vi "Data Analysis.vi"(1 "Data IN":T1={"Impulse Positions"=[], "No. Imp"=0, "Parameter Time Series"=[], "Parameter Impuls Series"=[], "Experiment Parameters"={"Freq"=0.0, "Vel"=0, "Acc"=0, "Stimulus"=""}, "Autosort File"=refnum, "Data File"={"Data Channels"=[], "Sample Rate"=0, "Channel List"=[]}, "Experiment data path"=path "/Macintosh HD/Users/patrick/Studium/Diploma Thesis/Data Analysis", "Image data path"=path "/Macintosh HD/Users/patrick/Studium/Diploma Thesis/Data Analysis", "LVS data path"=path "/Macintosh HD/Users/patrick/Studium/Diploma Thesis/Data Analysis", "Raw copy path"=path "/Macintosh HD/Users/patrick/Studium/Diploma Thesis/Data Analysis", "filename"="No file selected", "desaccading parameters"={"Tolerance"=0, "Acc Range"=0.0, "Sample Rate"=0, "Impulse Plane 2"=enum."Other", "Impulse dir"=FALSE}, "Experiment Parameters 2"={"Subject"="", "Strain"="", "Rotation plane"="", "Experimenter"="", "Trial"=0.0, "Time"=0.0}, "Excel"={"Excel._Application"=refnum, "Use Excel"=FALSE, "Worksheet SINE"=refnum, "Row SINE"=0, "Worksheet TRANS"=refnum, "Row TRANS"=0}, "Session Config File"=refnum, "Autosort Parameter Set"=1, "EMA Version"="", "desacc "={"Threshold 1 [Acc]"=1617.080808080808, "Threshold 2 [% of TH1]"=67, "tolerance"=5, "Search WD "=0.19090909090909092, " always use TH2"=TRUE, "Range"=3.2323232323232323, "Max time"=200.0, "Min time"=20.0, "Velocity Threshold"=67}, "Cycle Nr for Saccades"={"POS"=0, "NEG"=0}, "calibration name"="No file selected", "Excel"=refnum} {"Parameter Time Series"."time offset" format="%.3f"; "Parameter Time Series"."Gain" format="%.1f"; "Parameter Time Series"."Offset" format="%.1f"; "Parameter Time Series"."List 1" items=["Motor-Pos", "Motor-Vel", "Lx Position-in-Head", "Ly Position-in-Head", "Lz Position-in-Head", "Lx Velocity-in-Head", "Ly Velocity-in-Head", "Lz Velocity-in-Head", "Ll Velocity-in-Head", "Lr Velocity-in-Head", "Lx Accel-in-Head", "Ly Accel-in-Head", "Lz Accel-in-Head", "Rx Position-in-Head", "Ry Position-in-Head", "Rz Position-in-Head", "Rx Velocity-in-Head", "Ry Velocity-in-Head", "Rz Velocity-in-Head", "Rl Velocity-in-Head", "Rr Velocity-in-Head", "Rx Accel-in-Head", "Ry Accel-in-Head", "Rz Accel-in-Head", "Global Trigger", "", "", ""]; "Parameter Impuls Series"."Gain" format="%.1f"; "Parameter Impuls Series"."Offset" format="%.1f"}, 9 "Trace Select":i32 min=0 max=1000, 11 "Interpolate":bool) -> (3 "Data OUT":T1={"Impulse Positions"=[], "No. Imp"=0, "Parameter Time Series"=[], "Parameter Impuls Series"=[], "Experiment Parameters"={"Freq"=0.0, "Vel"=0, "Acc"=0, "Stimulus"=""}, "Autosort File"=refnum, "Data File"={"Data Channels"=[], "Sample Rate"=0, "Channel List"=[]}, "Experiment data path"=path "/Macintosh HD/Users/patrick/Studium/Diploma Thesis/Data Analysis", "Image data path"=path "/Macintosh HD/Users/patrick/Studium/Diploma Thesis/Data Analysis", "LVS data path"=path "/Macintosh HD/Users/patrick/Studium/Diploma Thesis/Data Analysis", "Raw copy path"=path "/Macintosh HD/Users/patrick/Studium/Diploma Thesis/Data Analysis", "filename"="No file selected", "desaccading parameters"={"Tolerance"=0, "Acc Range"=0.0, "Sample Rate"=0, "Impulse Plane 2"=enum."Other", "Impulse dir"=FALSE}, "Experiment Parameters 2"={"Subject"="", "Strain"="", "Rotation plane"="", "Experimenter"="", "Trial"=0.0, "Time"=0.0}, "Excel"={"Excel._Application"=refnum, "Use Excel"=FALSE, "Worksheet SINE"=refnum, "Row SINE"=0, "Worksheet TRANS"=refnum, "Row TRANS"=0}, "Session Config File"=refnum, "Autosort Parameter Set"=1, "EMA Version"="", "desacc "={"Threshold 1 [Acc]"=1617.080808080808, "Threshold 2 [% of TH1]"=67, "tolerance"=5, "Search WD "=0.19090909090909092, " always use TH2"=TRUE, "Range"=3.2323232323232323, "Max time"=200.0, "Min time"=20.0, "Velocity Threshold"=67}, "Cycle Nr for Saccades"={"POS"=0, "NEG"=0}, "calibration name"="No file selected", "Excel"=refnum} {"Parameter Time Series"."time offset" format="%.3f"; "Parameter Time Series"."Gain" format="%.1f"; "Parameter Time Series"."Offset" format="%.1f"; "Parameter Time Series"."List 1" items=["Motor-Pos", "Motor-Vel", "Lx Position-in-Head", "Ly Position-in-Head", "Lz Position-in-Head", "Lx Velocity-in-Head", "Ly Velocity-in-Head", "Lz Velocity-in-Head", "Ll Velocity-in-Head", "Lr Velocity-in-Head", "Lx Accel-in-Head", "Ly Accel-in-Head", "Lz Accel-in-Head", "Rx Position-in-Head", "Ry Position-in-Head", "Rz Position-in-Head", "Rx Velocity-in-Head", "Ry Velocity-in-Head", "Rz Velocity-in-Head", "Rl Velocity-in-Head", "Rr Velocity-in-Head", "Rx Accel-in-Head", "Ry Accel-in-Head", "Rz Accel-in-Head", "Global Trigger", "", "", ""]; "Parameter Impuls Series"."Gain" format="%.1f"; "Parameter Impuls Series"."Offset" format="%.1f"})   [LabVIEW 2016]
uses:
  Typedef - Sinusoidal Fit Controls.ctl
  Typedef - Sinusoidal Fit Coefficients.ctl
  Typedef_StatisticType.ctl
  Typedef - Gain and Phase.ctl
  core/type-defs/TD_Statemachine-Data.ctl
  <userlib>/Import Export/Excel/Excel.lvclass
  core/type-defs/TD_Time Series.ctl
  core/type-defs/TD_Impulse Parameter.ctl
  Typedef - Type of Analysis.ctl
  core/Classes/Exponential Fit/Exponential Fit Parameters.ctl
  core/Classes/Head Impulse Fit/Fit Data.ctl
  core/Classes/Head Impulse Fit/Fit Controls.ctl
  Data Analysis state.ctl
  Typedef - Data Analyser Main Cluster.ctl
  core/Classes/Impulse Data/Instance handle.ctl
  core/Classes/Impulse Data/Impulse Data.lvclass
  core/Classes/Impulse Manager/Impulse Manager.lvclass
  core/Classes/Graph Manager/Graph Manager.lvclass
  core/Classes/Sinusoidal Fit/Sinusoidal Fit.lvclass
  C:/Users/w.figtree/Desktop/Work/4. Projects/3. In Progress Engineering Projects/EMA/src/core/Classes/Abstract Fit/Abstract Fit.lvclass
  core/Classes/Excel Logger/Excel Logger.lvclass
  core/Classes/Fit Displays/Halfwave Fit Display/Halfwave Fit Display.lvclass
  core/Classes/Mean Fit/Mean Fit.lvclass
  core/Classes/Exponential Fit/Exponential Fit.lvclass
  core/Classes/Head Impulse Fit/Head Impulse Fit.lvclass
  core/Classes/Desaccade Manipulator/Desaccade Manipulator.lvclass
  core/Classes/Excel Logger/Excel Logger.lvclass/Excel Logger.ctl
  core/type-defs/TD_Impulse Planes.ctl
  core/Classes/Abstract Fit/Abstract Fit.lvclass/Abstract Fit.ctl
  core/Classes/Sinusoidal Fit/Sinusoidal Fit.lvclass/Sinusoidal Fit.ctl
  <vilib>/Analysis/baseanly.llb/Mean (DBL).vi
  core/Classes/Data Analyser Report/Data Analyser Report.lvclass
  C:/Users/w.figtree/Desktop/Work/4. Projects/3. In Progress Engineering Projects/EMA/src/core/Classes/Excel Interface/Excel Sheet/Excel Sheet.lvclass
  core/Classes/Sinusoidal Fit/Halfwave Sinusoidal Fit/Halfwave Sinusoidal Fit.lvclass
  C:/Users/w.figtree/Desktop/Work/4. Projects/3. In Progress Engineering Projects/EMA/src/core/Classes/Sinusoidal Fit/Sinusoidal Fit.lvclass
  core/Classes/Excel Interface/Excel Sheet/Write to Cell - String.vi
  core/Classes/Excel Interface/Excel Sheet/Write to Cell - Int.vi
  core/Classes/Excel Interface/Excel Sheet/Write to Cell - Dbl.vi
  <userlib>/_OpenG.lib/array/array.llb/Remove Duplicates from 1D Array (I32)__ogtk.vi
  comm/impulse/impulse functions.lvlib
  comm/nan operations/nan operations.lvlib
  comm/stats/stats.lvlib
  <vilib>/Analysis/NI_AALPro.lvlib
  comm/excel/excel.lvlib
  <vilib>/Analysis/NI_AALBase.lvlib
  core/core.lvlib
  core/Classes/Excel Interface/Excel Sheet/Excel Sheet.lvclass
  core/Classes/Abstract Fit/Abstract Fit.lvclass
panel:
  out "Impulse Trace":cluster{dbl, dbl, "Impulses":dbl[][]}(graph)
  in  "Response":dbl[](array[numeric]) format="%.2f"
  in  "Stimulus":dbl[](array[numeric]) format="%.2f"
  in  "Reset view":bool
  in  "Show Fit":bool=TRUE
  in  "Mean Traces":bool=TRUE
  in  "Fixed Time":bool
  in  "Fixed Amplitude":bool
  in  "Interpolate 3":bool
  in  "Interpolate 2":bool
  in  "Gv Line Fit Response":cluster{"Offset":dbl, "Slope":dbl}={"Offset"=186.60289859552654, "Slope"=-3505.824046527282} {"Slope" format="%.2f"; "Offset" format="%.2f"}
  in  "Gv Line Fit Stimulus":cluster{"Offset":dbl, "Slope":dbl}={"Offset"=195.7972297018837, "Slope"=-3976.499768980883} {"Slope" format="%.2f"; "Offset" format="%.2f"}
  in  "Fitted Curves":dbl[][](array[numeric]) format="%.2f"
  in  "Tab Control":T4(tab)
  in  "Sinusoidal Fit Controls":T5={"Sinusoidal Response"={"Offset"=-0.14811303182601265, "Gain"=36.1562775012231, "Phase"=51.14206032808873, "Freq"=8.0}, "Sinusoidal Stimulus"={"Offset"=-0.1762531244084861, "Gain"=54.01231242273056, "Phase"=48.997269246957444, "Freq"=8.0}, "Stimulus\nFrequency"=8.0, "Stat."=enum."Ind. Traces", "Use Values Above to Calculate Gains"=FALSE, "Automatically Calculate \nStimulus Frequency"=FALSE, "Gain and Phase"={"Gain"=0.0, "Gain SD"=0.0, "Phase"=0.0, "Phase SD"=0.0}} {"Gain and Phase"."Phase SD" format="%.1f"; "Gain and Phase"."Phase" format="%.1f"; "Gain and Phase"."Gain SD" format="%.2f"; "Gain and Phase"."Gain" format="%.2f"; "Stimulus\nFrequency" format="%.2f"; "Sinusoidal Stimulus"."Freq" format="%#.2f"; "Sinusoidal Stimulus"."Offset" format="%.3f"; "Sinusoidal Stimulus"."Gain" format="%.2f"; "Sinusoidal Stimulus"."Phase" format="%.1f"; "Sinusoidal Response"."Freq" format="%#.2f"; "Sinusoidal Response"."Offset" format="%.3f"; "Sinusoidal Response"."Gain" format="%.2f"; "Sinusoidal Response"."Phase" format="%.1f"}
  in  "Transient Gains":T9={"Line Fit Response"={"Offset"=186.60289859552654, "Slope"=-3505.824046527282}, "Stimulus Equation"="195.80  + -3976.50 t ", "Reponse Equation"="186.60  + -3505.82 t ", "Gv"=-0.4707337082056428, "Ga"=0.8816409948711299, "Line Fit Stimulus"={"Offset"=195.7972297018837, "Slope"=-3976.499768980883}, "Ga Window (early)"=0, "Gv Window"=1, "Latency (ms)"=3.987957239637936, "Stim.Onset"=49.23858696766971, "TH/#SDs 2"=10.0, "Response Onset"=53.22654420730765, "Snap Cursor"=1, "Latency"=2, "Poly. Window"=1, "Ord."=3, "BIC"=3.7869704994038274, "Poly Equation"="124.42 t^0 + -1322.54 t^1 + -147215.26 t^2 + 1663449.30 t^3", "Gv SD"=1.2509198071254501, "Ga SD"=0.09245681991197086, "Ga Stat."=0, "Mirror"=FALSE, "MSE"=3.7869704994038274, "Gv Stat."=2, "Ga 2"=0.8816409948711299, "Ga SD 2"=0.09245681991197086, "Ga Window  (late)"=5, "Ga Stat. 2"=0, "GV desaccading"=TRUE, "GA2 desaccading"=FALSE, "GA1 desaccading"=FALSE, "Line Fit Response 2"={"Offset"=186.60289859552654, "Slope"=-3505.824046527282}, "Stimulus Equation 2"="195.80  + -3976.50 t ", "Reponse Equation 2"="186.60  + -3505.82 t ", "Line Fit Stimulus 2"={"Offset"=195.7972297018837, "Slope"=-3976.499768980883}, "Show Line Fit Parameters "=FALSE, "Gv Line Fit Stimulus"={"Offset"=195.7972297018837, "Slope"=-3976.499768980883}, "Gv Line Fit Response"={"Offset"=186.60289859552654, "Slope"=-3505.824046527282}, "Latency window"=0, "Latency Stat."=0, "Line Fit Res Latency"={"Offset"=186.60289859552654, "Slope"=-3505.824046527282}, "Stim Eq Latency"="195.80  + -3976.50 t ", "Resp Eq Latency"="186.60  + -3505.82 t ", "Line Fit Stim Latency"={"Offset"=195.7972297018837, "Slope"=-3976.499768980883}, "GA Line active"=0} {"Line Fit Stim Latency"."Slope" format="%.2f"; "Line Fit Stim Latency"."Offset" format="%.2f"; "Line Fit Res Latency"."Slope" format="%.2f"; "Line Fit Res Latency"."Offset" format="%.2f"; "Latency Stat." items=["Mean Trace", "Ind. Traces", "Pnt. by Pnt.", "Inst. Slope"]; "Latency window" items=["Cursor", "10 - 20 ms", "20 - 30 ms", "30 - 40 ms", "40 - 50 ms", "20 - 40 ms", "10 - 30 ms"]; "Latency" items=["Standard Dev.", "Threshold", "Line Intercept"]; "TH/#SDs 2" format="%.2f"; "Stim.Onset" format="%.2f"; "Latency (ms)" format="%.2f"; "MSE" format="%.4f"; "BIC" format="%.2f"; "Poly. Window" items=["Cursor", "10 - 40 ms", "5 - 35 ms", "0 - 30 ms"]; "Ga Stat." items=["Mean Trace", "Ind. Traces", "Pnt. by Pnt.", "Inst. Slope"]; "Ga SD" format="%.2f"; "Ga Window (early)" items=["Cursor", "10 - 20 ms", "20 - 30 ms", "30 - 40 ms", "40 - 50 ms", "20 - 40 ms", "10 - 30 ms"]; "Ga" format="%.2f"; "Ga Stat. 2" items=["Mean Trace", "Ind. Traces", "Pnt. by Pnt.", "Inst. Slope"]; "Ga Window  (late)" items=["Cursor", "10 - 20 ms", "20 - 30 ms", "30 - 40 ms", "40 - 50 ms", "20 - 40 ms", "10 - 30 ms"]; "Ga SD 2" format="%.2f"; "Ga 2" format="%.2f"; "Gv Stat." items=["Mean Trace", "Ind. Traces", "Pnt. by Pnt.", "Inst. Slope"]; "Gv SD" format="%.2f"; "Gv Window" items=["Cursor", "200 - 400ms", "200 - 700ms"]; "Gv" format="%.2f"; "Snap Cursor" items=["No Snap", "to Ga (early)", "to Ga (late)", "to Gv", "Latency"]; "Gv Line Fit Response"."Slope" format="%.2f"; "Gv Line Fit Response"."Offset" format="%.2f"; "Gv Line Fit Stimulus"."Slope" format="%.2f"; "Gv Line Fit Stimulus"."Offset" format="%.2f"; "Line Fit Stimulus 2"."Slope" format="%.2f"; "Line Fit Stimulus 2"."Offset" format="%.2f"; "Line Fit Response 2"."Slope" format="%.2f"; "Line Fit Response 2"."Offset" format="%.2f"; "Response Onset" format="%.2f"; "Line Fit Stimulus"."Slope" format="%.2f"; "Line Fit Stimulus"."Offset" format="%.2f"; "Line Fit Response"."Slope" format="%.2f"; "Line Fit Response"."Offset" format="%.2f"}
  in  "Tab Control 2":enum32{"Page 1", "Page 2"}(tab)
  in  "Save All G&P To Excel":bool
  out "Normal Sine - Gain and Phase":T8 caption="Gain and Phase" {"Phase SD" format="%.1f"; "Phase" format="%.1f"; "Gain SD" format="%.2f"; "Gain" format="%.2f"}
  out "Normal Sine - Stimulus":T6 caption="Stimulus" {"Freq" format="%#.2f"; "Offset" format="%.3f"; "Gain" format="%.2f"; "Phase" format="%.1f"}
  in  "Normal Sine - Response":T6 caption="Response" {"Freq" format="%#.2f"; "Offset" format="%.3f"; "Gain" format="%.2f"; "Phase" format="%.1f"}
  out "Positive Halfwave":T8 {"Phase SD" format="%.1f"; "Phase" format="%.1f"; "Gain SD" format="%.2f"; "Gain" format="%.2f"}
  out "Negative Halfwave":T8 {"Phase SD" format="%.1f"; "Phase" format="%.1f"; "Gain SD" format="%.2f"; "Gain" format="%.2f"}
  out "Coefficients":T6 {"Freq" format="%#.2f"; "Offset" format="%.3f"; "Gain" format="%.2f"; "Phase" format="%.1f"}
  in  "Pos HW Response":T6 caption="Response" {"Freq" format="%#.2f"; "Offset" format="%.3f"; "Gain" format="%.2f"; "Phase" format="%.1f"}
  out "Coefficients 2":T6 {"Freq" format="%#.2f"; "Offset" format="%.3f"; "Gain" format="%.2f"; "Phase" format="%.1f"}
  in  "Neg HW Response":T6 {"Freq" format="%#.2f"; "Offset" format="%.3f"; "Gain" format="%.2f"; "Phase" format="%.1f"}
  in  "Auto Calc.":bool
  in  "Stimulus\nFrequency":dbl=8.0 format="%.2f"
  in  "Sine Fit Type":enum16{"Normal Fit", "Halfwave Fit"}(ring)
  in  "Stat. Method":T7=enum."Ind. Traces"
  in  "Offset":dbl format="%#_13g"
  in  "Mean Stats Method":T7=enum."Ind. Traces" caption="Statistics Method"
  out "Mean Fit":T10
  in  "Exp Response":T11 caption="Response Fit Parameters"
  in  "Exp Stimulus":T11 caption="Stimulus Fit Parameters"
  in  "Head Impulse Fit Controls":T12={"Pre-peak-ms"=30.0, "Onset threshold (%)"=4.0, "Window size (+- ms)"=10.0, "Window Centres\n(ms after onset)"=[40.0, 60.0, 80.0]}
  out "Head Impulse Fit Data":T13 {"Window Eye Lag (ms)" format="%#_4g"; "Window Gain" format="%#_4g"}
  in  "btn_SaveImpulseLatency":bool
  out "Impulse Latency Summary":T14
  in  "Impulse Latency Controls":T15={"Peak%"=4.0, "Min Valid Latency"=-50.0, "Max Valid Latency"=50.0, "Only After\nCursor?"=TRUE}
  out "Impulse Latency Results":dbl[][](array[numeric])
  in  "Excel Cell Handling":enum16{"Active Cell", "First empty cell (Ax)"}(ring)=enum."First empty cell (Ax)"
  in  "Freeze Visibility On Channel Cycle":bool
  in  "Auto Channel Cycle":bool
  in  "Prefer Mean Fit":bool
  in  "Limit Phase to 180 degrees (negative gains!)":bool
  in  "Hide Grid":bool
  in  "Hide Cursors":bool
  in  "Parameters":T16={"Vel Range"=10.0, "Acc Range"=500.0, "Stimulus Freq"=4.0, "Impulse Plane"=enum."Other", "Impulse Direction"=TRUE} {"Stimulus Freq" step=0.5 format="%.2f"; "Acc Range" format="%.2f"; "Vel Range" format="%.2f"}
  in  "Line Range +/- GV":dbl=0.2
  in  "Line Range +/- GA":dbl=0.06
  in  "Spline Parameter":dbl=0.999
  in  "Spline":bool
  in  "Type of Analysis":T17
  in  "Save 2 Excel":bool
  in  "Save":bool
  in  "Analyse Data":bool
  in  "Impulse Direction":bool=TRUE
  in  "Cycle  Channel":bool
  in  "Parameter Impuls Series":T3=[{"Color"=4652800, "Visible"=TRUE, "Channel"=5, "Invert"=FALSE, "Desaccade"=FALSE, "Offset"=0.0, "Gain"=1.0}, {"Color"=16860, "Visible"=TRUE, "Channel"=13, "Invert"=FALSE, "Desaccade"=FALSE, "Offset"=0.0, "Gain"=1.0}, {"Color"=16711680, "Visible"=TRUE, "Channel"=21, "Invert"=FALSE, "Desaccade"=FALSE, "Offset"=0.0, "Gain"=1.0}] {"Gain" format="%.1f"; "Offset" format="%.1f"; "Channel" items=["-", "Hz Velocity-in-Head", "-", "Hy Velocity-in-Head", "-", "Hx Velocity-in-Head", "Hl Velocity-in-Head", "Hr Velocity-in-Head", "-", "Ly Position-in-Head", "Lz Position-in-Head", "-", "Ly Velocity-in-Head", "Lz Velocity-in-Head", "-", "Hx Acceleration-in-Head", "Hy Acceleration-in-Head", "Hz Acceleration-in-Head", "Hl Acceleration-in-Head", "Hr Acceleration-in-Head", "-", "Ly Acceleration-in-Head", "Lz Acceleration-in-Head", "-"]}
  in  "Generate New Plot":bool
  # "Gain:"
  # "+/-"
  # "Phase:"
  # "+/-"
  # "Latency"
  # "Polynomial Fit"
  # "Regression Fit"
  # "Desacc."
  # "Gain:"
  # "+/-"
  # "Phase:"
  # "+/-"
  # "Gain:"
  # "+/-"
  # "Phase:"
  # "+/-"
  # "Gain:"
  # "+/-"
  # "Phase:"
  # "+/-"
  # "Fit Controls"
  # "Stimulus"
  # "Response"
  # "EXPERIMENTAL - DO NOT USE"
  # "NOTE: Response must be inverted!"
  # "Desaccading Parameters"
  # "Pos"
  # "Neg"
  # "Latency, Gain and Phase Detector \nver 3.0\nAmerico A. Migliaccio and Patrick P. Huebner\n13th May 2010"
  # "Analysis"
  # "Offset      Gain    Inv                    Channel                      Col   Vis   Sac"
  # "Stimulus"
  # "Response"
  # "Additional\n|\n\\/"
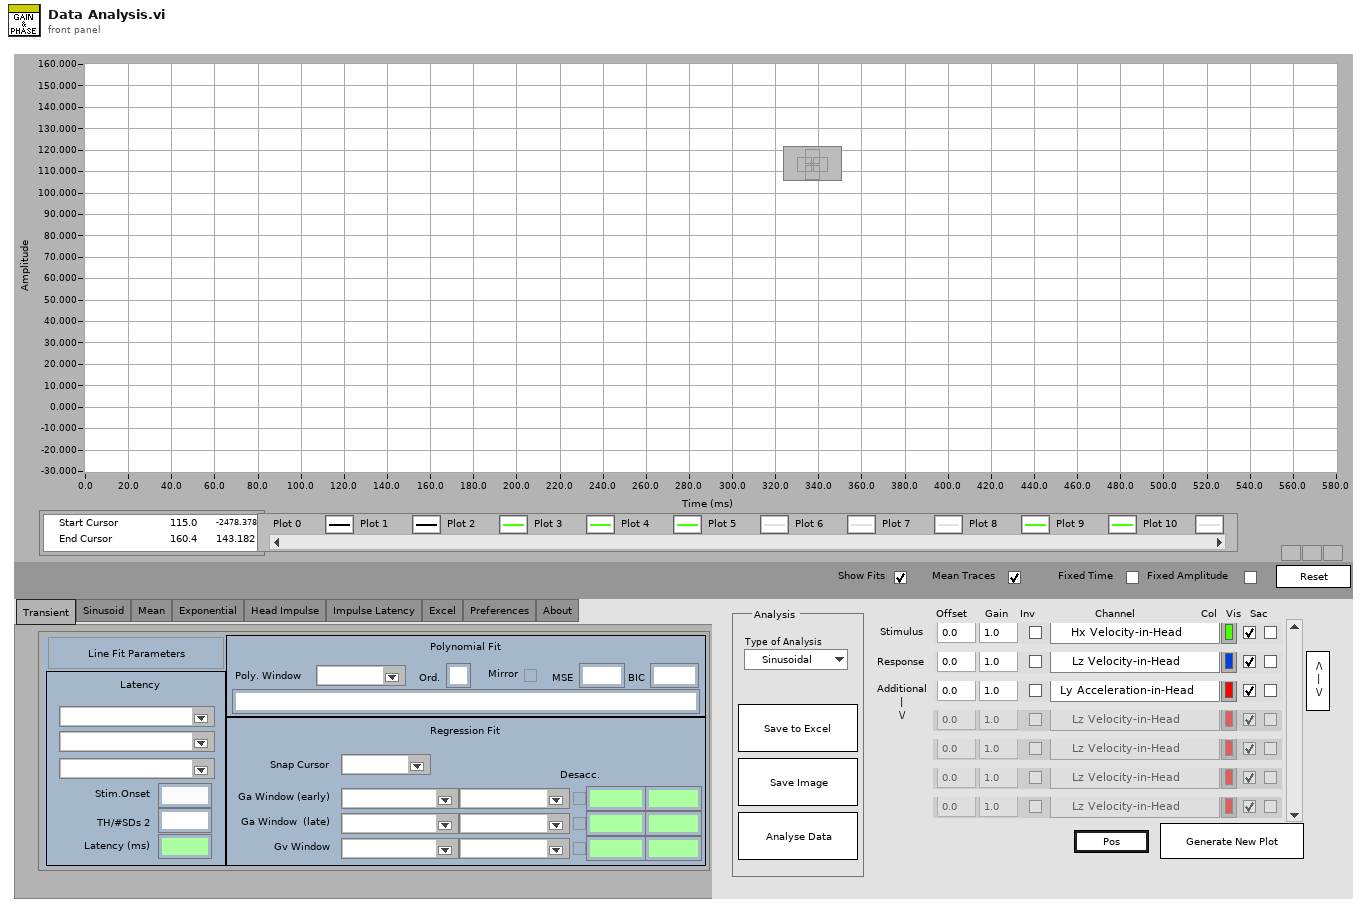
[diagram p1: front panel]
types:
  T1 = typedef "core.lvlib/TD_Statemachine-Data.ctl" = cluster{"Impulse Positions":cluster{"Start":i32, "End":i32, "Impulse Plane":enum16{"Other", "Yaw", "Pitch", "Roll", "LARP", "RALP"}, "Impulse Direction +ve?":bool, "Time offset":i32, "Amplitude offset":dbl}[], "No. Imp":i32, "Parameter Time Series":T2, "Parameter Impuls Series":T3, "Experiment Parameters":cluster{"Freq":dbl, "Vel":i32, "Acc":i32, "Stimulus":string}, "Autosort File":refnum<file>, "Data File":cluster{"Data Channels":dbl[][], "Sample Rate":i32, "Channel List":string[]}, "Experiment data path":path, "Image data path":path, "LVS data path":path, "Raw copy path":path, "filename":string, "desaccading parameters":cluster{"Tolerance":i32, "Acc Range":dbl, "Sample Rate":i32, "Impulse Plane 2":enum16{"Other", "Yaw", "Pitch", "Roll", "LARP", "RALP"}, "Impulse dir":bool}, "Experiment Parameters 2":cluster{"Subject":string, "Strain":string, "Rotation plane":string, "Experimenter":string, "Trial":dbl, "Time":dbl}, "Excel":cluster{"Excel._Application":refnum<k7>, "Use Excel":bool, "Worksheet SINE":refnum<k7>, "Row SINE":i32, "Worksheet TRANS":refnum<k7>, "Row TRANS":i32}, "Session Config File":refnum<file>, "Autosort Parameter Set":i32, "EMA Version":string, "desacc ":cluster{"Threshold 1 [Acc]":dbl, "Threshold 2 [% of TH1]":i32, "tolerance":i32, "Search WD ":dbl, " always use TH2":bool, "Range":dbl, "Max time":dbl, "Min time":dbl, "Velocity Threshold":i32}, "Cycle Nr for Saccades":cluster{"POS":i32, "NEG":i32}, "calibration name":string, "Excel":refnum<class "Excel.lvclass">}
  T2 = typedef "core.lvlib/TD_Time Series.ctl" = cluster{"time offset":dbl, "Offset":dbl, "Gain":dbl, "inverse":bool, "filter data":bool, "dots":bool, "interpolate":bool, "List 1":u16, "Color Box":u32, "Boolean":bool}[]
  T3 = typedef "core.lvlib/TD_Impulse Parameter.ctl" = cluster{"Color":u32, "Visible":bool, "Channel":u16, "Invert":bool, "Desaccade":bool, "Offset":dbl, "Gain":dbl}[]
  T4 = enum32{"Transient", "Sinusoid", "Mean", "Exponential", "Head Impulse", "Impulse Latency", "Excel", "Preferences", "About"}
  T5 = typedef "Typedef - Sinusoidal Fit Controls.ctl" = cluster{"Sinusoidal Response":T6, "Sinusoidal Stimulus":T6, "Stimulus\nFrequency":dbl, "Stat.":T7, "Use Values Above to Calculate Gains":bool, "Automatically Calculate \nStimulus Frequency":bool, "Gain and Phase":T8}
  T6 = typedef "Typedef - Sinusoidal Fit Coefficients.ctl" = cluster{"Offset":dbl, "Gain":dbl, "Phase":dbl, "Freq":dbl}
  T7 = typedef "Typedef_StatisticType.ctl" = enum16{"Mean Trace", "Ind. Traces"}
  T8 = typedef "Typedef - Gain and Phase.ctl" = cluster{"Gain":dbl, "Gain SD":dbl, "Phase":dbl, "Phase SD":dbl}
  T9 = cluster{"Line Fit Response":cluster{"Offset":dbl, "Slope":dbl}, "Stimulus Equation":string, "Reponse Equation":string, "Gv":dbl, "Ga":dbl, "Line Fit Stimulus":cluster{"Offset":dbl, "Slope":dbl}, "Ga Window (early)":u16, "Gv Window":u16, "Latency (ms)":dbl, "Stim.Onset":dbl, "TH/#SDs 2":dbl, "Response Onset":dbl, "Snap Cursor":u16, "Latency":u16, "Poly. Window":u16, "Ord.":i32, "BIC":dbl, "Poly Equation":string, "Gv SD":dbl, "Ga SD":dbl, "Ga Stat.":u16, "Mirror":bool, "MSE":dbl, "Gv Stat.":u16, "Ga 2":dbl, "Ga SD 2":dbl, "Ga Window  (late)":u16, "Ga Stat. 2":u16, "GV desaccading":bool, "GA2 desaccading":bool, "GA1 desaccading":bool, "Line Fit Response 2":cluster{"Offset":dbl, "Slope":dbl}, "Stimulus Equation 2":string, "Reponse Equation 2":string, "Line Fit Stimulus 2":cluster{"Offset":dbl, "Slope":dbl}, "Show Line Fit Parameters ":bool, "Gv Line Fit Stimulus":cluster{"Offset":dbl, "Slope":dbl}, "Gv Line Fit Response":cluster{"Offset":dbl, "Slope":dbl}, "Latency window":u16, "Latency Stat.":u16, "Line Fit Res Latency":cluster{"Offset":dbl, "Slope":dbl}, "Stim Eq Latency":string, "Resp Eq Latency":string, "Line Fit Stim Latency":cluster{"Offset":dbl, "Slope":dbl}, "GA Line active":i32}
  T10 = cluster{"Respopnse Mean":dbl, "Response SD":dbl, "Stimulus Mean":dbl, "Stimulus SD":dbl}
  T11 = typedef "Exponential Fit.lvclass/Exponential Fit Parameters.ctl" = cluster{"Amplitude":dbl, "Duration":dbl, "Time Constant":dbl, "Offset":dbl}
  T12 = typedef "Head Impulse Fit.lvclass/Fit Controls.ctl" = cluster{"Pre-peak-ms":dbl, "Onset threshold (%)":dbl, "Window size (+- ms)":dbl, "Window Centres\n(ms after onset)":dbl[]}
  T13 = typedef "Head Impulse Fit.lvclass/Fit Data.ctl" = cluster{"Peak time (ms)":dbl, "Peak val":dbl, "Gain":dbl, "Gain SD":dbl, "Peak-Peak lag (ms)":dbl, "Peak-Peak lag SD":dbl, "Window Gain":dbl[][], "Window Eye Lag (ms)":dbl[][]}
  T14 = cluster{"Stimulus Onset (ms)":dbl, "Response Onset (ms)":dbl, "Latency (ms)":dbl, "Num Impulses":dbl}
  T15 = cluster{"Peak%":dbl, "Min Valid Latency":dbl, "Max Valid Latency":dbl, "Only After\nCursor?":bool}
  T16 = cluster{"Vel Range":dbl, "Acc Range":dbl, "Stimulus Freq":dbl, "Impulse Plane":enum16{"Other", "Yaw", "Pitch", "Roll", "LARP", "RALP"}, "Impulse Direction":bool}
  T17 = typedef "Typedef - Type of Analysis.ctl" = enum16{"Sinusoidal", "Transient", "Mean", "Exponential", "Head Impulse", "Impulse Latency"}
  T18 = typedef "Typedef - Data Analyser Main Cluster.ctl" = cluster{"Impulse Positions":cluster{"Start":i32, "End":i32, "Impulse Plane":enum16{"Other", "Yaw", "Pitch", "Roll", "LARP", "RALP"}, "Impulse Direction +ve?":bool, "Time offset":i32, "Amplitude offset":dbl}[], "Data File":cluster{"Data Channels":dbl[][], "Sample Rate":i32, "Channel List":string[]}, "desaccading parameters":cluster{"Tolerance":i32, "Acc Range":dbl, "Sample Rate":i32, "Impulse Plane 2":enum16{"Other", "Yaw", "Pitch", "Roll", "LARP", "RALP"}, "Impulse dir":bool}, "Stimulus":dbl[], "Response":dbl[], "Fitted Curves":dbl[][], "Sinusoidal Fit Controls":T5, "Transient Gains":cluster{"Line Fit Response":cluster{"Offset":dbl, "Slope":dbl}, "Stimulus Equation":string, "Reponse Equation":string, "Gv":dbl, "Ga":dbl, "Line Fit Stimulus":cluster{"Offset":dbl, "Slope":dbl}, "Ga Window (early)":u16, "Gv Window":u16, "Latency (ms)":dbl, "Stim.Onset":dbl, "TH/#SDs 2":dbl, "Response Onset":dbl, "Snap Cursor":u16, "Latency":u16, "Poly. Window":u16, "Ord.":i32, "BIC":dbl, "Poly Equation":string, "Gv SD":dbl, "Ga SD":dbl, "Ga Stat.":u16, "Mirror":bool, "MSE":dbl, "Gv Stat.":u16, "Ga 2":dbl, "Ga SD 2":dbl, "Ga Window  (late)":u16, "Ga Stat. 2":u16, "GV desaccading":bool, "GA2 desaccading":bool, "GA1 desaccading":bool, "Line Fit Response 2":cluster{"Offset":dbl, "Slope":dbl}, "Stimulus Equation 2":string, "Reponse Equation 2":string, "Line Fit Stimulus 2":cluster{"Offset":dbl, "Slope":dbl}, "Show Line Fit Parameters ":bool, "Gv Line Fit Stimulus":cluster{"Offset":dbl, "Slope":dbl}, "Gv Line Fit Response":cluster{"Offset":dbl, "Slope":dbl}, "Latency window":u16, "Latency Stat.":u16, "Line Fit Res Latency":cluster{"Offset":dbl, "Slope":dbl}, "Stim Eq Latency":string, "Resp Eq Latency":string, "Line Fit Stim Latency":cluster{"Offset":dbl, "Slope":dbl}, "GA Line active":i32}, "Gv Line Fit Stimulus":cluster{"Offset":dbl, "Slope":dbl}, "Gv Line Fit Response":cluster{"Offset":dbl, "Slope":dbl}, "Fit Calculated":bool, "Excel":cluster{"Excel._Application":refnum<k7>, "Use Excel":bool, "Worksheet SINE":refnum<k7>, "Row SINE":i32, "Worksheet TRANS":refnum<k7>, "Row TRANS":i32}, "desacc ":cluster{"Threshold 1 [Acc]":dbl, "Threshold 2 [% of TH1]":i32, "tolerance":i32, "Search WD ":dbl, " always use TH2":bool, "Range":dbl, "Max time":dbl, "Min time":dbl, "Velocity Threshold":i32}, "Impulse Data":T19, "Impulse Manager":refnum<class "Impulse Manager.lvclass">, "Graph Manager":refnum<class "Graph Manager.lvclass">, "Sine Fit":refnum<class "Sinusoidal Fit.lvclass">[], "Excel Logger":refnum<class "Excel Logger.lvclass">, "Halfwave Fit Display":refnum<class "Halfwave Fit Display.lvclass">, "Mean Fit":refnum<class "Mean Fit.lvclass">, "Exponential Fit":refnum<class "Exponential Fit.lvclass">, "HI Fit":refnum<class "Head Impulse Fit.lvclass">}
  T19 = typedef "Impulse Data.lvclass/Instance handle.ctl" = refnum<data-value>
  T20 = typedef "Data Analysis state.ctl" = enum16{"Quit", "Cycle Channels", "Generate Plot", "Analyse Data", "Save Image", "Polynomial Fit", "Open_Create Excel", "Excel find free A cell", "Panel Monitoring", "Save to Excel", "Initialize", "Extract Data", "Display Data", "Calculate Sinusoidal Gains", "Make Transient Fits & Equations", "Calculate Latency Fits", "Calculate Transient Ga 1 Gain", "Calculate Transient Ga 2 Gain", "Calculate Transient Gv Gain", "Stop", "Calculate Latency", "Calculate Exponential", "Calculate Mean", "Calculate Head Impulse", "Update controls and variables", "Save All Gain And Phase To Excel", "Calculate Impulse Latency", "Save Impulse Latency To Excel"}
  T21 = enum8{"solid", "dashed long", "dashed short", "dot dashed"}
  T22 = cluster{"Tolerance":i32, "Acc Range":dbl, "Sample Rate":i32, "Impulse Plane 2":enum16{"Other", "Yaw", "Pitch", "Roll", "LARP", "RALP"}, "Impulse dir":bool}
  T23 = typedef "eventvkey.ctl" = enum16{"ASCII", "Enter", "Return", "Shift", "Ctrl", "Alt", "Cmd", "Opt", "Caps", "NumLock", "Clear", "Break", "Up", "Down", "Left", "Right", "Insert", "Delete", "Home", "End", "PageUp", "PageDown", "Escape", "Help", "Pause", "ScrollLock", "F1", "F2", "F3", "F4", "F5", "F6", "F7", "F8", "F9", "F10", "F11", "F12", "F13", "F14", "F15", "F16", "F17", "F18", "F19", "F20", "F21", "F22", "F23", "F24", "Play", "VolumeUp", "VolumeDown", "Mute", "Two Byte Char"}
  T24 = cluster{"Start":i32, "End":i32, "Impulse Plane":enum16{"Other", "Yaw", "Pitch", "Roll", "LARP", "RALP"}, "Impulse Direction +ve?":bool, "Time offset":i32, "Amplitude offset":dbl}[]
  T25 = cluster{"Data Channels":dbl[][], "Sample Rate":i32, "Channel List":string[]}
  T26 = cluster{"Excel._Application":refnum<k7>, "Use Excel":bool, "Worksheet SINE":refnum<k7>, "Row SINE":i32, "Worksheet TRANS":refnum<k7>, "Row TRANS":i32}
  T27 = cluster{"Threshold 1 [Acc]":dbl, "Threshold 2 [% of TH1]":i32, "tolerance":i32, "Search WD ":dbl, " always use TH2":bool, "Range":dbl, "Max time":dbl, "Min time":dbl, "Velocity Threshold":i32}
  T28 = enum16{"Other", "Yaw", "Pitch", "Roll", "LARP", "RALP"}
  T29 = cluster{"Subject":string, "Strain":string, "Rotation plane":string, "Experimenter":string, "Trial":dbl, "Time":dbl}
  T30 = cluster{"Freq":dbl, "Vel":i32, "Acc":i32, "Stimulus":string}
  T31 = cluster{"Color":u32, "Visible":bool, "Channel":u16, "Invert":bool, "Desaccade":bool, "Offset":dbl, "Gain":dbl}
  T32 = typedef "imagedata.ctl" = cluster{"image type":i32, "image depth":i32, "image":u8[], "mask":u8[], "colors":u32[], "Rectangle":cluster{"left":i16, "top":i16, "right":i16, "bottom":i16}}
  T33 = typedef "TD_Impulse Planes.ctl" = enum16{"Other", "Yaw", "Pitch", "Roll", "LARP", "RALP"}
  T34 = cluster{"Impulse Plane":T33, "Impulse Direction +ve?":bool, "Start":i32, "Duration":i32}[]
  T35 = typedef "LVCursorListTypeDef.ctl" = cluster{"Name":string, "Color":u32, "Style":u8, "Point Style":u8, "Name Visible":bool, "Allow Drag":bool, "Cursor Mode":u32, "Plot":i32, "Index":i32, "Position":cluster{"X":dbl, "Y":dbl}, "X Scale":u32, "Y Scale":u32, "Watch Plots":i32[], "Watch All Plots":bool, "Plot Area":i32, "Label Offset":cluster{"X":dbl, "Y":dbl}}[]
  T36 = cluster{"Name":string, "Color":u32, "Style":u8, "Point Style":u8, "Name Visible":bool, "Allow Drag":bool, "Cursor Mode":u32, "Plot":i32, "Index":i32, "Position":cluster{"X":dbl, "Y":dbl}, "X Scale":u32, "Y Scale":u32, "Watch Plots":i32[], "Watch All Plots":bool, "Plot Area":i32, "Label Offset":cluster{"X":dbl, "Y":dbl}}
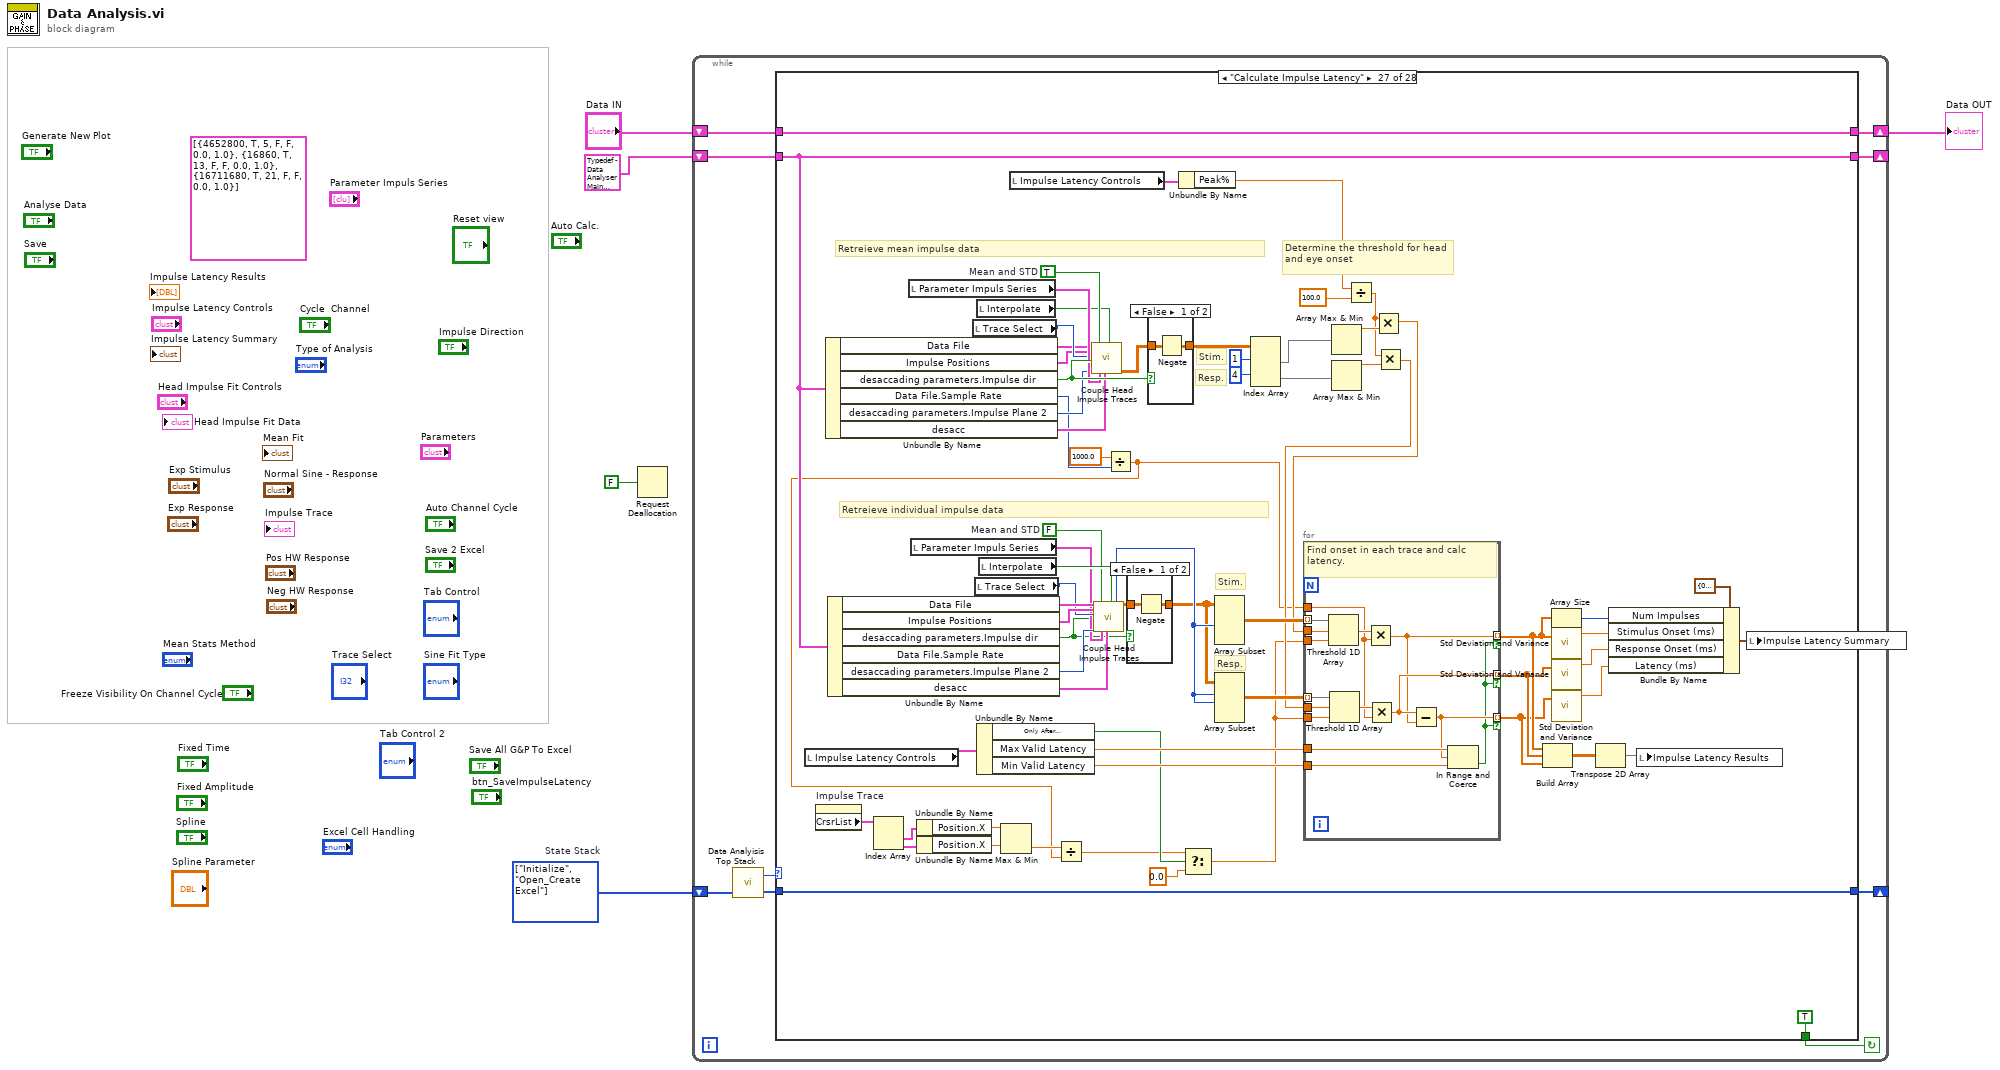
[diagram p0: block diagram]
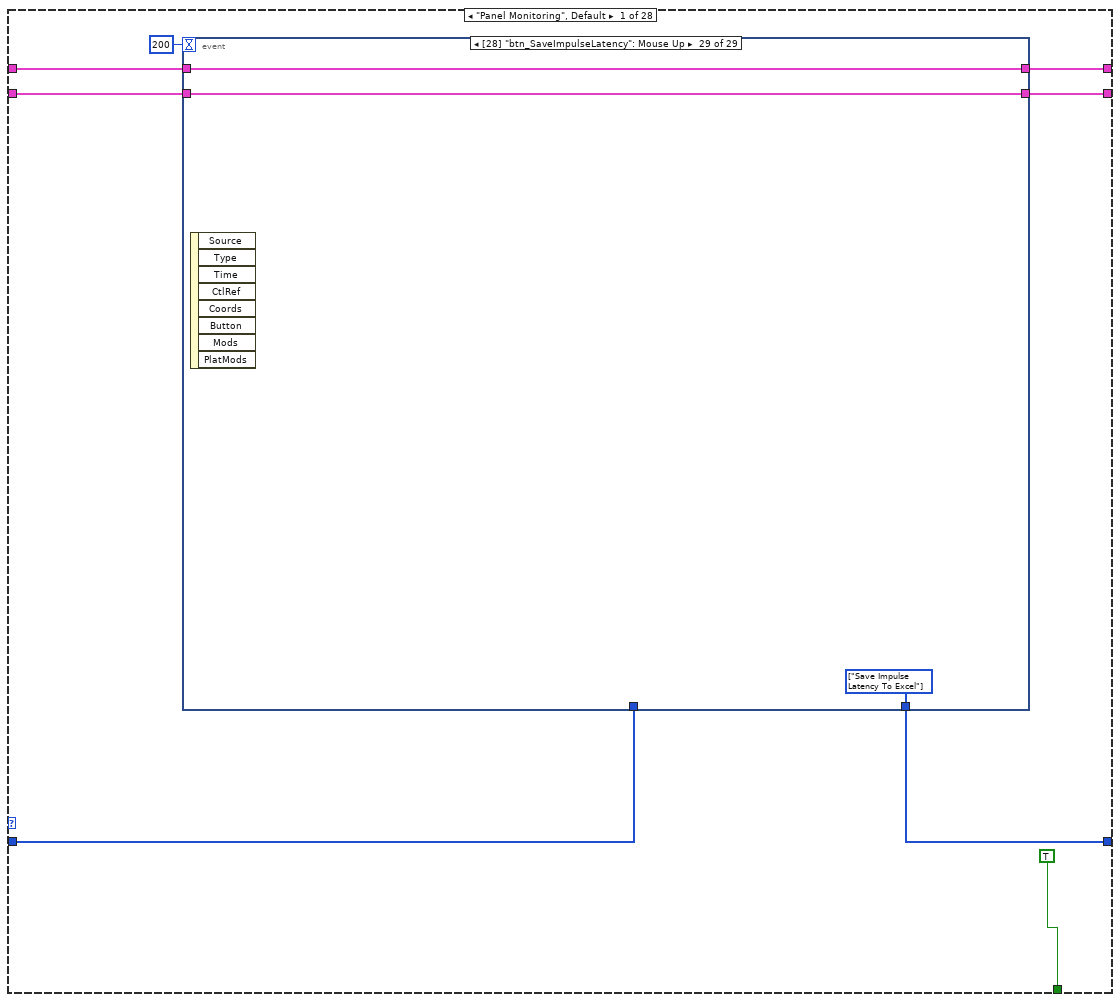
[diagram p2: hidden frame]
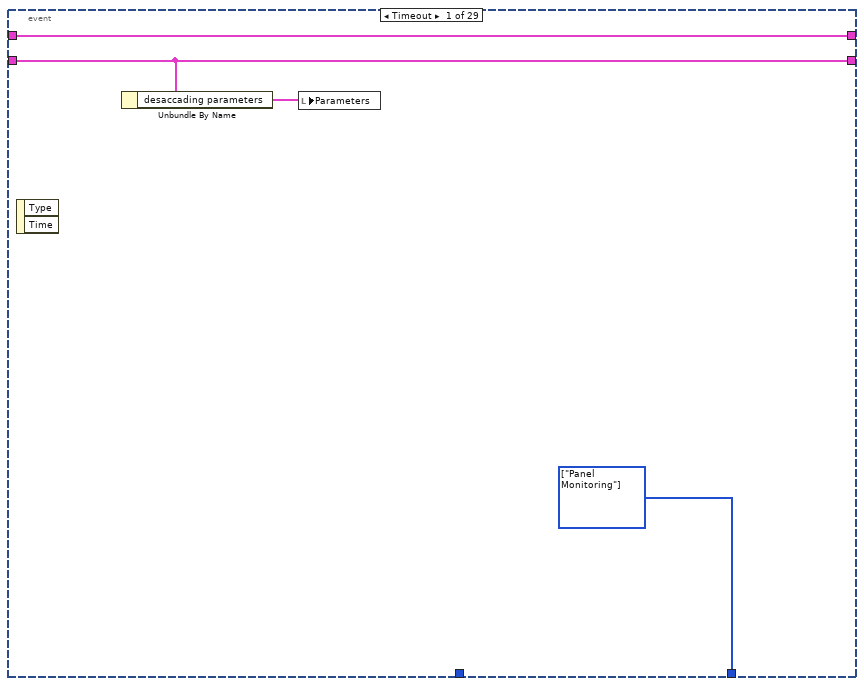
[diagram p3: hidden frame]
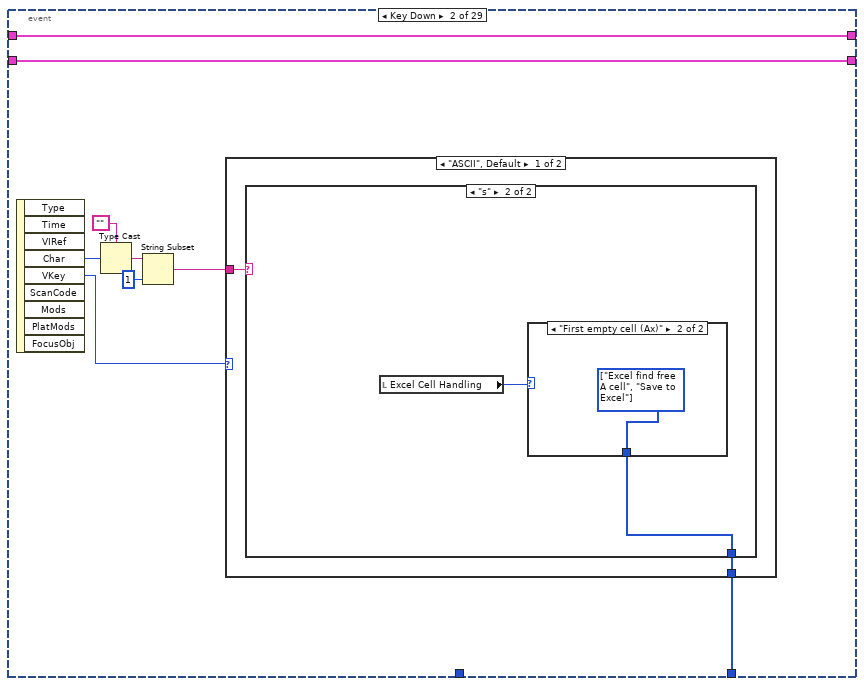
[diagram p4: hidden frame]
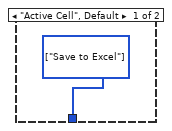
[diagram p6: hidden frame]
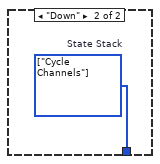
[diagram p7: hidden frame]
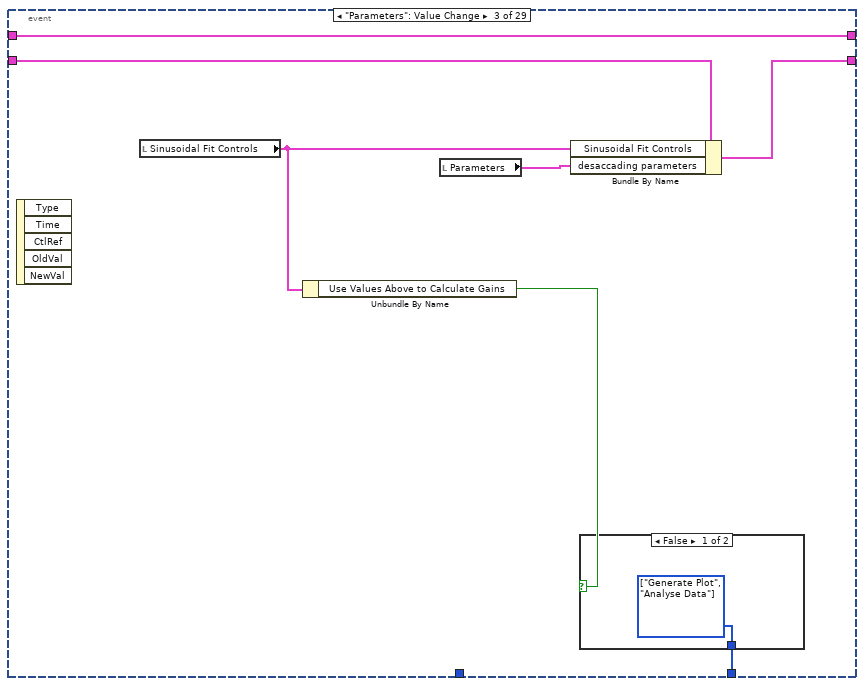
[diagram p8: hidden frame]
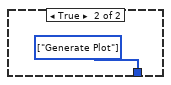
[diagram p9: hidden frame]
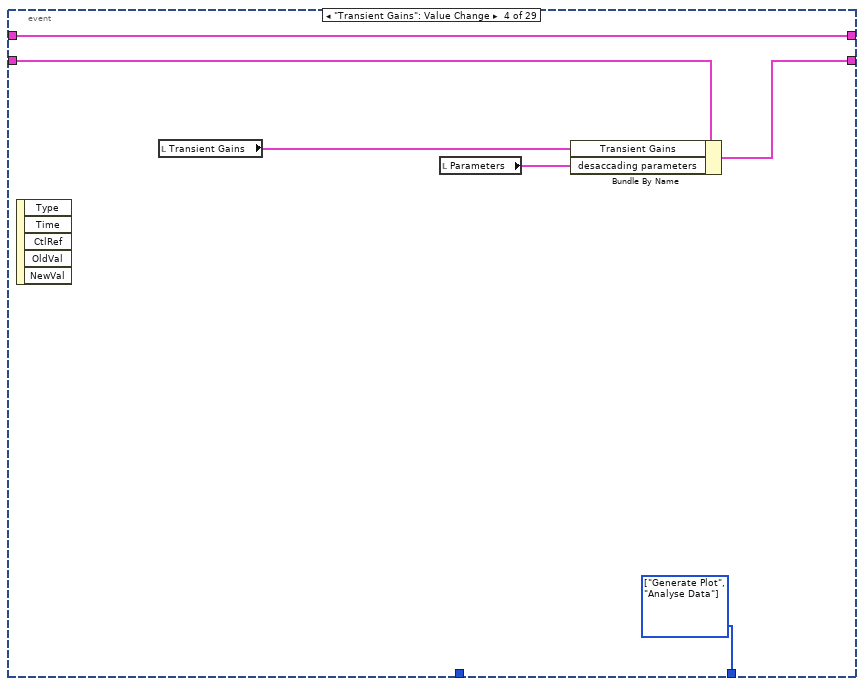
[diagram p10: hidden frame]
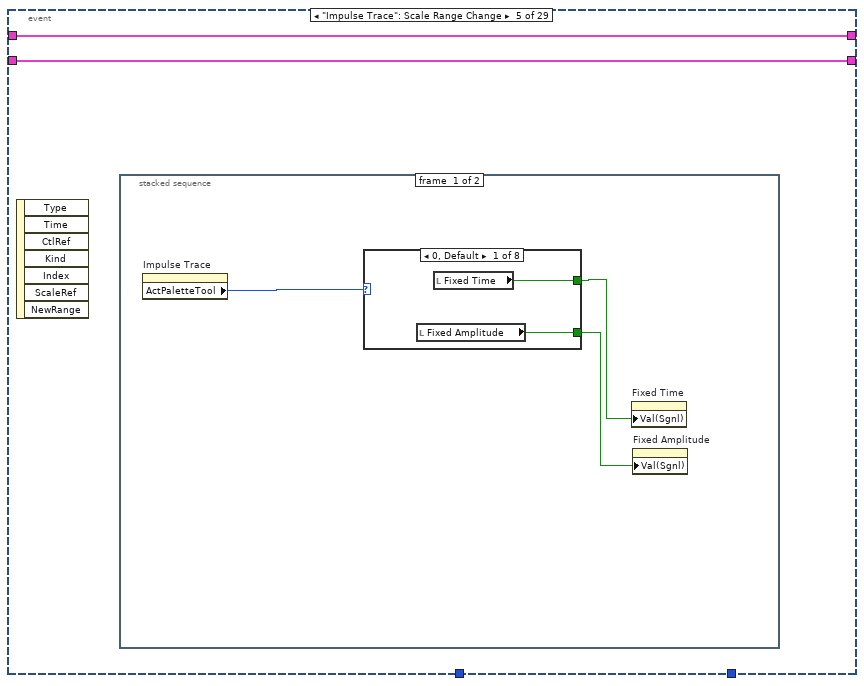
[diagram p11: hidden frame]
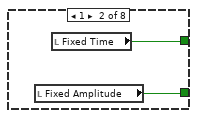
[diagram p12: hidden frame]
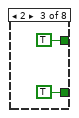
[diagram p13: hidden frame]
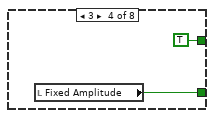
[diagram p14: hidden frame]
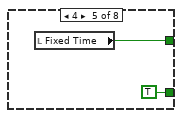
[diagram p15: hidden frame]
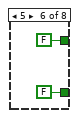
[diagram p16: hidden frame]
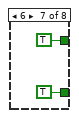
[diagram p17: hidden frame]
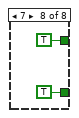
[diagram p18: hidden frame]
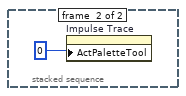
[diagram p19: hidden frame]
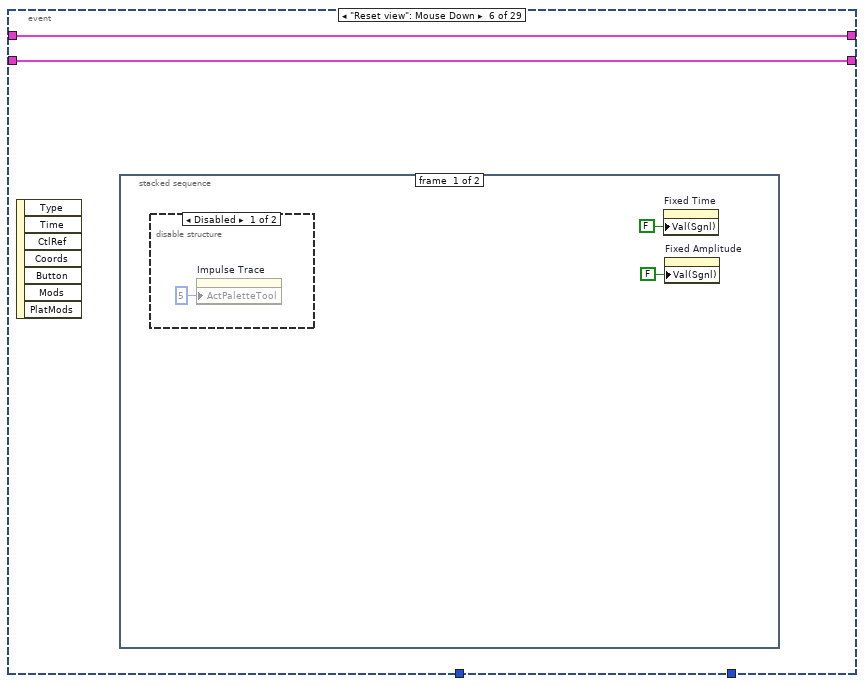
[diagram p20: hidden frame]
diagram:
  (unwired) T3 [{"Color"=4652800, "Visible"=TRUE, "Channel"=5, "Invert"=FALSE, "Desaccade"=FALSE, "Offset"=0.0, "Gain"=1.0}, {"Color"=16860, "Visible"=TRUE, "Channel"=13, "Invert"=FALSE, "Desaccade"=FALSE, "Offset"=0.0, "Gain"=1.0}, {"Color"=16711680, "Visible"=TRUE, "Channel"=21, "Invert"=FALSE, "Desaccade"=FALSE, "Offset"=0.0, "Gain"=1.0}] ("Parameter Impuls Series")
  w2 = T20[] [enum."Initialize", enum."Open_Create Excel"] items=["Quit", "Cycle Channels", "Generate Plot", "Analyse Data", "Save Image", "Polynomial Fit", "Open_Create Excel", "Excel find free A cell", "Panel Monitoring", "Save to Excel", "Initialize", "Extract Data", "Display Data", "Calculate Sinusoidal Gains", "Make Transient Fits & Equations", "Calculate Latency Fits", "Calculate Transient Ga 1 Gain", "Calculate Transient Ga 2 Gain", "Calculate Transient Gv Gain", "Stop", "Calculate Latency", "Calculate Exponential", "Calculate Mean", "Calculate Head Impulse", "Update controls and variables", "Save All Gain And Phase To Excel", "Calculate Impulse Latency", "Save Impulse Latency To Excel"]  # State Stack
  n1 = Request Deallocation(FALSE ("flag")) -> ()
  n2 = while {
    shift-left: w2 -> [w14]
    shift-right: [w12] -> _
    shift-right: [w6] -> _
    shift-left: T18 {"Impulse Positions"=[], "Data File"={"Data Channels"=[], "Sample Rate"=0, "Channel List"=[]}, "desaccading parameters"={"Tolerance"=0, "Acc Range"=0.0, "Sample Rate"=0, "Impulse Plane 2"=enum."Other", "Impulse dir"=FALSE}, "Stimulus"=[], "Response"=[], "Fitted Curves"=[], "Sinusoidal Fit Controls"={"Sinusoidal Response"={"Offset"=0.0, "Gain"=0.0, "Phase"=0.0, "Freq"=0.0}, "Sinusoidal Stimulus"={"Offset"=0.0, "Gain"=0.0, "Phase"=0.0, "Freq"=0.0}, "Stimulus\nFrequency"=0.0, "Stat."=enum."Mean Trace", "Use Values Above to Calculate Gains"=FALSE, "Automatically Calculate \nStimulus Frequency"=FALSE, "Gain and Phase"={"Gain"=0.0, "Gain SD"=0.0, "Phase"=0.0, "Phase SD"=0.0}}, "Transient Gains"={"Line Fit Response"={"Offset"=0.0, "Slope"=0.0}, "Stimulus Equation"="", "Reponse Equation"="", "Gv"=0.0, "Ga"=0.0, "Line Fit Stimulus"={"Offset"=0.0, "Slope"=0.0}, "Ga Window (early)"=0, "Gv Window"=0, "Latency (ms)"=0.0, "Stim.Onset"=0.0, "TH/#SDs 2"=0.0, "Response Onset"=0.0, "Snap Cursor"=0, "Latency"=0, "Poly. Window"=0, "Ord."=0, "BIC"=0.0, "Poly Equation"="", "Gv SD"=0.0, "Ga SD"=0.0, "Ga Stat."=0, "Mirror"=FALSE, "MSE"=0.0, "Gv Stat."=0, "Ga 2"=0.0, "Ga SD 2"=0.0, "Ga Window  (late)"=0, "Ga Stat. 2"=0, "GV desaccading"=FALSE, "GA2 desaccading"=FALSE, "GA1 desaccading"=FALSE, "Line Fit Response 2"={"Offset"=0.0, "Slope"=0.0}, "Stimulus Equation 2"="", "Reponse Equation 2"="", "Line Fit Stimulus 2"={"Offset"=0.0, "Slope"=0.0}, "Show Line Fit Parameters "=FALSE, "Gv Line Fit Stimulus"={"Offset"=0.0, "Slope"=0.0}, "Gv Line Fit Response"={"Offset"=0.0, "Slope"=0.0}, "Latency window"=0, "Latency Stat."=0, "Line Fit Res Latency"={"Offset"=0.0, "Slope"=0.0}, "Stim Eq Latency"="", "Resp Eq Latency"="", "Line Fit Stim Latency"={"Offset"=0.0, "Slope"=0.0}, "GA Line active"=0}, "Gv Line Fit Stimulus"={"Offset"=0.0, "Slope"=0.0}, "Gv Line Fit Response"={"Offset"=0.0, "Slope"=0.0}, "Fit Calculated"=FALSE, "Excel"={"Excel._Application"=refnum, "Use Excel"=FALSE, "Worksheet SINE"=refnum, "Row SINE"=0, "Worksheet TRANS"=refnum, "Row TRANS"=0}, "desacc "={"Threshold 1 [Acc]"=0.0, "Threshold 2 [% of TH1]"=0, "tolerance"=0, "Search WD "=0.0, " always use TH2"=FALSE, "Range"=0.0, "Max time"=0.0, "Min time"=0.0, "Velocity Threshold"=0}, "Impulse Data"=refnum, "Impulse Manager"=refnum, "Graph Manager"=refnum, "Sine Fit"=[], "Excel Logger"=refnum, "Halfwave Fit Display"=refnum, "Mean Fit"=refnum, "Exponential Fit"=refnum, "HI Fit"=refnum} ("output cluster") -> [w9]
    shift-right: [w7] -> w3
    shift-left: "Data IN" -> [w8]
    stop <- w10 continue-if-true
    n3 = call "Data Analyisis Top Stack.vi"("State Stack (in)"=w14) -> ("State Stack (out)"=w13:T20[], "State (out)"=w11:T20)  [unwired: 1 in]
    n4 = case shown="\"Calculate Impulse Latency\"" w11 {
      tunnel: w13 -> [w21 _ w284 w290 w369 w376 w535 w567 w572 _ _ _ w727 w848 w862 w1101 w1134 w1469 w1804 w2135 w2403 w2520 w2604 w2628 w2631 w2679 w2747 w2807]
      tunnel: [w20 w260 w284 w290 w369 w376 w535 w567 w571 w584 w610 w628 w725 w848 w862 w1101 w1134 w1469 w1804 w2135 w2403 w2520 w2604 w2628 w2631 w2679 w2747 w2807] -> w12
      tunnel: [TRUE TRUE FALSE TRUE TRUE TRUE FALSE TRUE TRUE TRUE TRUE TRUE TRUE TRUE TRUE TRUE TRUE TRUE TRUE TRUE TRUE TRUE TRUE TRUE TRUE TRUE TRUE TRUE] -> w10
      tunnel: w9 -> [w19 w227 w281 w285 w366 w374 w533 w564 w573 w580 w612 w622 w724 w847 w860 w1100 w1116 w1451 w1786 w2122 w2386 w2503 w2601 w2625 w2634 w2659 w2736 w2808]
      tunnel: [w18 w244 w281 w286 w366 w373 w533 w564 w573 w579 w612 w622 w723 w829 w861 w1094 w1133 w1468 w1803 w2134 w2385 w2504 w2603 w2627 w2633 w2659 w2736 w2808] -> w6
      tunnel: w8 -> [w17 w251 w282 w288 w367 w372 w532 w565 w574 w587 w613 w625 w728 w828 w851 w1099 w1103 w1439 w1774 w2109 w2361 w2474 w2605 w2629 w2649 w2652 w2763 w2794]
      tunnel: [w16 w251 w282 w288 w367 w372 w531 w565 w574 w587 w613 w624 w728 w827 w851 w1099 w1103 w1439 w1774 w2109 w2361 w2474 w2605 w2629 w2649 w2651 w2763 w2793] -> w7
      frame "Panel Monitoring", Default {
        n5 = event shown="[28] \"btn_SaveImpulseLatency\": Mouse Up" {
          selector: _ -> [_ _ _ _ _ _ _ _ _ _ _ _ _ _ _ _ _ _ _ _ _ _ _ _ _ _ _ _ _]
          dyn-events: _ -> [_ _ _ _ _ _ _ _ _ _ _ _ _ _ _ _ _ _ _ _ _ _ _ _ _ _ _ _ _]
          timeout: 200 -> [_ _ _ _ _ _ _ _ _ _ _ _ _ _ _ _ _ _ _ _ _ _ _ _ _ _ _ _ _]
          tunnel: w21 -> [_ _ _ _ _ _ _ _ _ _ _ _ _ _ _ _ _ _ _ _ _ _ _ _ _ _ w213 _ _]
          tunnel: [w26 w30 w48 w56 _ _ w86 w93 w96 w101 w108 w110 _ _ w131 w134 w138 w139 w144 w154 w166 w178 w190 w193 w198 w200 w211 w218 w221] -> w20
          tunnel: w19 -> [w24 w27 w47 w55 w58 w80 w88 w95 w97 w99 w104 w113 w118 w127 w129 w132 w136 w140 w146 w157 w169 w181 w191 w194 w196 w203 w214 w216 w219]
          tunnel: w17 -> [w25 w28 w49 w57 w59 w81 w87 w94 w98 w100 w109 w116 w122 w128 w130 w133 w137 w141 w147 w161 w173 w185 w192 w195 w197 w204 w215 w217 w220]
          tunnel: [w24 w27 w46 w54 w58 w80 w88 w95 w97 w99 w107 w112 w117 w126 w129 w132 w136 w140 w146 w156 w168 w180 w191 w194 w196 w203 w214 w216 w219] -> w18
          tunnel: [w25 w28 w49 w57 w59 w81 w87 w94 w98 w100 w109 w116 w122 w128 w130 w133 w137 w141 w147 w161 w173 w185 w192 w195 w197 w204 w215 w217 w220] -> w16
          event Timeout {
            w26 = T20[] [enum."Panel Monitoring"] items=["Quit", "Cycle Channels", "Generate Plot", "Analyse Data", "Save Image", "Polynomial Fit", "Open_Create Excel", "Excel find free A cell", "Panel Monitoring", "Save to Excel", "Initialize", "Extract Data", "Display Data", "Calculate Sinusoidal Gains", "Make Transient Fits & Equations", "Calculate Latency Fits", "Calculate Transient Ga 1 Gain", "Calculate Transient Ga 2 Gain", "Calculate Transient Gv Gain", "Stop", "Calculate Latency", "Calculate Exponential", "Calculate Mean", "Calculate Head Impulse", "Update controls and variables", "Save All Gain And Phase To Excel", "Calculate Impulse Latency", "Save Impulse Latency To Excel"] ("State Stack")
            n6 = event-data() -> ()  [unwired: 1 in, 2 out]
            n7 = Unbundle By Name(w24) -> ("desaccading parameters"=w23:T22)
            n8 = local write "Parameters"(w23) -> ()
          }
          event Key Down {
            n9 = event-data() -> ("Char"=w35:i16, "VKey"=w29:T23)  [unwired: 1 in, 7 out]
            n10 = Type Cast(type="", x=w35) -> (*(type *) &x=w33:string)
            n11 = String Subset(string=w33, offset (0)=1) -> (substring=w31:string)  [unwired: 1 in]
            n12 = case shown="\"ASCII\", Default" w29 {
              tunnel: w31 -> [w37 _]
              tunnel: [w36 w42] -> w30
              frame "ASCII", Default {
                n13 = case shown="\"s\"" w37 {
                  tunnel: [_ w39] -> w36
                  frame "False", Default {
                  }
                  frame "s" {
                    n14 = local read "Excel Cell Handling"() -> (w38:enum16{"Active Cell", "First empty cell (Ax)"})
                    n15 = case shown="\"First empty cell (Ax)\"" w38 {
                      tunnel: [w40 w41] -> w39
                      frame "Active Cell", Default {
                        w40 = T20[] [enum."Save to Excel"] items=["Quit", "Cycle Channels", "Generate Plot", "Analyse Data", "Save Image", "Polynomial Fit", "Open_Create Excel", "Excel find free A cell", "Panel Monitoring", "Save to Excel", "Initialize", "Extract Data", "Display Data", "Calculate Sinusoidal Gains", "Make Transient Fits & Equations", "Calculate Latency Fits", "Calculate Transient Ga 1 Gain", "Calculate Transient Ga 2 Gain", "Calculate Transient Gv Gain", "Stop", "Calculate Latency", "Calculate Exponential", "Calculate Mean", "Calculate Head Impulse", "Update controls and variables", "Save All Gain And Phase To Excel", "Calculate Impulse Latency", "Save Impulse Latency To Excel"] ("State Stack")
                      }
                      frame "First empty cell (Ax)" {
                        w41 = T20[] [enum."Excel find free A cell", enum."Save to Excel"] items=["Quit", "Cycle Channels", "Generate Plot", "Analyse Data", "Save Image", "Polynomial Fit", "Open_Create Excel", "Excel find free A cell", "Panel Monitoring", "Save to Excel", "Initialize", "Extract Data", "Display Data", "Calculate Sinusoidal Gains", "Make Transient Fits & Equations", "Calculate Latency Fits", "Calculate Transient Ga 1 Gain", "Calculate Transient Ga 2 Gain", "Calculate Transient Gv Gain", "Stop", "Calculate Latency", "Calculate Exponential", "Calculate Mean", "Calculate Head Impulse", "Update controls and variables", "Save All Gain And Phase To Excel", "Calculate Impulse Latency", "Save Impulse Latency To Excel"] ("State Stack")
                      }
                    }
                  }
                }
              }
              frame "Down" {
                w42 = T20[] [enum."Cycle Channels"] items=["Quit", "Cycle Channels", "Generate Plot", "Analyse Data", "Save Image", "Polynomial Fit", "Open_Create Excel", "Excel find free A cell", "Panel Monitoring", "Save to Excel", "Initialize", "Extract Data", "Display Data", "Calculate Sinusoidal Gains", "Make Transient Fits & Equations", "Calculate Latency Fits", "Calculate Transient Ga 1 Gain", "Calculate Transient Ga 2 Gain", "Calculate Transient Gv Gain", "Stop", "Calculate Latency", "Calculate Exponential", "Calculate Mean", "Calculate Head Impulse", "Update controls and variables", "Save All Gain And Phase To Excel", "Calculate Impulse Latency", "Save Impulse Latency To Excel"]  # State Stack
              }
            }
          }
          event "Parameters": Value Change {
            n16 = event-data() -> ()  [unwired: 1 in, 5 out]
            n17 = local read "Sinusoidal Fit Controls"() -> (w44:T5)
            n18 = Unbundle By Name(w44) -> ("Use Values Above to Calculate Gains"=w43:bool)
            n19 = local read "Parameters"() -> (w45:T16)
            n20 = Bundle By Name(cluster=w47, "Sinusoidal Fit Controls"=w44, "desaccading parameters"=w45) -> (w46:T18)
            n21 = case shown="False" w43 {
              tunnel: [w50 w51] -> w48
              frame False {
                w50 = T20[] [enum."Generate Plot", enum."Analyse Data"] items=["Quit", "Cycle Channels", "Generate Plot", "Analyse Data", "Save Image", "Polynomial Fit", "Open_Create Excel", "Excel find free A cell", "Panel Monitoring", "Save to Excel", "Initialize", "Extract Data", "Display Data", "Calculate Sinusoidal Gains", "Make Transient Fits & Equations", "Calculate Latency Fits", "Calculate Transient Ga 1 Gain", "Calculate Transient Ga 2 Gain", "Calculate Transient Gv Gain", "Stop", "Calculate Latency", "Calculate Exponential", "Calculate Mean", "Calculate Head Impulse", "Update controls and variables", "Save All Gain And Phase To Excel", "Calculate Impulse Latency", "Save Impulse Latency To Excel"] ("State Stack")
              }
              frame True {
                w51 = T20[] [enum."Generate Plot"] items=["Quit", "Cycle Channels", "Generate Plot", "Analyse Data", "Save Image", "Polynomial Fit", "Open_Create Excel", "Excel find free A cell", "Panel Monitoring", "Save to Excel", "Initialize", "Extract Data", "Display Data", "Calculate Sinusoidal Gains", "Make Transient Fits & Equations", "Calculate Latency Fits", "Calculate Transient Ga 1 Gain", "Calculate Transient Ga 2 Gain", "Calculate Transient Gv Gain", "Stop", "Calculate Latency", "Calculate Exponential", "Calculate Mean", "Calculate Head Impulse", "Update controls and variables", "Save All Gain And Phase To Excel", "Calculate Impulse Latency", "Save Impulse Latency To Excel"] ("State Stack")
              }
            }
          }
          event "Transient Gains": Value Change {
            w56 = T20[] [enum."Generate Plot", enum."Analyse Data"] items=["Quit", "Cycle Channels", "Generate Plot", "Analyse Data", "Save Image", "Polynomial Fit", "Open_Create Excel", "Excel find free A cell", "Panel Monitoring", "Save to Excel", "Initialize", "Extract Data", "Display Data", "Calculate Sinusoidal Gains", "Make Transient Fits & Equations", "Calculate Latency Fits", "Calculate Transient Ga 1 Gain", "Calculate Transient Ga 2 Gain", "Calculate Transient Gv Gain", "Stop", "Calculate Latency", "Calculate Exponential", "Calculate Mean", "Calculate Head Impulse", "Update controls and variables", "Save All Gain And Phase To Excel", "Calculate Impulse Latency", "Save Impulse Latency To Excel"] ("State Stack")
            n22 = event-data() -> ()  [unwired: 1 in, 5 out]
            n23 = local read "Transient Gains"() -> (w52:T9)
            n24 = local read "Parameters"() -> (w53:T16)
            n25 = Bundle By Name(cluster=w55, "Transient Gains"=w52, "desaccading parameters"=w53) -> (w54:T18)
          }
          event "Impulse Trace": Scale Range Change {
            n26 = event-data() -> ()  [unwired: 1 in, 7 out]
            n27 = stacked-sequence {
              frame #0 {
                n28 = property on="Impulse Trace" class="WFGraph (strict)"() -> ("ActPaletteTool"=w62:i32)  [unwired: 2 in, 2 out]
                n29 = case shown="0, Default" w62 {
                  tunnel: [w64 w65 TRUE ("Fixed Time") TRUE ("Fixed Time") w71 FALSE ("Fixed Time") TRUE ("Fixed Time") TRUE ("Fixed Time")] -> w61
                  tunnel: [w63 w66 TRUE ("Fixed Amplitude") w69 TRUE ("Fixed Amplitude") FALSE ("Fixed Amplitude") TRUE ("Fixed Amplitude") TRUE ("Fixed Amplitude")] -> w60
                  frame 0, Default {
                    n30 = local read "Fixed Amplitude"() -> (w63:bool)
                    n31 = local read "Fixed Time"() -> (w64:bool)
                  }
                  frame 1 {
                    n32 = local read "Fixed Amplitude"() -> (w66:bool)
                    n33 = local read "Fixed Time"() -> (w65:bool)
                  }
                  frame 2 {
                  }
                  frame 3 {
                    n34 = local read "Fixed Amplitude"() -> (w69:bool)
                  }
                  frame 4 {
                    n35 = local read "Fixed Time"() -> (w71:bool)
                  }
                  frame 5 {
                  }
                  frame 6 {
                  }
                  frame 7 {
                  }
                }
                n36 = property on="Fixed Time" class="Bool (strict)"("Val(Sgnl)"=w61) -> ()  [unwired: 2 in, 2 out]
                n37 = property on="Fixed Amplitude" class="Bool (strict)"("Val(Sgnl)"=w60) -> ()  [unwired: 2 in, 2 out]
              }
              frame #1 {
                n38 = property on="Impulse Trace" class="WFGraph (strict)"("ActPaletteTool"=0 ("Palette:Active Tool")) -> ()  [unwired: 2 in, 2 out]
              }
            }
          }
          event "Reset view": Mouse Down {
            n39 = event-data() -> ()  [unwired: 1 in, 7 out]
            n40 = stacked-sequence {
              frame #0 {
                n41 = disable-structure shown="Disabled" {
                  frame Disabled {
                    n42 = property on="Impulse Trace" class="WFGraph (strict)"("ActPaletteTool"=5 ("Palette:Active Tool")) -> ()  [unwired: 2 in, 2 out]
                  }
                  frame Enabled {
                  }
                }
                n43 = property on="Fixed Time" class="Bool (strict)"("Val(Sgnl)"=FALSE ("Value (Signaling)")) -> ()  [unwired: 2 in, 2 out]
                n44 = property on="Fixed Amplitude" class="Bool (strict)"("Val(Sgnl)"=FALSE ("Value (Signaling)")) -> ()  [unwired: 2 in, 2 out]
              }
              frame #1 {
                n45 = disable-structure shown="Disabled" {
                  frame Disabled {
                    n46 = property on="Impulse Trace" class="WFGraph (strict)"("ActPaletteTool"=0 ("Palette:Active Tool")) -> ()  [unwired: 2 in, 2 out]
                  }
                  frame Enabled {
                  }
                }
              }
            }
          }
          event "Hide Cursors": Value Change {
            w86 = T20[] [enum."Panel Monitoring"] items=["Quit", "Cycle Channels", "Generate Plot", "Analyse Data", "Save Image", "Polynomial Fit", "Open_Create Excel", "Excel find free A cell", "Panel Monitoring", "Save to Excel", "Initialize", "Extract Data", "Display Data", "Calculate Sinusoidal Gains", "Make Transient Fits & Equations", "Calculate Latency Fits", "Calculate Transient Ga 1 Gain", "Calculate Transient Ga 2 Gain", "Calculate Transient Gv Gain", "Stop", "Calculate Latency", "Calculate Exponential", "Calculate Mean", "Calculate Head Impulse", "Update controls and variables", "Save All Gain And Phase To Excel", "Calculate Impulse Latency", "Save Impulse Latency To Excel"] ("State Stack")
            n47 = event-data() -> ()  [unwired: 1 in, 5 out]
            n48 = Not(x="Hide Cursors") -> (.not. x?=w89:bool)
            n49 = property on="Impulse Trace" class="WFGraph (strict)"("Active Cursor"=u32 0, "Cursor.Visible"=w89) -> ()  [unwired: 2 in, 2 out]
            n50 = property on="Impulse Trace" class="WFGraph (strict)"("Active Cursor"=u32 1, "Cursor.Visible"=w89) -> ()  [unwired: 2 in, 2 out]
          }
          event "Impulse Trace": Cursor Release {
            w93 = T20[] [enum."Analyse Data"] items=["Quit", "Cycle Channels", "Generate Plot", "Analyse Data", "Save Image", "Polynomial Fit", "Open_Create Excel", "Excel find free A cell", "Panel Monitoring", "Save to Excel", "Initialize", "Extract Data", "Display Data", "Calculate Sinusoidal Gains", "Make Transient Fits & Equations", "Calculate Latency Fits", "Calculate Transient Ga 1 Gain", "Calculate Transient Ga 2 Gain", "Calculate Transient Gv Gain", "Stop", "Calculate Latency", "Calculate Exponential", "Calculate Mean", "Calculate Head Impulse", "Update controls and variables", "Save All Gain And Phase To Excel", "Calculate Impulse Latency", "Save Impulse Latency To Excel"] ("State Stack")
            n51 = event-data() -> ()  [unwired: 1 in, 9 out]
          }
          event "Hide Grid": Value Change {
            w96 = T20[] [enum."Panel Monitoring"] items=["Quit", "Cycle Channels", "Generate Plot", "Analyse Data", "Save Image", "Polynomial Fit", "Open_Create Excel", "Excel find free A cell", "Panel Monitoring", "Save to Excel", "Initialize", "Extract Data", "Display Data", "Calculate Sinusoidal Gains", "Make Transient Fits & Equations", "Calculate Latency Fits", "Calculate Transient Ga 1 Gain", "Calculate Transient Ga 2 Gain", "Calculate Transient Gv Gain", "Stop", "Calculate Latency", "Calculate Exponential", "Calculate Mean", "Calculate Head Impulse", "Update controls and variables", "Save All Gain And Phase To Excel", "Calculate Impulse Latency", "Save Impulse Latency To Excel"] ("State Stack")
            n52 = event-data() -> ()  [unwired: 1 in, 5 out]
          }
          event "Prefer Mean Fit": Value Change {
            w101 = T20[] [enum."Panel Monitoring"] items=["Quit", "Cycle Channels", "Generate Plot", "Analyse Data", "Save Image", "Polynomial Fit", "Open_Create Excel", "Excel find free A cell", "Panel Monitoring", "Save to Excel", "Initialize", "Extract Data", "Display Data", "Calculate Sinusoidal Gains", "Make Transient Fits & Equations", "Calculate Latency Fits", "Calculate Transient Ga 1 Gain", "Calculate Transient Ga 2 Gain", "Calculate Transient Gv Gain", "Stop", "Calculate Latency", "Calculate Exponential", "Calculate Mean", "Calculate Head Impulse", "Update controls and variables", "Save All Gain And Phase To Excel", "Calculate Impulse Latency", "Save Impulse Latency To Excel"] ("State Stack")
            n53 = event-data() -> ()  [unwired: 1 in, 6 out]
          }
          event "Impulse Direction": Value Change {
            w108 = T20[] [enum."Analyse Data"] items=["Quit", "Cycle Channels", "Generate Plot", "Analyse Data", "Save Image", "Polynomial Fit", "Open_Create Excel", "Excel find free A cell", "Panel Monitoring", "Save to Excel", "Initialize", "Extract Data", "Display Data", "Calculate Sinusoidal Gains", "Make Transient Fits & Equations", "Calculate Latency Fits", "Calculate Transient Ga 1 Gain", "Calculate Transient Ga 2 Gain", "Calculate Transient Gv Gain", "Stop", "Calculate Latency", "Calculate Exponential", "Calculate Mean", "Calculate Head Impulse", "Update controls and variables", "Save All Gain And Phase To Excel", "Calculate Impulse Latency", "Save Impulse Latency To Excel"] ("State Stack")
            n54 = event-data() -> ("NewVal"=w105:bool)  [unwired: 1 in, 4 out]
            n55 = Unbundle By Name(w104) -> ("Impulse Manager"=w106:refnum<class "Impulse Manager.lvclass">)
            n56 = call-dynamic "Set Direction.vi"("Direction"=w105, "Impulse Manager in"=w106) -> ("Impulse Manager out"=w102:refnum<class "Impulse Manager.lvclass">)  [unwired: 8 in, 1 out]
            n57 = Bundle By Name(cluster=w104, "Impulse Manager"=w102) -> (w103:T18)
            n58 = Bundle By Name(cluster=w103, "desaccading parameters.Impulse dir"=w105) -> (w107:T18)
          }
          event Value Change {
            w110 = T20[] [enum."Generate Plot"] items=["Quit", "Cycle Channels", "Generate Plot", "Analyse Data", "Save Image", "Polynomial Fit", "Open_Create Excel", "Excel find free A cell", "Panel Monitoring", "Save to Excel", "Initialize", "Extract Data", "Display Data", "Calculate Sinusoidal Gains", "Make Transient Fits & Equations", "Calculate Latency Fits", "Calculate Transient Ga 1 Gain", "Calculate Transient Ga 2 Gain", "Calculate Transient Gv Gain", "Stop", "Calculate Latency", "Calculate Exponential", "Calculate Mean", "Calculate Head Impulse", "Update controls and variables", "Save All Gain And Phase To Excel", "Calculate Impulse Latency", "Save Impulse Latency To Excel"] ("State Stack")
            n59 = event-data() -> ("NewVal"=w114:T3)  [unwired: 1 in, 5 out]
            n60 = Unbundle By Name(w113) -> ("Impulse Manager"=w115:refnum<class "Impulse Manager.lvclass">)
            n61 = call-dynamic "Set Channels.vi"("Channel Selector in"=w114, "Impulse Manager in"=w115) -> ("Impulse Manager out"=w111:refnum<class "Impulse Manager.lvclass">)  [unwired: 8 in, 1 out]
            n62 = Bundle By Name(cluster=w113, "Impulse Manager"=w111) -> (w112:T18)
          }
          event "Fixed Amplitude": Value Change {
            n63 = event-data() -> ("NewVal"=w120:bool)  [unwired: 1 in, 5 out]
            n64 = Unbundle By Name(w118) -> ("Graph Manager"=w121:refnum<class "Graph Manager.lvclass">)
            n65 = call-dynamic "Set Y Scale Lock.vi"("Lock"=w120, "Graph Manager in"=w121) -> ("Graph Manager out"=w119:refnum<class "Graph Manager.lvclass">)  [unwired: 8 in, 1 out]
            n66 = Bundle By Name(cluster=w118, "Graph Manager"=w119) -> (w117:T18)
          }
          event "Fixed Time": Value Change {
            n67 = event-data() -> ("NewVal"=w123:bool)  [unwired: 1 in, 5 out]
            n68 = Unbundle By Name(w127) -> ("Graph Manager"=w125:refnum<class "Graph Manager.lvclass">)
            n69 = call-dynamic "Set X Scale Lock.vi"("Lock"=w123, "Graph Manager in"=w125) -> ("Graph Manager out"=w124:refnum<class "Graph Manager.lvclass">)  [unwired: 8 in, 1 out]
            n70 = Bundle By Name(cluster=w127, "Graph Manager"=w124) -> (w126:T18)
          }
          event "Show Fit", "Mean Traces": Value Change {
            w131 = T20[] [enum."Display Data"] items=["Quit", "Cycle Channels", "Generate Plot", "Analyse Data", "Save Image", "Polynomial Fit", "Open_Create Excel", "Excel find free A cell", "Panel Monitoring", "Save to Excel", "Initialize", "Extract Data", "Display Data", "Calculate Sinusoidal Gains", "Make Transient Fits & Equations", "Calculate Latency Fits", "Calculate Transient Ga 1 Gain", "Calculate Transient Ga 2 Gain", "Calculate Transient Gv Gain", "Stop", "Calculate Latency", "Calculate Exponential", "Calculate Mean", "Calculate Head Impulse", "Update controls and variables", "Save All Gain And Phase To Excel", "Calculate Impulse Latency", "Save Impulse Latency To Excel"]  # State Stack
            n71 = event-data() -> ()  [unwired: 1 in, 6 out]
          }
          event "Sine Fit Type": Value Change {
            w134 = T20[] [enum."Update controls and variables", enum."Display Data"] items=["Quit", "Cycle Channels", "Generate Plot", "Analyse Data", "Save Image", "Polynomial Fit", "Open_Create Excel", "Excel find free A cell", "Panel Monitoring", "Save to Excel", "Initialize", "Extract Data", "Display Data", "Calculate Sinusoidal Gains", "Make Transient Fits & Equations", "Calculate Latency Fits", "Calculate Transient Ga 1 Gain", "Calculate Transient Ga 2 Gain", "Calculate Transient Gv Gain", "Stop", "Calculate Latency", "Calculate Exponential", "Calculate Mean", "Calculate Head Impulse", "Update controls and variables", "Save All Gain And Phase To Excel", "Calculate Impulse Latency", "Save Impulse Latency To Excel"] ("State Stack")
            n72 = event-data() -> ()  [unwired: 1 in, 6 out]
          }
          event Panel Close? {
            w138 = T20[] [enum."Quit"] items=["Quit", "Cycle Channels", "Generate Plot", "Analyse Data", "Save Image", "Polynomial Fit", "Open_Create Excel", "Excel find free A cell", "Panel Monitoring", "Save to Excel", "Initialize", "Extract Data", "Display Data", "Calculate Sinusoidal Gains", "Make Transient Fits & Equations", "Calculate Latency Fits", "Calculate Transient Ga 1 Gain", "Calculate Transient Ga 2 Gain", "Calculate Transient Gv Gain", "Stop", "Calculate Latency", "Calculate Exponential", "Calculate Mean", "Calculate Head Impulse", "Update controls and variables", "Save All Gain And Phase To Excel", "Calculate Impulse Latency", "Save Impulse Latency To Excel"]  # State Stack
            n73 = event-data() -> ()  [unwired: 1 in, 4 out]
            n74 = event-data("Discard?"=TRUE) -> ()  [unwired: 1 in, 1 out]
          }
          event "Generate New Plot": Mouse Up {
            w139 = T20[] [enum."Generate Plot"] items=["Quit", "Cycle Channels", "Generate Plot", "Analyse Data", "Save Image", "Polynomial Fit", "Open_Create Excel", "Excel find free A cell", "Panel Monitoring", "Save to Excel", "Initialize", "Extract Data", "Display Data", "Calculate Sinusoidal Gains", "Make Transient Fits & Equations", "Calculate Latency Fits", "Calculate Transient Ga 1 Gain", "Calculate Transient Ga 2 Gain", "Calculate Transient Gv Gain", "Stop", "Calculate Latency", "Calculate Exponential", "Calculate Mean", "Calculate Head Impulse", "Update controls and variables", "Save All Gain And Phase To Excel", "Calculate Impulse Latency", "Save Impulse Latency To Excel"] ("State Stack")
            n75 = event-data() -> ()  [unwired: 1 in, 7 out]
          }
          event Value Change {
            w144 = T20[] [enum."Panel Monitoring"] items=["Quit", "Cycle Channels", "Generate Plot", "Analyse Data", "Save Image", "Polynomial Fit", "Open_Create Excel", "Excel find free A cell", "Panel Monitoring", "Save to Excel", "Initialize", "Extract Data", "Display Data", "Calculate Sinusoidal Gains", "Make Transient Fits & Equations", "Calculate Latency Fits", "Calculate Transient Ga 1 Gain", "Calculate Transient Ga 2 Gain", "Calculate Transient Gv Gain", "Stop", "Calculate Latency", "Calculate Exponential", "Calculate Mean", "Calculate Head Impulse", "Update controls and variables", "Save All Gain And Phase To Excel", "Calculate Impulse Latency", "Save Impulse Latency To Excel"]  # State Stack
            n76 = event-data() -> ("NewVal"=w145:T17)  [unwired: 1 in, 5 out]
            n77 = case shown="\"Impulse Latency\"" w145 {
              frame "Sinusoidal", Default {
                n78 = local write "Tab Control"(T4."Sinusoid" ("Tab Control")) -> ()
              }
              frame "Transient" {
                n79 = local write "Tab Control"(T4."Transient" ("Tab Control")) -> ()
              }
              frame "Mean" {
                n80 = local write "Tab Control"(T4."Mean" ("Tab Control")) -> ()
              }
              frame "Exponential" {
                n81 = local write "Tab Control"(T4."Exponential" ("Tab Control")) -> ()
              }
              frame "Head Impulse" {
                n82 = local write "Tab Control"(T4."Head Impulse" ("Tab Control")) -> ()
              }
              frame "Impulse Latency" {
                n83 = local write "Tab Control"(T4."Impulse Latency" ("Tab Control")) -> ()
              }
            }
            n84 = property on="Transient Gains" class="Clust (strict)"("Visible"=TRUE) -> ()  [unwired: 2 in, 2 out]
            n85 = property on="Sinusoidal Fit Controls" class="Clust (strict)"("Visible"=FALSE) -> ()  [unwired: 2 in, 2 out]
          }
          event Value Change {
            w154 = T20[] [enum."Update controls and variables", enum."Display Data"] items=["Quit", "Cycle Channels", "Generate Plot", "Analyse Data", "Save Image", "Polynomial Fit", "Open_Create Excel", "Excel find free A cell", "Panel Monitoring", "Save to Excel", "Initialize", "Extract Data", "Display Data", "Calculate Sinusoidal Gains", "Make Transient Fits & Equations", "Calculate Latency Fits", "Calculate Transient Ga 1 Gain", "Calculate Transient Ga 2 Gain", "Calculate Transient Gv Gain", "Stop", "Calculate Latency", "Calculate Exponential", "Calculate Mean", "Calculate Head Impulse", "Update controls and variables", "Save All Gain And Phase To Excel", "Calculate Impulse Latency", "Save Impulse Latency To Excel"] ("State Stack")
            n86 = event-data() -> ("NewVal"=w158:T6)  [unwired: 1 in, 5 out]
            n87 = Unbundle By Name(w157) -> ("Sine Fit"=w160:refnum<class "Sinusoidal Fit.lvclass">[])
            n88 = in-place {
              in-place-border: w158 -> [w164]
              n89 = in-place-array #1(w160, 0) -> (w165:refnum<class "Sinusoidal Fit.lvclass">)
              n90 = call-dynamic "Set Response Coefficients.vi"("Coefficients"=w164, "Sinusoidal Fit in"=w165) -> ("Sinusoidal Fit out"=w163:refnum<class "Sinusoidal Fit.lvclass">)  [unwired: 8 in, 1 out]
              n91 = call-dynamic "Adjust Gain and Phase.vi"("Sinusoidal Fit in"=w163) -> ("Sinusoidal Fit out"=w162:refnum<class "Sinusoidal Fit.lvclass">)  [unwired: 9 in, 1 out]
              n92 = in-place-array #1(w162) -> (w155:refnum<class "Sinusoidal Fit.lvclass">[])  [unwired: 1 out]
            }
            n93 = Bundle By Name(cluster=w157, "Sine Fit"=w155) -> (w156:T18)
          }
          event Value Change {
            w166 = T20[] [enum."Update controls and variables", enum."Display Data"] items=["Quit", "Cycle Channels", "Generate Plot", "Analyse Data", "Save Image", "Polynomial Fit", "Open_Create Excel", "Excel find free A cell", "Panel Monitoring", "Save to Excel", "Initialize", "Extract Data", "Display Data", "Calculate Sinusoidal Gains", "Make Transient Fits & Equations", "Calculate Latency Fits", "Calculate Transient Ga 1 Gain", "Calculate Transient Ga 2 Gain", "Calculate Transient Gv Gain", "Stop", "Calculate Latency", "Calculate Exponential", "Calculate Mean", "Calculate Head Impulse", "Update controls and variables", "Save All Gain And Phase To Excel", "Calculate Impulse Latency", "Save Impulse Latency To Excel"] ("State Stack")
            n94 = event-data() -> ("NewVal"=w170:T6)  [unwired: 1 in, 5 out]
            n95 = Unbundle By Name(w169) -> ("Sine Fit"=w172:refnum<class "Sinusoidal Fit.lvclass">[])
            n96 = in-place {
              in-place-border: w170 -> [w174]
              n97 = in-place-array #2(w172, 2) -> (w177:refnum<class "Sinusoidal Fit.lvclass">)
              n98 = call-dynamic "Set Response Coefficients.vi"("Coefficients"=w174, "Sinusoidal Fit in"=w177) -> ("Sinusoidal Fit out"=w176:refnum<class "Sinusoidal Fit.lvclass">)  [unwired: 8 in, 1 out]
              n99 = call-dynamic "Adjust Gain and Phase.vi"("Sinusoidal Fit in"=w176) -> ("Sinusoidal Fit out"=w175:refnum<class "Sinusoidal Fit.lvclass">)  [unwired: 9 in, 1 out]
              n100 = in-place-array #2(w175) -> (w167:refnum<class "Sinusoidal Fit.lvclass">[])  [unwired: 1 out]
            }
            n101 = Bundle By Name(cluster=w169, "Sine Fit"=w167) -> (w168:T18)
          }
          event Value Change {
            w178 = T20[] [enum."Update controls and variables", enum."Display Data"] items=["Quit", "Cycle Channels", "Generate Plot", "Analyse Data", "Save Image", "Polynomial Fit", "Open_Create Excel", "Excel find free A cell", "Panel Monitoring", "Save to Excel", "Initialize", "Extract Data", "Display Data", "Calculate Sinusoidal Gains", "Make Transient Fits & Equations", "Calculate Latency Fits", "Calculate Transient Ga 1 Gain", "Calculate Transient Ga 2 Gain", "Calculate Transient Gv Gain", "Stop", "Calculate Latency", "Calculate Exponential", "Calculate Mean", "Calculate Head Impulse", "Update controls and variables", "Save All Gain And Phase To Excel", "Calculate Impulse Latency", "Save Impulse Latency To Excel"] ("State Stack")
            n102 = event-data() -> ("NewVal"=w182:T6)  [unwired: 1 in, 5 out]
            n103 = Unbundle By Name(w181) -> ("Sine Fit"=w184:refnum<class "Sinusoidal Fit.lvclass">[])
            n104 = in-place {
              in-place-border: w182 -> [w186]
              n105 = in-place-array #3(w184, 1) -> (w189:refnum<class "Sinusoidal Fit.lvclass">)
              n106 = call-dynamic "Set Response Coefficients.vi"("Coefficients"=w186, "Sinusoidal Fit in"=w189) -> ("Sinusoidal Fit out"=w188:refnum<class "Sinusoidal Fit.lvclass">)  [unwired: 8 in, 1 out]
              n107 = call-dynamic "Adjust Gain and Phase.vi"("Sinusoidal Fit in"=w188) -> ("Sinusoidal Fit out"=w187:refnum<class "Sinusoidal Fit.lvclass">)  [unwired: 9 in, 1 out]
              n108 = in-place-array #3(w187) -> (w179:refnum<class "Sinusoidal Fit.lvclass">[])  [unwired: 1 out]
            }
            n109 = Bundle By Name(cluster=w181, "Sine Fit"=w179) -> (w180:T18)
          }
          event "Analyse Data": Mouse Up {
            w190 = T20[] [enum."Analyse Data"] items=["Quit", "Cycle Channels", "Generate Plot", "Analyse Data", "Save Image", "Polynomial Fit", "Open_Create Excel", "Excel find free A cell", "Panel Monitoring", "Save to Excel", "Initialize", "Extract Data", "Display Data", "Calculate Sinusoidal Gains", "Make Transient Fits & Equations", "Calculate Latency Fits", "Calculate Transient Ga 1 Gain", "Calculate Transient Ga 2 Gain", "Calculate Transient Gv Gain", "Stop", "Calculate Latency", "Calculate Exponential", "Calculate Mean", "Calculate Head Impulse", "Update controls and variables", "Save All Gain And Phase To Excel", "Calculate Impulse Latency", "Save Impulse Latency To Excel"] ("State Stack")
            n110 = event-data() -> ()  [unwired: 1 in, 7 out]
          }
          event Value Change {
            w193 = T20[] [enum."Analyse Data"] items=["Quit", "Cycle Channels", "Generate Plot", "Analyse Data", "Save Image", "Polynomial Fit", "Open_Create Excel", "Excel find free A cell", "Panel Monitoring", "Save to Excel", "Initialize", "Extract Data", "Display Data", "Calculate Sinusoidal Gains", "Make Transient Fits & Equations", "Calculate Latency Fits", "Calculate Transient Ga 1 Gain", "Calculate Transient Ga 2 Gain", "Calculate Transient Gv Gain", "Stop", "Calculate Latency", "Calculate Exponential", "Calculate Mean", "Calculate Head Impulse", "Update controls and variables", "Save All Gain And Phase To Excel", "Calculate Impulse Latency", "Save Impulse Latency To Excel"] ("State Stack")
            n111 = event-data() -> ()  [unwired: 1 in, 6 out]
          }
          event "Cycle  Channel": Mouse Up {
            w198 = T20[] [enum."Cycle Channels"] items=["Quit", "Cycle Channels", "Generate Plot", "Analyse Data", "Save Image", "Polynomial Fit", "Open_Create Excel", "Excel find free A cell", "Panel Monitoring", "Save to Excel", "Initialize", "Extract Data", "Display Data", "Calculate Sinusoidal Gains", "Make Transient Fits & Equations", "Calculate Latency Fits", "Calculate Transient Ga 1 Gain", "Calculate Transient Ga 2 Gain", "Calculate Transient Gv Gain", "Stop", "Calculate Latency", "Calculate Exponential", "Calculate Mean", "Calculate Head Impulse", "Update controls and variables", "Save All Gain And Phase To Excel", "Calculate Impulse Latency", "Save Impulse Latency To Excel"] ("State Stack")
            n112 = event-data() -> ()  [unwired: 1 in, 7 out]
          }
          event "Save 2 Excel": Mouse Up {
            n113 = event-data() -> ()  [unwired: 1 in, 7 out]
            n114 = local read "Excel Cell Handling"() -> (w199:enum16{"Active Cell", "First empty cell (Ax)"})
            n115 = case shown="\"First empty cell (Ax)\"" w199 {
              tunnel: [w209 w210] -> w201
              frame "Active Cell", Default {
                w209 = T20[] [enum."Save to Excel"] items=["Quit", "Cycle Channels", "Generate Plot", "Analyse Data", "Save Image", "Polynomial Fit", "Open_Create Excel", "Excel find free A cell", "Panel Monitoring", "Save to Excel", "Initialize", "Extract Data", "Display Data", "Calculate Sinusoidal Gains", "Make Transient Fits & Equations", "Calculate Latency Fits", "Calculate Transient Ga 1 Gain", "Calculate Transient Ga 2 Gain", "Calculate Transient Gv Gain", "Stop", "Calculate Latency", "Calculate Exponential", "Calculate Mean", "Calculate Head Impulse", "Update controls and variables", "Save All Gain And Phase To Excel", "Calculate Impulse Latency", "Save Impulse Latency To Excel"] ("State Stack")
              }
              frame "First empty cell (Ax)" {
                w210 = T20[] [enum."Excel find free A cell", enum."Save to Excel"] items=["Quit", "Cycle Channels", "Generate Plot", "Analyse Data", "Save Image", "Polynomial Fit", "Open_Create Excel", "Excel find free A cell", "Panel Monitoring", "Save to Excel", "Initialize", "Extract Data", "Display Data", "Calculate Sinusoidal Gains", "Make Transient Fits & Equations", "Calculate Latency Fits", "Calculate Transient Ga 1 Gain", "Calculate Transient Ga 2 Gain", "Calculate Transient Gv Gain", "Stop", "Calculate Latency", "Calculate Exponential", "Calculate Mean", "Calculate Head Impulse", "Update controls and variables", "Save All Gain And Phase To Excel", "Calculate Impulse Latency", "Save Impulse Latency To Excel"] ("State Stack")
              }
            }
            n116 = local read "Auto Channel Cycle"() -> (w202:bool)
            n117 = case shown="True" w202 {
              tunnel: w201 -> [w205 w207]
              tunnel: [w205 w208] -> w200
              frame False {
              }
              frame True {
                n118 = Build Array (concatenate)(w207, Data_Analysis_state."Cycle Channels" ("State (out)")) -> (w208:T20[])
              }
            }
          }
          event "Save All G&P To Excel": Mouse Up {
            w212 = T20[] [enum."Save All Gain And Phase To Excel"] items=["Quit", "Cycle Channels", "Generate Plot", "Analyse Data", "Save Image", "Polynomial Fit", "Open_Create Excel", "Excel find free A cell", "Panel Monitoring", "Save to Excel", "Initialize", "Extract Data", "Display Data", "Calculate Sinusoidal Gains", "Make Transient Fits & Equations", "Calculate Latency Fits", "Calculate Transient Ga 1 Gain", "Calculate Transient Ga 2 Gain", "Calculate Transient Gv Gain", "Stop", "Calculate Latency", "Calculate Exponential", "Calculate Mean", "Calculate Head Impulse", "Update controls and variables", "Save All Gain And Phase To Excel", "Calculate Impulse Latency", "Save Impulse Latency To Excel"] ("element")
            n119 = event-data() -> ()  [unwired: 1 in, 8 out]
            n120 = Build Array (concatenate)(w213, w212) -> (w211:T20[])
          }
          event "Save": Mouse Up {
            w218 = T20[] [enum."Save Image"] items=["Quit", "Cycle Channels", "Generate Plot", "Analyse Data", "Save Image", "Polynomial Fit", "Open_Create Excel", "Excel find free A cell", "Panel Monitoring", "Save to Excel", "Initialize", "Extract Data", "Display Data", "Calculate Sinusoidal Gains", "Make Transient Fits & Equations", "Calculate Latency Fits", "Calculate Transient Ga 1 Gain", "Calculate Transient Ga 2 Gain", "Calculate Transient Gv Gain", "Stop", "Calculate Latency", "Calculate Exponential", "Calculate Mean", "Calculate Head Impulse", "Update controls and variables", "Save All Gain And Phase To Excel", "Calculate Impulse Latency", "Save Impulse Latency To Excel"]  # State Stack
            n121 = event-data() -> ()  [unwired: 1 in, 7 out]
          }
          event "btn_SaveImpulseLatency": Mouse Up {
            w221 = T20[] [enum."Save Impulse Latency To Excel"] items=["Quit", "Cycle Channels", "Generate Plot", "Analyse Data", "Save Image", "Polynomial Fit", "Open_Create Excel", "Excel find free A cell", "Panel Monitoring", "Save to Excel", "Initialize", "Extract Data", "Display Data", "Calculate Sinusoidal Gains", "Make Transient Fits & Equations", "Calculate Latency Fits", "Calculate Transient Ga 1 Gain", "Calculate Transient Ga 2 Gain", "Calculate Transient Gv Gain", "Stop", "Calculate Latency", "Calculate Exponential", "Calculate Mean", "Calculate Head Impulse", "Update controls and variables", "Save All Gain And Phase To Excel", "Calculate Impulse Latency", "Save Impulse Latency To Excel"] ("State Stack")
            n122 = event-data() -> ()  [unwired: 1 in, 8 out]
          }
        }
      }
      frame "Initialize" {
        w252 = FALSE  # Fit Calculated
        w260 = T20[] [enum."Open_Create Excel", enum."Excel find free A cell", enum."Update controls and variables", enum."Generate Plot", enum."Analyse Data", enum."Panel Monitoring"] items=["Quit", "Cycle Channels", "Generate Plot", "Analyse Data", "Save Image", "Polynomial Fit", "Open_Create Excel", "Excel find free A cell", "Panel Monitoring", "Save to Excel", "Initialize", "Extract Data", "Display Data", "Calculate Sinusoidal Gains", "Make Transient Fits & Equations", "Calculate Latency Fits", "Calculate Transient Ga 1 Gain", "Calculate Transient Ga 2 Gain", "Calculate Transient Gv Gain", "Stop", "Calculate Latency", "Calculate Exponential", "Calculate Mean", "Calculate Head Impulse", "Update controls and variables", "Save All Gain And Phase To Excel", "Calculate Impulse Latency", "Save Impulse Latency To Excel"]  # State Stack
        n123 = Unbundle By Name(w251) -> ("Impulse Positions"=w240:T24, "Data File"=w242:T25, "desaccading parameters"=w239:T22, "Experiment Parameters.Stimulus"=w250:string, "Experiment Parameters.Freq"=w228:dbl, "Parameter Impuls Series"=w237:T3, "Excel"=w246:T26, "desacc"=w225:T27)
        n124 = call-dynamic "Set Desaccading Parameters.vi"("Parameter"=w225, "Desaccade Manipulator in"=refnum<class "Desaccade Manipulator.lvclass"> refnum ("Desaccade Manipulator.lvclass")) -> ("Desaccade Manipulator out"=w222:refnum<class "Desaccade Manipulator.lvclass">)  [unwired: 8 in, 1 out]
        n125 = call "Constructor.vi"() -> ("data value reference"=w243:T19)  [unwired: 11 in]
        n126 = case shown="Default" w250 {
          frame Default {
            n127 = local write "Type of Analysis"(Typedef_-_Type_of_Analysis."Mean" ("Type of Analysis")) -> ()
            n128 = local write "Tab Control"(T4."Mean" ("Tab Control")) -> ()
          }
          frame "TRANSIENT" {
            n129 = local read "Prefer Mean Fit"() -> (w265:bool)
            n130 = case shown="False" w265 {
              tunnel: [Typedef_-_Type_of_Analysis."Transient" ("Type of Analysis") Typedef_-_Type_of_Analysis."Mean" ("Type of Analysis")] -> w266
              tunnel: [T4."Transient" ("Tab Control") T4."Mean" ("Tab Control")] -> w264
              frame False {
              }
              frame True {
              }
            }
            n131 = local write "Type of Analysis"(w266) -> ()
            n132 = local write "Tab Control"(w264) -> ()
          }
          frame "SINE" {
            n133 = local write "Type of Analysis"(Typedef_-_Type_of_Analysis."Sinusoidal" ("Type of Analysis")) -> ()
            n134 = local write "Tab Control"(T4."Sinusoid" ("Tab Control")) -> ()
          }
          frame "EXP" {
            n135 = local write "Type of Analysis"(Typedef_-_Type_of_Analysis."Exponential" ("Type of Analysis")) -> ()
            n136 = local write "Tab Control"(T4."Exponential" ("Tab Control")) -> ()
          }
          frame "HIT-Horizontal" {
            n137 = local write "Type of Analysis"(Typedef_-_Type_of_Analysis."Head Impulse" ("Type of Analysis")) -> ()
            n138 = local write "Tab Control"(T4."Head Impulse" ("Tab Control")) -> ()
          }
        }
        n139 = Bundle By Name(cluster="Sinusoidal Fit Controls", "Stimulus\nFrequency"=w228) -> (w248:T5)
        n140 = local write "Stimulus\nFrequency"(w228) -> ()
        n141 = local write "Parameter Impuls Series"(w237) -> ()
        n142 = control-ref of="Impulse Trace"() -> (w236:refnum<vi>)
        n143 = Unbundle By Name(w239) -> ("Impulse Plane 2"=w238:T28, "Impulse dir"=w229:bool)
        n144 = call "Set Time Data.vi"("Time Series Data"=w242, "Reference in"=w243) -> ("Reference out"=w241:T19)  [unwired: 8 in, 1 out]
        n145 = call "Set Impulse Positions.vi"("Impulse Positions"=w240, "Reference in"=w241) -> ("Reference out"=w234:T19)  [unwired: 9 in]
        n146 = call "Constructor with Impulse Reference.vi"("Impulse Object Reference"=w234) -> ("Impulse Manager.lvclass"=w235:refnum<class "Impulse Manager.lvclass">)  [unwired: 10 in]
        n147 = call "Constructor Singleton.vi"() -> ("Excel Logger.lvclass"=w233:refnum<class "Excel Logger.lvclass">)  [unwired: 11 in]
        n148 = call "Constructor.vi"("Graph Reference"=w236) -> ("Graph Manager out"=w232:refnum<class "Graph Manager.lvclass">)  [unwired: 10 in]
        n149 = call-dynamic "Set Impulse Plane.vi"("Impulse Plane"=w238, "Impulse Manager in"=w235) -> ("Impulse Manager out"=w231:refnum<class "Impulse Manager.lvclass">)  [unwired: 8 in, 1 out]
        n150 = call-dynamic "Set Direction.vi"("Direction"=w229, "Impulse Manager in"=w231) -> ("Impulse Manager out"=w230:refnum<class "Impulse Manager.lvclass">)  [unwired: 8 in, 1 out]
        n151 = call-dynamic "Set Channels.vi"("Channel Selector in"=w237, "Impulse Manager in"=w230) -> ("Impulse Manager out"=w224:refnum<class "Impulse Manager.lvclass">)  [unwired: 8 in, 1 out]
        n152 = call-dynamic "Set Desaccade Manipulator.vi"("Desaccade Manipulator.lvclass"=w222, "Impulse Manager in"=w224) -> ("Impulse Manager out"=w223:refnum<class "Impulse Manager.lvclass">)  [unwired: 8 in, 1 out]
        n153 = Unbundle By Name(w242) -> ("Channel List"=w245:string[])
        n154 = local write "Parameters"(w239) -> ()
        n155 = Unbundle By Name(w239) -> ("Impulse dir"=w247:bool)
        n156 = Bundle By Name(cluster=w227, "Impulse Positions"=w240, "Data File"=w242, "desaccading parameters"=w239, "Stimulus"="Stimulus", "Response"="Response", "Fitted Curves"="Fitted Curves", "Sinusoidal Fit Controls"=w248, "Transient Gains"="Transient Gains", "Transient Gains.Gv Line Fit Stimulus"="Gv Line Fit Stimulus", "Transient Gains.Gv Line Fit Response"="Gv Line Fit Response", "Fit Calculated"=w252, "Excel"=w246, "desacc"=w225, "Impulse Data"=w234, "Impulse Manager"=w223, "Graph Manager"=w232, "Excel Logger"=w233) -> (w244:T18)
        n157 = local write "Impulse Direction"(w247) -> ()
        n158 = property on="Response Onset" class="DigNum (strict)"("Visible"=FALSE) -> ()  [unwired: 2 in, 2 out]
        n159 = property on="Channel" class="Ring (strict)"("Strings []"=w245) -> ()  [unwired: 2 in, 2 out]
      }
      frame "Quit" {
        n160 = Unbundle By Name(w281) -> ("Halfwave Fit Display"=w280:refnum<class "Halfwave Fit Display.lvclass">, "Excel Logger"=w278:refnum<class "Excel Logger.lvclass">, "Impulse Data"=w277:T19)
        n161 = call-dynamic "Stop Core.vi"("Halfwave Fit Display in"=w280) -> ()  [unwired: 9 in, 2 out]
        n162 = call "Constructor Singleton.vi"("Enum"=enum16{"Init", "Update"}."Update", "Excel Logger.lvclass 2"=w278) -> ()  [unwired: 9 in, 1 out]
        n163 = call "Destructor.vi"("data value reference"=w277) -> ()  [unwired: 11 in]
      }
      frame "Excel find free A cell" {
        n164 = Unbundle By Name(w285) -> ("Excel.Use Excel"=w287:bool)
        n165 = disable-structure shown="Enabled" {
          disable-tunnel: w287 -> [w293 _]
          disable-tunnel: [w292 w350] -> w286
          disable-tunnel: w285 -> [w291 w350]
          frame Disabled {
            n166 = case shown="True" w293 {
              tunnel: [w294 w298] -> w292
              tunnel: w291 -> [w294 w299]
              tunnel: w291 -> [_ w303]
              frame False {
              }
              frame True {
                n167 = local read item#-1() -> (w296)
                n168 = case shown="\"Sinusoidal\", Default" w296 {
                  tunnel: w303 -> [w346 w349]
                  tunnel: [w344 w348] -> w302
                  tunnel: [w345 w347] -> w300
                  frame "Transient" {
                    n169 = Unbundle By Name(w346) -> ("Excel.Worksheet TRANS"=w345:refnum<k7>, "Excel.Row TRANS"=w344:i32)
                  }
                  frame "Sinusoidal", Default {
                    n170 = Unbundle By Name(w349) -> ("Excel.Worksheet SINE"=w347:refnum<k7>, "Excel.Row SINE"=w348:i32)
                  }
                }
                n171 = while {
                  shift-right: [w315] -> w297
                  shift-left: w302 -> [w320]
                  shift-right: [w324] -> _
                  shift-left: FALSE -> [w323]
                  shift-right: [w312] -> w295
                  shift-left: w300 -> [w317]
                  stop <- w318 stop-if-true
                  n172 = call "Excel Num to Cell.vi"("Column"=1, "Row"=w320) -> ("Cell"=w330:string)  [unwired: 3 in]
                  n173 = To Variant(anything=w330) -> (Variant=w329:variant)
                  n174 = invoke class="_Worksheet" method="Range"(reference=w317, "Cell1"=w329) -> (reference out=w312:refnum<k7>, "Range"=w328:refnum<k7>)  [unwired: 3 in, 3 out]
                  n175 = property class="Range"(reference=w328) -> ("Value2"=w325:variant)  [unwired: 1 in, 2 out]
                  n176 = Variant To Data(type="", Variant=w325) -> (data=w327:string)  [unwired: 1 in, 1 out]
                  n177 = Empty String/Path?(string/path=w327) -> (empty?=w324:bool)
                  n178 = Build Array(w324, w323) -> (w322:bool[])
                  n179 = Boolean Array To Number(Boolean array=w322) -> (number=w321:u32)
                  n180 = case shown="2" w321 {
                    tunnel: w320 -> [w334 w337 w340 w343]
                    tunnel: [w333 w336 w339 w342] -> w314
                    tunnel: [FALSE FALSE TRUE FALSE] -> w319
                    frame 0, Default {
                      # "No empty cell found, \ngo to next"
                      n181 = Increment(x=w334) -> (x+1=w333:i32)
                    }
                    frame 1 {
                      # "Empty Cell found,\nreverse direction"
                      n182 = Decrement(x=w337) -> (x-1=w336:i32)
                    }
                    frame 2 {
                      # "First empty cell found"
                      n183 = Increment(x=w340) -> (x+1=w339:i32)
                    }
                    frame 3 {
                      # "Two empty cells found,\nreduce cell by one"
                      n184 = Decrement(x=w343) -> (x-1=w342:i32)
                    }
                  }
                  n185 = Less Or Equal To 0?(x=w314) -> (x <= 0?=w316:bool)
                  n186 = Compound Arithmetic op=OR(w316, w319) -> (w318:bool)
                  n187 = Select(t=1, s=w316, f=w314) -> (s? t:f=w315:i32)
                }
                n188 = case shown="\"Sinusoidal\", Default" w296 {
                  tunnel: w299 -> [w306 w311]
                  tunnel: [w307 w310] -> w298
                  tunnel: w297 -> [w305 w309]
                  tunnel: w295 -> [w304 w308]
                  frame "Sinusoidal", Default {
                    n189 = Bundle By Name(cluster=w306, "Excel.Row SINE"=w305, "Excel.Worksheet SINE"=w304) -> (w307:T18)
                  }
                  frame "Transient" {
                    n190 = Bundle By Name(cluster=w311, "Excel.Row TRANS"=w309, "Excel.Worksheet TRANS"=w308) -> (w310:T18)
                  }
                }
              }
            }
          }
          frame Enabled {
          }
        }
      }
      frame "Open_Create Excel" {
        n191 = Unbundle By Name(w366) -> ("Excel Logger"=w365:refnum<class "Excel Logger.lvclass">)
        n192 = call "Get Sinusoidal Sheet.vi"("Excel Logger in"=w365) -> ("Data Analyser Report.lvclass"=w364:refnum<class "Data Analyser Report.lvclass">, "Excel Logger out"=w362:refnum<class "Excel Logger.lvclass">)  [unwired: 8 in, 1 out]
        n193 = call-dynamic "Write Header.vi"("Header"=string[] ["ID", "Type", "Rot.Plane", "Experimenter", "Trial", "Eye", "Eye.Plane", "Direction", "Freq", "Vel", "Acc", "Cycles", "Gain", "Gain.SD", "Phase", "Phase.SD", "Offset", "Filename"], "Data Analyser Report in"=w364) -> ()  [unwired: 8 in, 2 out]
        n194 = call "Get Transient Sheet.vi"("Excel Logger in"=w362) -> ("Data Analyser Report.lvclass"=w361:refnum<class "Data Analyser Report.lvclass">, "Excel Logger out"=w359:refnum<class "Excel Logger.lvclass">)  [unwired: 8 in, 1 out]
        n195 = call-dynamic "Write Header.vi"("Header"=string[] ["ID", "Type", "Rot.Plane", "Experimenter", "Trial", "Eye", "Eye.Plane", "Direction", "Acc", "Vel", "Cycles", "GA1", "GA1.SD", "GA2", "GA2.SD", "GV", "GV.SD", "Latency"], "Data Analyser Report in"=w361) -> ()  [unwired: 8 in, 2 out]
        n196 = call "Get Mean Sheet.vi"("Excel Logger in"=w359) -> ("Data Analyser Report.lvclass"=w358:refnum<class "Data Analyser Report.lvclass">, "Excel Logger out"=w356:refnum<class "Excel Logger.lvclass">)  [unwired: 8 in, 1 out]
        n197 = call-dynamic "Write Header.vi"("Header"=string[] ["ID", "Type", "Rot.Plane", "Experimenter", "Trial", "Eye", "Eye.Plane", "Direction", "Stimulus", "Number Impulses", "Stimulus.Mean", "Stimulus.SD", "Response.Mean", "Response.SD"], "Data Analyser Report in"=w358) -> ()  [unwired: 8 in, 2 out]
        n198 = call "Get Exponential Sheet.vi"("Excel Logger in"=w356) -> ("Exponential"=w355:refnum<class "Data Analyser Report.lvclass">, "Excel Logger out"=w353:refnum<class "Excel Logger.lvclass">)  [unwired: 8 in, 1 out]
        n199 = call-dynamic "Write Header.vi"("Header"=string[] ["ID", "Type", "Rot.Plane", "Experimenter", "Trial", "Eye", "Eye.Plane", "Direction", "Stimulus", "Number Impulses", "Stimulus.Amplitude", "Stimulus.Duration", "Stimulus.TC", "Stimulus.Offset", "Response.Amplitude", "Response.Duration", "Response.TC", "Response.Offset"], "Data Analyser Report in"=w355) -> ()  [unwired: 8 in, 2 out]
        n200 = call "Get Head Impulse Sheet.vi"("Excel Logger in"=w353) -> ("Head Impulse"=w351:refnum<class "Data Analyser Report.lvclass">)  [unwired: 8 in, 2 out]
        n201 = call-dynamic "Write Header.vi"("Header"=string[] ["ID", "Type", "Rot.Plane", "Experimenter", "Trial", "Eye", "Eye.Plane", "Direction", "Stimulus", "Number Impulses", "Peak Head Velocity (deg/s)", "Gain", "Gain.SD", "Peak-Peak Lag (ms)", "Peak-Peak Lag (ms).SD", "GainW1", "GainW1.SD", "LagW1", "LagW1.SD", "GainW2", "GainW2.SD", "LagW2", "LagW2.SD", "GainW3", "GainW3.SD", "LagW3", "LagW3.SD"], "Data Analyser Report in"=w351) -> ()  [unwired: 8 in, 2 out]
      }
      frame "Save to Excel" {
        n202 = property on="Type of Analysis" class="Enum (strict)"() -> ("Value"=w370:T17)  [unwired: 2 in, 2 out]
        n203 = Unbundle By Name(w374) -> ("Excel Logger"=w371:refnum<class "Excel Logger.lvclass">)
        n204 = case shown="\"Transient\"" w370 {
          tunnel: w371 -> [w390 w440 w452 w477 w505]
          tunnel: w372 -> [w378 w439 w456 w484 w512]
          tunnel: w374 -> [w388 w424 w457 w485 w513]
          tunnel: w374 -> [w381 w434 w459 w487 w515]
          tunnel: [w380 w433 w458 w486 w514] -> w373
          frame "Sinusoidal", Default {
            n205 = call "Get Sinusoidal Sheet.vi"("Excel Logger in"=w390) -> ("Data Analyser Report.lvclass"=w386:refnum<class "Data Analyser Report.lvclass">, "Excel Logger out"=w382:refnum<class "Excel Logger.lvclass">)  [unwired: 8 in, 1 out]
            n206 = Unbundle By Name(w388) -> ("Sine Fit"=w387:refnum<class "Sinusoidal Fit.lvclass">[], "Impulse Manager"=w385:refnum<class "Impulse Manager.lvclass">)
            n207 = Unbundle By Name(w378) -> ("Experiment Parameters 2"=w389:T29, "Experiment Parameters"=w384:T30)
            n208 = Unbundle By Name(w378) -> ("filename"=w377:string)
            n209 = for {
              tunnel: w389 -> [w415]
              tunnel: w387 -> [w403] mode=indexing
              shift-right: [w392] -> w383
              shift-left: w386 -> [w405]
              tunnel: w385 -> [w411]
              tunnel: w384 -> [w394]
              tunnel: w377 -> [w391]
              n210 = call-dynamic "Find first empty row.vi"("Excel Sheet in"=w405) -> ("Excel Sheet out"=w404:refnum<class "Data Analyser Report.lvclass">)  [unwired: 8 in, 2 out]
              n211 = call "Write Experiment Parameter.vi"("Experiment Parameters"=w415, "Data Analyser Reportin"=w404) -> ("Data Analyser Report out"=w412:refnum<class "Data Analyser Report.lvclass">)  [unwired: 9 in]
              n212 = call "Write Eye and Eye Axis.vi"("Impulse Manager"=w411, "Data Analyser Report in"=w412) -> ("Data Analyser Report out"=w410:refnum<class "Data Analyser Report.lvclass">)  [unwired: 8 in, 1 out]
              n213 = call-dynamic "Direction to String.vi"("Sinusoidal Fit in"=w403) -> ("String"=w413:string, "Sinusoidal Fit out"=w409:refnum<class "Sinusoidal Fit.lvclass">)  [unwired: 8 in, 1 out]
              n214 = call-dynamic "Get Stimulus Coefficients.vi"("Sinusoidal Fit in"=w403) -> ("Coefficients"=w402:T6)  [unwired: 8 in, 2 out]
              n215 = call-dynamic "Get Response Coefficients.vi"("Sinusoidal Fit in"=w403) -> ("Coefficients"=w401:T6)  [unwired: 8 in, 2 out]
              n216 = Unbundle By Name(w402) -> ("Offset"=w399:dbl)
              n217 = Unbundle By Name(w401) -> ("Offset"=w400:dbl)
              n218 = call-poly "Write to Cell.vi"("Value"=w413, "Excel Sheet in"=w410) -> ("Excel Sheet out"=w395:refnum<class "Data Analyser Report.lvclass">)  [unwired: 9 in]
              n219 = call-dynamic "Write Sinusoid Stimulus Parameter.vi"("Stimulus Parameters"=w394, "Data Analyser Report in"=w395) -> ("Data Analyser Report out"=w396:refnum<class "Data Analyser Report.lvclass">)  [unwired: 8 in, 1 out]
              n220 = call-dynamic "Get Impulse Count.vi"("Abstract Fit in"=w409) -> ("Nr of Fit Impulses"=w407:i32, "Abstract Fit out"=w408:refnum<class "Sinusoidal Fit.lvclass">)  [unwired: 8 in, 1 out]
              n221 = Subtract(x=w400, y=w399) -> (x-y=w397:dbl)
              n222 = call-poly "Write to Cell.vi"("Value"=w407, "Excel Sheet in"=w396) -> ("Excel Sheet out"=w406:refnum<class "Data Analyser Report.lvclass">)  [unwired: 9 in]
              n223 = call-dynamic "Fit Result to String.vi"("Sinusoidal Fit in"=w408) -> ("Array"=w414:string[])  [unwired: 8 in, 2 out]
              n224 = for {
                tunnel: w414 -> [w417] mode=indexing
                shift-right: [w416] -> w398
                shift-left: w406 -> [w418]
                n225 = call-poly "Write to Cell.vi"("Value"=w417, "Excel Sheet in"=w418) -> ("Excel Sheet out"=w416:refnum<class "Data Analyser Report.lvclass">)  [unwired: 9 in]
              }
              n226 = call-poly "Write to Cell.vi"("Value"=w397, "Excel Sheet in"=w398) -> ("Excel Sheet out"=w393:refnum<class "Data Analyser Report.lvclass">)  [unwired: 9 in]
              n227 = call-poly "Write to Cell.vi"("Value"=w391, "Excel Sheet in"=w393) -> ("Excel Sheet out"=w392:refnum<class "Data Analyser Report.lvclass">)  [unwired: 9 in]
            }
            n228 = call "Write Sinusoid Sheet.vi"("Data Analyser Report.lvclass"=w383, "Excel Logger in"=w382) -> ("Excel Logger out"=w379:refnum<class "Excel Logger.lvclass">)  [unwired: 8 in, 1 out]
            n229 = Bundle By Name(cluster=w381, "Excel Logger"=w379) -> (w380:T18)
          }
          frame "Transient" {
            n230 = call "Get Transient Sheet.vi"("Excel Logger in"=w440) -> ("Data Analyser Report.lvclass"=w437:refnum<class "Data Analyser Report.lvclass">, "Excel Logger out"=w435:refnum<class "Excel Logger.lvclass">)  [unwired: 8 in, 1 out]
            n231 = Unbundle By Name(w424) -> ("Transient Gains"=w426:T9, "Impulse Manager"=w436:refnum<class "Impulse Manager.lvclass">)
            n232 = Unbundle By Name(w424) -> ("desaccading parameters.Impulse dir"=w423:bool)
            n233 = Unbundle By Name(w439) -> ("Experiment Parameters 2"=w438:T29, "Experiment Parameters"=w419:T30, "No. Imp"=w422:i32)
            n234 = call-dynamic "Find first empty row.vi"("Excel Sheet in"=w437) -> ("Excel Sheet out"=w429:refnum<class "Data Analyser Report.lvclass">)  [unwired: 8 in, 2 out]
            n235 = call "Write Experiment Parameter.vi"("Experiment Parameters"=w438, "Data Analyser Reportin"=w429) -> ("Data Analyser Report out"=w431:refnum<class "Data Analyser Report.lvclass">)  [unwired: 9 in]
            n236 = case shown="False" w423 {
              tunnel: ["NEG" "POS"] -> w425
              frame False {
              }
              frame True {
              }
            }
            n237 = call "Write Eye and Eye Axis.vi"("Impulse Manager"=w436, "Data Analyser Report in"=w431) -> ("Data Analyser Report out"=w430:refnum<class "Data Analyser Report.lvclass">)  [unwired: 8 in, 1 out]
            n238 = call-poly "Write to Cell.vi"("Value"=w425, "Excel Sheet in"=w430) -> ("Excel Sheet out"=w421:refnum<class "Data Analyser Report.lvclass">)  [unwired: 9 in]
            n239 = call-dynamic "Write Transient Stimulus Parameter.vi"("Stimulus Parameters"=w419, "Data Analyser Report in"=w421) -> ("Data Analyser Report out"=w420:refnum<class "Data Analyser Report.lvclass">)  [unwired: 8 in, 1 out]
            n240 = call-poly "Write to Cell.vi"("Value"=w422, "Excel Sheet in"=w420) -> ("Excel Sheet out"=w428:refnum<class "Data Analyser Report.lvclass">)  [unwired: 9 in]
            n241 = call-dynamic "Write Transient temporarily.vi"("Transient Gains 2"=w426, "Data Analyser Report in"=w428) -> ("Data Analyser Report out"=w427:refnum<class "Data Analyser Report.lvclass">)  [unwired: 8 in, 1 out]
            n242 = call "Write Transient Sheet.vi"("Data Analyser Report.lvclass"=w427, "Excel Logger in"=w435) -> ("Excel Logger out"=w432:refnum<class "Excel Logger.lvclass">)  [unwired: 8 in, 1 out]
            n243 = Bundle By Name(cluster=w434, "Excel Logger"=w432) -> (w433:T18)
          }
          frame "Mean" {
            n244 = call "Get Mean Sheet.vi"("Excel Logger in"=w452) -> ("Data Analyser Report.lvclass"=w451:refnum<class "Data Analyser Report.lvclass">, "Excel Logger out"=w449:refnum<class "Excel Logger.lvclass">)  [unwired: 8 in, 1 out]
            n245 = Unbundle By Name(w457) -> ("Impulse Manager"=w443:refnum<class "Impulse Manager.lvclass">, "Mean Fit"=w455:refnum<class "Mean Fit.lvclass">)
            n246 = Unbundle By Name(w456) -> ("Experiment Parameters 2"=w465:T29, "Experiment Parameters.Stimulus"=w445:string)
            n247 = Unbundle By Name(w457) -> ("desaccading parameters.Impulse dir"=w460:bool)
            n248 = call-dynamic "Find first empty row.vi"("Excel Sheet in"=w451) -> ("Excel Sheet out"=w462:refnum<class "Data Analyser Report.lvclass">)  [unwired: 8 in, 2 out]
            n249 = call "Write Experiment Parameter.vi"("Experiment Parameters"=w465, "Data Analyser Reportin"=w462) -> ("Data Analyser Report out"=w464:refnum<class "Data Analyser Report.lvclass">)  [unwired: 9 in]
            n250 = case shown="False" w460 {
              tunnel: ["NEG" "POS"] -> w461
              frame False {
              }
              frame True {
              }
            }
            n251 = call "Write Eye and Eye Axis.vi"("Impulse Manager"=w443, "Data Analyser Report in"=w464) -> ("Data Analyser Report out"=w463:refnum<class "Data Analyser Report.lvclass">)  [unwired: 8 in, 1 out]
            n252 = call-poly "Write to Cell.vi"("Value"=w461, "Excel Sheet in"=w463) -> ("Excel Sheet out"=w446:refnum<class "Data Analyser Report.lvclass">)  [unwired: 9 in]
            n253 = call-poly "Write to Cell.vi"("Value"=w445, "Excel Sheet in"=w446) -> ("Excel Sheet out"=w447:refnum<class "Data Analyser Report.lvclass">)  [unwired: 9 in]
            n254 = call "Get Number of Impulses.vi"("Impulse Manager in"=w443) -> ("Number of impulses"=w444:i32)  [unwired: 8 in, 2 out]
            n255 = call-poly "Write to Cell.vi"("Value"=w444, "Excel Sheet in"=w447) -> ("Excel Sheet out"=w454:refnum<class "Data Analyser Report.lvclass">)  [unwired: 9 in]
            n256 = call-dynamic "Fit Result to String.vi"("Mean Fit in"=w455) -> ("Array"=w453:string[])  [unwired: 8 in, 2 out]
            n257 = for {
              tunnel: w453 -> [w467] mode=indexing
              shift-right: [w466] -> w450
              shift-left: w454 -> [w468]
              n258 = call-poly "Write to Cell.vi"("Value"=w467, "Excel Sheet in"=w468) -> ("Excel Sheet out"=w466:refnum<class "Data Analyser Report.lvclass">)  [unwired: 9 in]
            }
            n259 = call "Write Mean Sheet.vi"("Data Analyser Report.lvclass"=w450, "Excel Logger in"=w449) -> ("Excel Logger out"=w448:refnum<class "Excel Logger.lvclass">)  [unwired: 8 in, 1 out]
            n260 = Bundle By Name(cluster=w459, "Excel Logger"=w448) -> (w458:T18)
          }
          frame "Exponential" {
            n261 = call "Get Exponential Sheet.vi"("Excel Logger in"=w477) -> ("Exponential"=w476:refnum<class "Data Analyser Report.lvclass">, "Excel Logger out"=w475:refnum<class "Excel Logger.lvclass">)  [unwired: 8 in, 1 out]
            n262 = Unbundle By Name(w485) -> ("Impulse Manager"=w471:refnum<class "Impulse Manager.lvclass">, "Exponential Fit"=w483:refnum<class "Exponential Fit.lvclass">)
            n263 = Unbundle By Name(w484) -> ("Experiment Parameters 2"=w493:T29, "Experiment Parameters.Stimulus"=w478:string)
            n264 = Unbundle By Name(w485) -> ("desaccading parameters.Impulse dir"=w488:bool)
            n265 = call-dynamic "Find first empty row.vi"("Excel Sheet in"=w476) -> ("Excel Sheet out"=w490:refnum<class "Data Analyser Report.lvclass">)  [unwired: 8 in, 2 out]
            n266 = call "Write Experiment Parameter.vi"("Experiment Parameters"=w493, "Data Analyser Reportin"=w490) -> ("Data Analyser Report out"=w492:refnum<class "Data Analyser Report.lvclass">)  [unwired: 9 in]
            n267 = case shown="True" w488 {
              tunnel: ["NEG" "POS"] -> w489
              frame False {
              }
              frame True {
              }
            }
            n268 = call "Write Eye and Eye Axis.vi"("Impulse Manager"=w471, "Data Analyser Report in"=w492) -> ("Data Analyser Report out"=w491:refnum<class "Data Analyser Report.lvclass">)  [unwired: 8 in, 1 out]
            n269 = call-poly "Write to Cell.vi"("Value"=w489, "Excel Sheet in"=w491) -> ("Excel Sheet out"=w479:refnum<class "Data Analyser Report.lvclass">)  [unwired: 9 in]
            n270 = call-poly "Write to Cell.vi"("Value"=w478, "Excel Sheet in"=w479) -> ("Excel Sheet out"=w480:refnum<class "Data Analyser Report.lvclass">)  [unwired: 9 in]
            n271 = call "Get Number of Impulses.vi"("Impulse Manager in"=w471) -> ("Number of impulses"=w472:i32)  [unwired: 8 in, 2 out]
            n272 = call-poly "Write to Cell.vi"("Value"=w472, "Excel Sheet in"=w480) -> ("Excel Sheet out"=w482:refnum<class "Data Analyser Report.lvclass">)  [unwired: 9 in]
            n273 = call-dynamic "Fit Result to String.vi"("Exponential Fit in"=w483) -> ("Array"=w481:string[])  [unwired: 8 in, 2 out]
            n274 = for {
              tunnel: w481 -> [w495] mode=indexing
              shift-right: [w494] -> w474
              shift-left: w482 -> [w496]
              n275 = call-poly "Write to Cell.vi"("Value"=w495, "Excel Sheet in"=w496) -> ("Excel Sheet out"=w494:refnum<class "Data Analyser Report.lvclass">)  [unwired: 9 in]
            }
            n276 = call "Write Exponential Sheet.vi"("Exponential"=w474, "Excel Logger in"=w475) -> ("Excel Logger out"=w473:refnum<class "Excel Logger.lvclass">)  [unwired: 8 in, 1 out]
            n277 = Bundle By Name(cluster=w487, "Excel Logger"=w473) -> (w486:T18)
          }
          frame "Head Impulse" {
            n278 = call "Get Head Impulse Sheet.vi"("Excel Logger in"=w505) -> ("Head Impulse"=w504:refnum<class "Data Analyser Report.lvclass">, "Excel Logger out"=w502:refnum<class "Excel Logger.lvclass">)  [unwired: 8 in, 1 out]
            n279 = Unbundle By Name(w513) -> ("Impulse Manager"=w500:refnum<class "Impulse Manager.lvclass">, "HI Fit"=w511:refnum<class "Head Impulse Fit.lvclass">)
            n280 = Unbundle By Name(w512) -> ("Experiment Parameters 2"=w521:T29, "Experiment Parameters.Stimulus"=w506:string)
            n281 = Unbundle By Name(w513) -> ("desaccading parameters.Impulse dir"=w516:bool)
            n282 = call-dynamic "Find first empty row.vi"("Excel Sheet in"=w504) -> ("Excel Sheet out"=w518:refnum<class "Data Analyser Report.lvclass">)  [unwired: 8 in, 2 out]
            n283 = call "Write Experiment Parameter.vi"("Experiment Parameters"=w521, "Data Analyser Reportin"=w518) -> ("Data Analyser Report out"=w520:refnum<class "Data Analyser Report.lvclass">)  [unwired: 9 in]
            n284 = case shown="True" w516 {
              tunnel: ["NEG" "POS"] -> w517
              frame False {
              }
              frame True {
              }
            }
            n285 = call "Write Eye and Eye Axis.vi"("Impulse Manager"=w500, "Data Analyser Report in"=w520) -> ("Data Analyser Report out"=w519:refnum<class "Data Analyser Report.lvclass">)  [unwired: 8 in, 1 out]
            n286 = call-poly "Write to Cell.vi"("Value"=w517, "Excel Sheet in"=w519) -> ("Excel Sheet out"=w507:refnum<class "Data Analyser Report.lvclass">)  [unwired: 9 in]
            n287 = call-poly "Write to Cell.vi"("Value"=w506, "Excel Sheet in"=w507) -> ("Excel Sheet out"=w508:refnum<class "Data Analyser Report.lvclass">)  [unwired: 9 in]
            n288 = call "Get Number of Impulses.vi"("Impulse Manager in"=w500) -> ("Number of impulses"=w499:i32)  [unwired: 8 in, 2 out]
            n289 = call-poly "Write to Cell.vi"("Value"=w499, "Excel Sheet in"=w508) -> ("Excel Sheet out"=w510:refnum<class "Data Analyser Report.lvclass">)  [unwired: 9 in]
            n290 = call-dynamic "Fit Result to String.vi"("Head Impulse Fit in"=w511) -> ("Array"=w509:string[])  [unwired: 8 in, 2 out]
            n291 = for {
              tunnel: w509 -> [w523] mode=indexing
              shift-right: [w522] -> w501
              shift-left: w510 -> [w524]
              n292 = call-poly "Write to Cell.vi"("Value"=w523, "Excel Sheet in"=w524) -> ("Excel Sheet out"=w522:refnum<class "Data Analyser Report.lvclass">)  [unwired: 9 in]
            }
            n293 = call "Write Head Impulse Sheet.vi"("Head Impulse"=w501, "Excel Logger in"=w502) -> ("Excel Logger out"=w503:refnum<class "Excel Logger.lvclass">)  [unwired: 8 in, 1 out]
            n294 = Bundle By Name(cluster=w515, "Excel Logger"=w503) -> (w514:T18)
          }
        }
      }
      frame "Stop" {
        n295 = Unbundle By Name(w533) -> ("Excel"=w530:T26, "Excel Logger"=w529:refnum<class "Excel Logger.lvclass">, "Impulse Data"=w527:T19)
        n296 = Bundle By Name(cluster=w532, "Excel"=w530) -> (w531:T1)
        n297 = call "Constructor Singleton.vi"("Enum"=enum16{"Init", "Update"}."Update", "Excel Logger.lvclass 2"=w529) -> ()  [unwired: 9 in, 1 out]
        n298 = call "Destructor.vi"("data value reference"=w527) -> ()  [unwired: 11 in]
      }
      frame "Update controls and variables" {
        n299 = Unbundle By Name(w564) -> ("Sine Fit"=w555:refnum<class "Sinusoidal Fit.lvclass">[], "Mean Fit"=w542:refnum<class "Mean Fit.lvclass">, "Exponential Fit"=w540:refnum<class "Exponential Fit.lvclass">, "HI Fit"=w537:refnum<class "Head Impulse Fit.lvclass">)
        n300 = call "GetFitValues.vi"("Mean Fit in"=w542) -> ("Mean Fit"=w541:T10)  [unwired: 8 in, 2 out]
        n301 = call "GetFitValues.vi"("Exponential Fit in"=w540) -> ("Response Parameters"=w538:T11, "Stimulus Parameters"=w539:T11)  [unwired: 7 in, 2 out]
        n302 = call "Get Fit Values.vi"("Head Impulse Fit in"=w537) -> ("Fit Data"=w536:T13)  [unwired: 8 in, 2 out]
        n303 = local write "Mean Fit"(w541) -> ()
        n304 = local write "Exp Stimulus"(w539) -> ()
        n305 = local write "Exp Response"(w538) -> ()
        n306 = local write "Head Impulse Fit Data"(w536) -> ()
        n307 = Index Array(array=w555) -> (element #1=w545:refnum<class "Sinusoidal Fit.lvclass">, element #2=w554:refnum<class "Sinusoidal Fit.lvclass">, element #3=w553:refnum<class "Sinusoidal Fit.lvclass">)  [unwired: 3 in]
        n308 = local read "Sine Fit Type"() -> (w544:enum16{"Normal Fit", "Halfwave Fit"})
        n309 = call-dynamic "Get Gain and Phase.vi"("Sinusoidal Fit in"=w554) -> ("Gain and Phase"=→"Positive Halfwave":T8, "Sinusoidal Fit out"=w561:refnum<class "Sinusoidal Fit.lvclass">)  [unwired: 8 in, 1 out]
        n310 = call-dynamic "Get Gain and Phase.vi"("Sinusoidal Fit in"=w553) -> ("Gain and Phase"=→"Negative Halfwave":T8, "Sinusoidal Fit out"=w558:refnum<class "Sinusoidal Fit.lvclass">)  [unwired: 8 in, 1 out]
        n311 = call-dynamic "Get Gain and Phase.vi"("Sinusoidal Fit in"=w545) -> ("Gain and Phase"=→"Normal Sine - Gain and Phase":T8, "Sinusoidal Fit out"=w549:refnum<class "Sinusoidal Fit.lvclass">)  [unwired: 8 in, 1 out]
        n312 = call-dynamic "Get Stimulus Coefficients.vi"("Sinusoidal Fit in"=w561) -> ("Coefficients"=→"Coefficients":T6, "Sinusoidal Fit out"=w560:refnum<class "Sinusoidal Fit.lvclass">)  [unwired: 8 in, 1 out]
        n313 = call-dynamic "Get Stimulus Coefficients.vi"("Sinusoidal Fit in"=w558) -> ("Coefficients"=→"Coefficients 2":T6, "Sinusoidal Fit out"=w557:refnum<class "Sinusoidal Fit.lvclass">)  [unwired: 8 in, 1 out]
        n314 = To Long Integer(number=w544) -> (32bit integer=w543:i32)
        n315 = call-dynamic "Get Stimulus Coefficients.vi"("Sinusoidal Fit in"=w549) -> ("Coefficients"=→"Normal Sine - Stimulus":T6, "Sinusoidal Fit out"=w548:refnum<class "Sinusoidal Fit.lvclass">)  [unwired: 8 in, 1 out]
        n316 = call-dynamic "Get Response Coefficients.vi"("Sinusoidal Fit in"=w560) -> ("Coefficients"=w552:T6)  [unwired: 8 in, 2 out]
        n317 = call-dynamic "Get Response Coefficients.vi"("Sinusoidal Fit in"=w557) -> ("Coefficients"=w551:T6)  [unwired: 8 in, 2 out]
        n318 = local write "Tab Control 2"(w543) -> ()
        n319 = call-dynamic "Get Response Coefficients.vi"("Sinusoidal Fit in"=w548) -> ("Coefficients"=w546:T6)  [unwired: 8 in, 2 out]
        n320 = local write "Pos HW Response"(w552) -> ()
        n321 = local write "Neg HW Response"(w551) -> ()
        n322 = local write "Normal Sine - Response"(w546) -> ()
      }
      frame "Generate Plot" {
        n323 = local read "Type of Analysis"() -> (w568:T17)
        n324 = case shown="\"Mean\", Default" w568 {
          tunnel: [w576 w577] -> w570
          frame "Mean", Default {
            w576 = T20[] [enum."Display Data"] items=["Quit", "Cycle Channels", "Generate Plot", "Analyse Data", "Save Image", "Polynomial Fit", "Open_Create Excel", "Excel find free A cell", "Panel Monitoring", "Save to Excel", "Initialize", "Extract Data", "Display Data", "Calculate Sinusoidal Gains", "Make Transient Fits & Equations", "Calculate Latency Fits", "Calculate Transient Ga 1 Gain", "Calculate Transient Ga 2 Gain", "Calculate Transient Gv Gain", "Stop", "Calculate Latency", "Calculate Exponential", "Calculate Mean", "Calculate Head Impulse", "Update controls and variables", "Save All Gain And Phase To Excel", "Calculate Impulse Latency", "Save Impulse Latency To Excel"] ("State Stack")
          }
          frame "Transient" {
            w577 = T20[] [enum."Make Transient Fits & Equations", enum."Display Data"] items=["Quit", "Cycle Channels", "Generate Plot", "Analyse Data", "Save Image", "Polynomial Fit", "Open_Create Excel", "Excel find free A cell", "Panel Monitoring", "Save to Excel", "Initialize", "Extract Data", "Display Data", "Calculate Sinusoidal Gains", "Make Transient Fits & Equations", "Calculate Latency Fits", "Calculate Transient Ga 1 Gain", "Calculate Transient Ga 2 Gain", "Calculate Transient Gv Gain", "Stop", "Calculate Latency", "Calculate Exponential", "Calculate Mean", "Calculate Head Impulse", "Update controls and variables", "Save All Gain And Phase To Excel", "Calculate Impulse Latency", "Save Impulse Latency To Excel"]  # State Stack
          }
        }
        n325 = Insert Into Array(array=w572, index=0, new element=w570) -> (w571:T20[])
      }
      frame "Cycle Channels" {
        w584 = T20[] [enum."Generate Plot", enum."Analyse Data"] items=["Quit", "Cycle Channels", "Generate Plot", "Analyse Data", "Save Image", "Polynomial Fit", "Open_Create Excel", "Excel find free A cell", "Panel Monitoring", "Save to Excel", "Initialize", "Extract Data", "Display Data", "Calculate Sinusoidal Gains", "Make Transient Fits & Equations", "Calculate Latency Fits", "Calculate Transient Ga 1 Gain", "Calculate Transient Ga 2 Gain", "Calculate Transient Gv Gain", "Stop", "Calculate Latency", "Calculate Exponential", "Calculate Mean", "Calculate Head Impulse", "Update controls and variables", "Save All Gain And Phase To Excel", "Calculate Impulse Latency", "Save Impulse Latency To Excel"]  # State Stack
        n326 = local read "Freeze Visibility On Channel Cycle"() -> (w578:bool)
        n327 = local read "Parameter Impuls Series"() -> (w585:T3)
        n328 = Array Size(array=w585) -> (size(s)=w586:i32)
        n329 = case shown="3.." w586 {
          tunnel: [w589 w594] -> w582
          tunnel: w585 -> [w589 w598]
          tunnel: w578 -> [_ w590]
          frame 0..2, Default {
            # "If one or tw (or no) channel is active"
          }
          frame 3.. {
            # "If 3 or more channels (e.g. left and right eye) circle eyes"
            n330 = Delete From Array(array=w598, index=0) -> (deleted portion=w596:T31, array with subset deleted=w593:T3)  [unwired: 1 in]
            n331 = Rotate 1D Array(1:w593, 2:1 ("n")) -> (0:w592:T3)
            n332 = case shown="False" w590 {
              tunnel: w593 -> [_ w602]
              tunnel: w592 -> [w599 w601]
              tunnel: [w599 w600] -> w591
              frame False {
                # "Keep cycled visibility."
              }
              frame True {
                # "Keep visibility from before channel cycling."
                n333 = for {
                  tunnel: w602 -> [w606] mode=indexing
                  tunnel: w601 -> [w605] mode=indexing
                  tunnel: [w604] -> w600 mode=indexing
                  n334 = Unbundle By Name(w606) -> ("Visible"=w603:bool)
                  n335 = Bundle By Name(cluster=w605, "Visible"=w603) -> (w604:T31)
                }
              }
            }
            n336 = Build Array (concatenate)(w596, w591) -> (w594:T3)
          }
        }
        n337 = Unbundle By Name(w580) -> ("Impulse Manager"=w583:refnum<class "Impulse Manager.lvclass">)
        n338 = call-dynamic "Set Channels.vi"("Channel Selector in"=w582, "Impulse Manager in"=w583) -> ("Impulse Manager out"=w581:refnum<class "Impulse Manager.lvclass">)  [unwired: 8 in, 1 out]
        n339 = Bundle By Name(cluster=w580, "Impulse Manager"=w581) -> (w579:T18)
        n340 = property on="Parameter Impuls Series" class="Arr (strict)"("Val(Sgnl)"=w582) -> ()  [unwired: 2 in, 2 out]
      }
      frame "Analyse Data" {
        w608 = T20[] [enum."Extract Data"] items=["Quit", "Cycle Channels", "Generate Plot", "Analyse Data", "Save Image", "Polynomial Fit", "Open_Create Excel", "Excel find free A cell", "Panel Monitoring", "Save to Excel", "Initialize", "Extract Data", "Display Data", "Calculate Sinusoidal Gains", "Make Transient Fits & Equations", "Calculate Latency Fits", "Calculate Transient Ga 1 Gain", "Calculate Transient Ga 2 Gain", "Calculate Transient Gv Gain", "Stop", "Calculate Latency", "Calculate Exponential", "Calculate Mean", "Calculate Head Impulse", "Update controls and variables", "Save All Gain And Phase To Excel", "Calculate Impulse Latency", "Save Impulse Latency To Excel"] ("element")
        w609 = T20[] [enum."Display Data", enum."Panel Monitoring"] items=["Quit", "Cycle Channels", "Generate Plot", "Analyse Data", "Save Image", "Polynomial Fit", "Open_Create Excel", "Excel find free A cell", "Panel Monitoring", "Save to Excel", "Initialize", "Extract Data", "Display Data", "Calculate Sinusoidal Gains", "Make Transient Fits & Equations", "Calculate Latency Fits", "Calculate Transient Ga 1 Gain", "Calculate Transient Ga 2 Gain", "Calculate Transient Gv Gain", "Stop", "Calculate Latency", "Calculate Exponential", "Calculate Mean", "Calculate Head Impulse", "Update controls and variables", "Save All Gain And Phase To Excel", "Calculate Impulse Latency", "Save Impulse Latency To Excel"] ("State Stack (out)")
        n341 = local read "Type of Analysis"() -> (w611:T17)
        n342 = case shown="\"Impulse Latency\"" w611 {
          tunnel: [w615 w616 w617 w618 w619 w620] -> w607
          frame "Sinusoidal", Default {
            w615 = T20[] [enum."Calculate Sinusoidal Gains"] items=["Quit", "Cycle Channels", "Generate Plot", "Analyse Data", "Save Image", "Polynomial Fit", "Open_Create Excel", "Excel find free A cell", "Panel Monitoring", "Save to Excel", "Initialize", "Extract Data", "Display Data", "Calculate Sinusoidal Gains", "Make Transient Fits & Equations", "Calculate Latency Fits", "Calculate Transient Ga 1 Gain", "Calculate Transient Ga 2 Gain", "Calculate Transient Gv Gain", "Stop", "Calculate Latency", "Calculate Exponential", "Calculate Mean", "Calculate Head Impulse", "Update controls and variables", "Save All Gain And Phase To Excel", "Calculate Impulse Latency", "Save Impulse Latency To Excel"] ("State Stack")
          }
          frame "Transient" {
            w616 = T20[] [enum."Calculate Latency Fits", enum."Calculate Latency", enum."Calculate Transient Ga 1 Gain", enum."Calculate Transient Ga 2 Gain", enum."Calculate Transient Gv Gain", enum."Make Transient Fits & Equations"] items=["Quit", "Cycle Channels", "Generate Plot", "Analyse Data", "Save Image", "Polynomial Fit", "Open_Create Excel", "Excel find free A cell", "Panel Monitoring", "Save to Excel", "Initialize", "Extract Data", "Display Data", "Calculate Sinusoidal Gains", "Make Transient Fits & Equations", "Calculate Latency Fits", "Calculate Transient Ga 1 Gain", "Calculate Transient Ga 2 Gain", "Calculate Transient Gv Gain", "Stop", "Calculate Latency", "Calculate Exponential", "Calculate Mean", "Calculate Head Impulse", "Update controls and variables", "Save All Gain And Phase To Excel", "Calculate Impulse Latency", "Save Impulse Latency To Excel"] ("State Stack")
          }
          frame "Mean" {
            w617 = T20[] [enum."Calculate Mean"] items=["Quit", "Cycle Channels", "Generate Plot", "Analyse Data", "Save Image", "Polynomial Fit", "Open_Create Excel", "Excel find free A cell", "Panel Monitoring", "Save to Excel", "Initialize", "Extract Data", "Display Data", "Calculate Sinusoidal Gains", "Make Transient Fits & Equations", "Calculate Latency Fits", "Calculate Transient Ga 1 Gain", "Calculate Transient Ga 2 Gain", "Calculate Transient Gv Gain", "Stop", "Calculate Latency", "Calculate Exponential", "Calculate Mean", "Calculate Head Impulse", "Update controls and variables", "Save All Gain And Phase To Excel", "Calculate Impulse Latency", "Save Impulse Latency To Excel"] ("State Stack")
          }
          frame "Exponential" {
            w618 = T20[] [enum."Calculate Exponential"] items=["Quit", "Cycle Channels", "Generate Plot", "Analyse Data", "Save Image", "Polynomial Fit", "Open_Create Excel", "Excel find free A cell", "Panel Monitoring", "Save to Excel", "Initialize", "Extract Data", "Display Data", "Calculate Sinusoidal Gains", "Make Transient Fits & Equations", "Calculate Latency Fits", "Calculate Transient Ga 1 Gain", "Calculate Transient Ga 2 Gain", "Calculate Transient Gv Gain", "Stop", "Calculate Latency", "Calculate Exponential", "Calculate Mean", "Calculate Head Impulse", "Update controls and variables", "Save All Gain And Phase To Excel", "Calculate Impulse Latency", "Save Impulse Latency To Excel"] ("State Stack")
          }
          frame "Head Impulse" {
            w619 = T20[] [enum."Calculate Head Impulse"] items=["Quit", "Cycle Channels", "Generate Plot", "Analyse Data", "Save Image", "Polynomial Fit", "Open_Create Excel", "Excel find free A cell", "Panel Monitoring", "Save to Excel", "Initialize", "Extract Data", "Display Data", "Calculate Sinusoidal Gains", "Make Transient Fits & Equations", "Calculate Latency Fits", "Calculate Transient Ga 1 Gain", "Calculate Transient Ga 2 Gain", "Calculate Transient Gv Gain", "Stop", "Calculate Latency", "Calculate Exponential", "Calculate Mean", "Calculate Head Impulse", "Update controls and variables", "Save All Gain And Phase To Excel", "Calculate Impulse Latency", "Save Impulse Latency To Excel"] ("State Stack")
          }
          frame "Impulse Latency" {
            w620 = T20[] [enum."Calculate Impulse Latency"] items=["Quit", "Cycle Channels", "Generate Plot", "Analyse Data", "Save Image", "Polynomial Fit", "Open_Create Excel", "Excel find free A cell", "Panel Monitoring", "Save to Excel", "Initialize", "Extract Data", "Display Data", "Calculate Sinusoidal Gains", "Make Transient Fits & Equations", "Calculate Latency Fits", "Calculate Transient Ga 1 Gain", "Calculate Transient Ga 2 Gain", "Calculate Transient Gv Gain", "Stop", "Calculate Latency", "Calculate Exponential", "Calculate Mean", "Calculate Head Impulse", "Update controls and variables", "Save All Gain And Phase To Excel", "Calculate Impulse Latency", "Save Impulse Latency To Excel"] ("State Stack")
          }
        }
        n343 = Build Array (concatenate)(w608, w607, w609) -> (w610:T20[])
      }
      frame "Save Image" {
        w628 = T20[] [enum."Panel Monitoring"] items=["Quit", "Cycle Channels", "Generate Plot", "Analyse Data", "Save Image", "Polynomial Fit", "Open_Create Excel", "Excel find free A cell", "Panel Monitoring", "Save to Excel", "Initialize", "Extract Data", "Display Data", "Calculate Sinusoidal Gains", "Make Transient Fits & Equations", "Calculate Latency Fits", "Calculate Transient Ga 1 Gain", "Calculate Transient Ga 2 Gain", "Calculate Transient Gv Gain", "Stop", "Calculate Latency", "Calculate Exponential", "Calculate Mean", "Calculate Head Impulse", "Update controls and variables", "Save All Gain And Phase To Excel", "Calculate Impulse Latency", "Save Impulse Latency To Excel"] ("State Stack (out)")
        n344 = local read "Type of Analysis"() -> (w621:T17)
        n345 = Unbundle By Name(w622) -> ("desaccading parameters.Impulse dir"=w627:bool)
        n346 = Unbundle By Name(w625) -> ("Image data path"=w626:path, "filename"=w623:string)
        n347 = case shown="\"Sinusoidal\", Default" w621 {
          tunnel: [w655 w681] -> w631
          tunnel: [w654 w680] -> w630
          tunnel: w627 -> [w642 _]
          tunnel: w622 -> [w641 w671]
          frame "Transient" {
            w668 = i16 2 ("precision (6)")
            n348 = Unbundle By Name(w641) -> ("Data File.Channel List"=w649:string[])
            n349 = local read "Parameter Impuls Series"() -> (w640:T3)
            n350 = Index Array(array=w640, index=1) -> (element=w651:T31)
            n351 = local read "Transient Gains"() -> (w653:T9)
            n352 = Unbundle By Name(w651) -> ("Channel"=w650:u16)
            n353 = case shown="False" w642 {
              tunnel: ["NEG" ("string") "POS" ("string")] -> w643
              frame False {
              }
              frame True {
              }
            }
            n354 = Unbundle By Name(w653) -> ("Ga"=w667:dbl, "Ga SD"=w666:dbl, "Gv"=w665:dbl, "Gv SD"=w664:dbl)
            n355 = Index Array(array=w649, index=w650) -> (element=w648:string)
            n356 = String Subset(string=w648, length (rest)=2 ("length (rest)")) -> (substring=w645:string)  [unwired: 1 in]
            n357 = Number To Fractional String(number=w667, precision (6)=w668) -> (F-format string=w663:string)  [unwired: 2 in]
            n358 = Number To Fractional String(number=w666, precision (6)=w668) -> (F-format string=w660:string)  [unwired: 2 in]
            n359 = Number To Fractional String(number=w665, precision (6)=w668) -> (F-format string=w658:string)  [unwired: 2 in]
            n360 = Number To Fractional String(number=w664, precision (6)=w668) -> (F-format string=w656:string)  [unwired: 2 in]
            n361 = Concatenate Strings(" -- " ("string"), w645, " -- Ga " ("string"), w663, " | " ("string"), w660) -> (w655:string)
            n362 = Concatenate Strings(" -- Gv " ("string"), w658, " | " ("string"), w656, " - " ("string"), w643) -> (w654:string)
          }
          frame "Sinusoidal", Default {
            n363 = Unbundle By Name(w671) -> ("Data File.Channel List"=w675:string[])
            n364 = local read "Parameter Impuls Series"() -> (w679:T3)
            n365 = Index Array(array=w679, index=1) -> (element=w677:T31)
            n366 = Unbundle By Name(w677) -> ("Channel"=w676:u16)
            n367 = Index Array(array=w675, index=w676) -> (element=w674:string)
            n368 = String Subset(string=w674, length (rest)=2 ("length (rest)")) -> (substring=w672:string)  [unwired: 1 in]
            n369 = disable-structure shown="Disabled" {
              disable-tunnel: [w686 _] -> w681
              disable-tunnel: [w685 _] -> w680
              disable-tunnel: w672 -> [w682 _]
              frame Disabled {
                w699 = i16 2 ("precision (6)")
                n370 = local read "Sinusoidal Fit Controls"() -> (w684:T5)
                n371 = Unbundle By Name(w684) -> ("Sinusoidal Response.Gain"=w698:dbl, "Gain and Phase.Gain SD"=w697:dbl, "Phase shift"=w696:dbl, "Phase shift SD"=w695:dbl)
                n372 = Number To Fractional String(number=w698, precision (6)=w699) -> (F-format string=w694:string)  [unwired: 2 in]
                n373 = Number To Fractional String(number=w697, precision (6)=w699) -> (F-format string=w691:string)  [unwired: 2 in]
                n374 = Number To Fractional String(number=w696, precision (6)=w699) -> (F-format string=w689:string)  [unwired: 2 in]
                n375 = Number To Fractional String(number=w695, precision (6)=w699) -> (F-format string=w687:string)  [unwired: 2 in]
                n376 = Concatenate Strings(" -- " ("string"), w682, " -- Gain " ("string"), w694, " | " ("string"), w691) -> (w686:string)
                n377 = Concatenate Strings(" -- Phase " ("string"), w689, " | " ("string"), w687) -> (w685:string)
              }
              frame Enabled {
              }
            }
          }
        }
        n378 = String To Path(string=w623) -> (path=w636:path)
        n379 = call <vilib>:"Get File Extension.vi"("file"=w636) -> ("filename without extension"=w633:string)  [unwired: 6 in, 4 out]
        n380 = Concatenate Strings(w633, w631, w630, ".png" ("string")) -> (w632:string)
        n381 = call "File Dialog"("start path"=w626, "default name"=w632) -> ("selected path"=w637:path, "cancelled"=w635:bool)  [unwired: 10 in, 2 out]
        n382 = invoke on="Impulse Trace" class="WFGraph (strict)" method="Get Image"("image depth"=24 ("Image Depth")) -> ("image data"=w634:T32)  [unwired: 5 in, 5 out]
        n383 = case shown="False" w635 {
          tunnel: w637 -> [w703 _]
          tunnel: w634 -> [w704 _]
          tunnel: w625 -> [w702 w705]
          tunnel: [w700 w705] -> w624
          frame False {
            n384 = call <vilib>:"Write PNG File.vi"("image data"=w704, "path to PNG file"=w703) -> ()  [unwired: 8 in, 2 out]
            n385 = Strip Path(path=w703) -> (stripped path=w701:path)  [unwired: 1 out]
            n386 = Bundle By Name(cluster=w702, "Image data path"=w701) -> (w700:T1)
          }
          frame True {
          }
        }
      }
      frame "Display Data" {
        n387 = Unbundle By Name(w724) -> ("Impulse Manager"=w722:refnum<class "Impulse Manager.lvclass">, "Graph Manager"=w720:refnum<class "Graph Manager.lvclass">, "Sine Fit"=w718:refnum<class "Sinusoidal Fit.lvclass">[], "Fitted Curves"=w717:dbl[][], "Mean Fit"=w711:refnum<class "Mean Fit.lvclass">, "Exponential Fit"=w710:refnum<class "Exponential Fit.lvclass">, "HI Fit"=w709:refnum<class "Head Impulse Fit.lvclass">)  [unwired: 1 out]
        n388 = disable-structure shown="Enabled" {
          disable-tunnel: [w731 w735] -> w708
          disable-tunnel: [w730 w735] -> w707
          frame Disabled {
            n389 = local read "Parameter Impuls Series"() -> (w734:T3)
            n390 = Index Array(array=w734) -> (element #1=w733:T31, element #2=w732:T31)  [unwired: 2 in]
            n391 = Unbundle By Name(w733) -> ("Invert"=w731:bool)
            n392 = Unbundle By Name(w732) -> ("Invert"=w730:bool)
          }
          frame Enabled {
            w735 = FALSE ("Invert")
          }
        }
        n393 = call-dynamic "Clear Graph.vi"("Graph Manager in"=w720) -> ("Graph Manager out"=w719:refnum<class "Graph Manager.lvclass">)  [unwired: 9 in, 1 out]
        n394 = local read "Type of Analysis"() -> (w712:T17)
        n395 = call-dynamic "Plot Impulses.vi"("Graph Manager"=w719, "Impulse Manager in"=w722) -> ("Graph Manager out"=w716:refnum<class "Graph Manager.lvclass">)  [unwired: 7 in, 2 out]
        n396 = call-dynamic "Set all channels Mean.vi"("Boolean"="Mean Traces", "Graph Manager in"=w716) -> ("Graph Manager out"=w715:refnum<class "Graph Manager.lvclass">)  [unwired: 8 in, 1 out]
        n397 = case shown="True" "Show Fit" {
          tunnel: [w736 w746] -> w706
          tunnel: w718 -> [_ w745]
          tunnel: w712 -> [_ w744]
          tunnel: w717 -> [_ w743]
          tunnel: w715 -> [w736 w742]
          tunnel: w711 -> [_ w741]
          tunnel: w710 -> [_ w740]
          tunnel: w709 -> [_ w739]
          tunnel: w708 -> [_ w738]
          tunnel: w707 -> [_ w737]
          frame False {
          }
          frame True {
            n398 = case shown="\"Sinusoidal\"" w744 {
              tunnel: w742 -> [w753 w767 w781 w811 w817]
              tunnel: [w749 w764 w780 w805 w816] -> w746
              tunnel: w745 -> [_ _ w779 _ _]
              tunnel: w743 -> [_ _ _ w810 _]
              tunnel: w741 -> [w752 _ _ _ _]
              tunnel: w740 -> [_ w763 _ _ _]
              tunnel: w739 -> [_ _ _ _ w818]
              tunnel: w738 -> [w747 w762 w776 _ w815]
              tunnel: w737 -> [w748 w761 w775 _ w814]
              frame "Mean", Default {
                n399 = call-dynamic "Plot.vi"("Response Inverted?"=w748, "Stimulus Inverted?"=w747, "Graph Manager.lvclass"=w753, "Sinusoidal Fit in"=w752) -> ("Channel IDs"=w750:i32[], "Graph Manager.lvclass 2"=w751:refnum<class "Graph Manager.lvclass">)  [unwired: 4 in, 2 out]
                n400 = for {
                  shift-right: [w754] -> w749
                  shift-left: w751 -> [w760]
                  tunnel: w750 -> [w759] mode=indexing
                  n401 = call-dynamic "Set Line Width.vi"("width"=u8 4, "Channel"=w759, "Graph Manager in"=w760) -> ("Channel out"=w756:i32, "Graph Manager out"=w757:refnum<class "Graph Manager.lvclass">)  [unwired: 6 in, 1 out]
                  n402 = call-dynamic "Set Line Style.vi"("Line Style"=T21."dashed short", "Channel"=w756, "Graph Manager in"=w757) -> ("Graph Manager out"=w754:refnum<class "Graph Manager.lvclass">)  [unwired: 6 in, 2 out]
                }
              }
              frame "Exponential" {
                n403 = call-dynamic "Plot.vi"("Response Inverted?"=w761, "Stimulus Inverted?"=w762, "Graph Manager.lvclass"=w767, "Sinusoidal Fit in"=w763) -> ("Channel IDs"=w765:i32[], "Graph Manager.lvclass 2"=w766:refnum<class "Graph Manager.lvclass">)  [unwired: 4 in, 2 out]
                n404 = for {
                  shift-right: [w768] -> w764
                  shift-left: w766 -> [w774]
                  tunnel: w765 -> [w773] mode=indexing
                  n405 = call-dynamic "Set Line Width.vi"("width"=u8 4, "Channel"=w773, "Graph Manager in"=w774) -> ("Channel out"=w770:i32, "Graph Manager out"=w771:refnum<class "Graph Manager.lvclass">)  [unwired: 6 in, 1 out]
                  n406 = call-dynamic "Set Line Style.vi"("Line Style"=T21."dashed short", "Channel"=w770, "Graph Manager in"=w771) -> ("Graph Manager out"=w768:refnum<class "Graph Manager.lvclass">)  [unwired: 6 in, 2 out]
                }
              }
              frame "Sinusoidal" {
                n407 = local read "Sine Fit Type"() -> (w777:enum16{"Normal Fit", "Halfwave Fit"})
                n408 = case shown="\"Normal Fit\", Default" w777 {
                  tunnel: w779 -> [w784 w788]
                  tunnel: [w785 w787] -> w778
                  frame "Normal Fit", Default {
                    n409 = Array Subset(array=w784, index=0, length=1) -> (w785:refnum<class "Sinusoidal Fit.lvclass">[])
                  }
                  frame "Halfwave Fit" {
                    n410 = Array Subset(array=w788, index=1) -> (w787:refnum<class "Sinusoidal Fit.lvclass">[])  [unwired: 1 in]
                  }
                }
                n411 = for {
                  tunnel: w778 -> [w791] mode=indexing
                  shift-right: [w794] -> w780
                  shift-left: w781 -> [w795]
                  tunnel: w776 -> [w790]
                  tunnel: w775 -> [w789]
                  n412 = call-dynamic "Plot.vi"("Response Inverted?"=w789, "Stimulus Inverted?"=w790, "Graph Manager.lvclass"=w795, "Sinusoidal Fit in"=w791) -> ("Channel IDs"=w792:i32[], "Graph Manager.lvclass 2"=w793:refnum<class "Graph Manager.lvclass">)  [unwired: 4 in, 2 out]
                  n413 = for {
                    shift-right: [w796] -> w794
                    shift-left: w793 -> [w802]
                    tunnel: w792 -> [w801] mode=indexing
                    n414 = call-dynamic "Set Line Width.vi"("width"=u8 4, "Channel"=w801, "Graph Manager in"=w802) -> ("Channel out"=w798:i32, "Graph Manager out"=w799:refnum<class "Graph Manager.lvclass">)  [unwired: 6 in, 1 out]
                    n415 = call-dynamic "Set Line Style.vi"("Line Style"=T21."dashed short", "Channel"=w798, "Graph Manager in"=w799) -> ("Graph Manager out"=w796:refnum<class "Graph Manager.lvclass">)  [unwired: 6 in, 2 out]
                  }
                }
              }
              frame "Transient" {
                n416 = call-dynamic "Add Channel Data.vi"("Channel Data"=w810, "Graph Manager in"=w811) -> ("Channel ID"=w808:i32, "Graph Manager out"=w809:refnum<class "Graph Manager.lvclass">)  [unwired: 7 in, 1 out]
                n417 = call-dynamic "Set Line Width.vi"("width"=u8 4, "Channel"=w808, "Graph Manager in"=w809) -> ("Channel out"=w804:i32, "Graph Manager out"=w806:refnum<class "Graph Manager.lvclass">)  [unwired: 6 in, 1 out]
                n418 = call-dynamic "Set Line Style.vi"("Line Style"=T21."dashed short", "Channel"=w804, "Graph Manager in"=w806) -> ("Graph Manager out"=w805:refnum<class "Graph Manager.lvclass">)  [unwired: 6 in, 2 out]
              }
              frame "Head Impulse" {
                n419 = call-dynamic "Plot.vi"("Response Inverted?"=w814, "Stimulus Inverted?"=w815, "Graph Manager.lvclass"=w817, "Sinusoidal Fit in"=w818) -> ("Channel IDs"=w812:i32[], "Graph Manager.lvclass 2"=w813:refnum<class "Graph Manager.lvclass">)  [unwired: 4 in, 2 out]
                n420 = for {
                  shift-right: [w819] -> w816
                  shift-left: w813 -> [w825]
                  tunnel: w812 -> [w824] mode=indexing
                  n421 = call-dynamic "Set Line Width.vi"("width"=u8 4, "Channel"=w824, "Graph Manager in"=w825) -> ("Channel out"=w821:i32, "Graph Manager out"=w822:refnum<class "Graph Manager.lvclass">)  [unwired: 6 in, 1 out]
                  n422 = call-dynamic "Set Line Style.vi"("Line Style"=T21."dashed short", "Channel"=w821, "Graph Manager in"=w822) -> ("Graph Manager out"=w819:refnum<class "Graph Manager.lvclass">)  [unwired: 6 in, 2 out]
                }
              }
            }
          }
        }
        n423 = Build Array (concatenate)(Data_Analysis_state."Update controls and variables" ("State (out)"), w727) -> (w725:T20[])
        n424 = call-dynamic "Redraw.vi"("Graph Manager in"=w706) -> ("Graph Manager out"=w721:refnum<class "Graph Manager.lvclass">)  [unwired: 9 in, 1 out]
        n425 = Bundle By Name(cluster=w724, "Graph Manager"=w721) -> (w723:T18)
      }
      frame "Extract Data" {
        n426 = Unbundle By Name(w847) -> ("Data File"=w838:T25, "Impulse Positions"=w839:T24, "desaccading parameters.Impulse dir"=w835:bool, "desaccading parameters.Impulse Plane 2"=w840:T28, "desacc"=w841:T27)
        n427 = local read "Parameter Impuls Series"() -> (w837:T3)
        n428 = local read "Interpolate"() -> (w834:bool)
        n429 = local read "Spline Parameter"() -> (w831:dbl)
        n430 = local read "Spline"() -> (w832:bool)
        n431 = local read "Trace Select"() -> (w833:i32)
        n432 = call "Couple Head Impulse Traces.vi"("Data Input"=w838, "Impulse Positions"=w839, "Trace Select"=w833, "Impulse Direction +ve?"=w835, "Impulse Plane"=w840, "Mean and STD"=TRUE ("Mean Traces"), "Plot Selection 2"=w837, "desacc"=w841, "Interpolate"=w834, "S-pline"=w832, "balance parameter (s-pline Parameter)"=w831) -> ("No Impulses"=w826:i32, "Mean and STD"=w844:dbl[][])  [unwired: 5 in, 2 out]
        n433 = Index Array "Stimulus"(array=w844, index (row)=1 ("Index (row)")) -> (element=w843:dbl[])  [unwired: 1 in]
        n434 = Index Array "Response"(array=w844, index (row)=4 ("Index (row)")) -> (element=w842:dbl[])  [unwired: 1 in]
        n435 = Bundle By Name(cluster=w847, "Stimulus"=w843, "Response"=w842, "Fit Calculated"=FALSE) -> (w829:T18)
        n436 = Bundle By Name(cluster=w828, "No. Imp"=w826) -> (w827:T1)
      }
      frame "Calculate Latency" {
        n437 = Unbundle By Name(w860) -> ("Transient Gains.Latency Stat."=w850:u16, "Transient Gains.Latency"=w852:u16, "Fit Calculated"=w858:bool)
        n438 = Equal?(x=w852, y=u16 2) -> (x = y?=w855:bool)
        n439 = Equal?(x=w858, y=FALSE) -> (x = y?=w856:bool)
        n440 = And(x=w855, y=w856) -> (x .and. y?=w854:bool)
        n441 = case shown="False" w854 {
          tunnel: [w864 0] -> w853
          tunnel: w852 -> [w864 _]
          frame False {
          }
          frame True {
          }
        }
        n442 = case shown="0" w853 {
          tunnel: w860 -> [w869 w1020 w1063]
          tunnel: [w867 w1015 w1062] -> w861
          tunnel: w860 -> [w868 w1019 w1061]
          tunnel: w850 -> [w866 _ _]
          frame 0 {
            n443 = case shown="1" w866 {
              tunnel: w869 -> [w928 w992]
              tunnel: w868 -> [w927 w973]
              tunnel: [w895 w971] -> w867
              frame 0, Default {
                w884 = 30.0  # Go back 30 ms
                w908 = 0 ("index")
                w913 = 0 ("index")
                # "Calculates onset and latency using the SD method.\nThis method uses the instantaneous mean and +sd traces. Onset is defined at the index where mean >= mean(mean) + n * mean(sd). Where mean() functions are evaluated over the initial quiet data. Quiet data is defined as 0 index to dmean/dt > 500."
                n444 = Unbundle By Name(w928) -> ("Data File"=w945:T25, "Impulse Positions"=w944:T24, "desaccading parameters.Impulse dir"=w929:bool, "Data File.Sample Rate"=w886:i32, "desaccading parameters.Impulse Plane 2"=w943:T28, "desacc"=w942:T27, "Transient Gains"=w939:T9)
                n445 = local read "Parameter Impuls Series"() -> (w946:T3)
                n446 = local read "Trace Select"() -> (w871:i32)
                n447 = local read "Interpolate"() -> (w872:bool)
                n448 = Divide(x=w886, y=1000 ("x")) -> (x/y=w885:dbl)
                n449 = Unbundle By Name(w939) -> ("TH/#SDs 2"=w938:dbl)
                n450 = Multiply(x=w884, y=w885) -> (x*y=w880:dbl)
                n451 = call "Couple Head Impulse Traces.vi"("Data Input"=w945, "Impulse Positions"=w944, "Trace Select"=w871, "Impulse Direction +ve?"=w929, "Impulse Plane"=w943, "Mean and STD"=TRUE ("Mean Traces"), "Plot Selection 2"=w946, "desacc"=w942, "Interpolate"=w872) -> ("Mean and STD"=w930:dbl[][])  [unwired: 7 in, 3 out]
                n452 = Index Array "Stimulus"(array=w930, index (row)=0 ("Index (row)")) -> (element=w936:dbl[])  [unwired: 1 in]
                n453 = Index Array "Stimulus"(array=w930, index (row)=1 ("Index (row)")) -> (element=w935:dbl[])  [unwired: 1 in]
                n454 = Index Array "Stimulus"(array=w930, index (row)=3 ("Index (row)")) -> (element=w933:dbl[])  [unwired: 1 in]
                n455 = Index Array "Stimulus"(array=w930, index (row)=4 ("Index (row)")) -> (element=w934:dbl[])  [unwired: 1 in]
                n456 = case shown="True" w929 {
                  tunnel: w936 -> [w956 w958]
                  tunnel: [w954 w958] -> w876
                  tunnel: w935 -> [w955 w957]
                  tunnel: [w953 w957] -> w875
                  frame False {
                    n457 = Negate(x=w956) -> (-x=w954:dbl[])
                    n458 = Negate(x=w955) -> (-x=w953:dbl[])
                  }
                  frame True {
                  }
                }
                n459 = case shown="True" w929 {
                  tunnel: w933 -> [w950 w952]
                  tunnel: [w948 w952] -> w877
                  tunnel: w934 -> [w949 w951]
                  tunnel: [w947 w951] -> w878
                  frame False {
                    n460 = Negate(x=w950) -> (-x=w948:dbl[])
                    n461 = Negate(x=w949) -> (-x=w947:dbl[])
                  }
                  frame True {
                  }
                }
                n462 = Subtract(x=w876, y=w875) -> (x-y=w915:dbl[])
                n463 = Subtract(x=w877, y=w878) -> (x-y=w906:dbl[])
                n464 = Absolute Value(x=w915) -> (abs(x)=w874:dbl[])
                n465 = Build Array(w875) -> (w925:dbl[][])
                n466 = Absolute Value(x=w906) -> (abs(x)=w873:dbl[])
                n467 = Build Array(w878) -> (w897:dbl[][])
                n468 = call "Differentiate 3D.vi"("Sample Rate 4"=w886, "Data (in)"=w925) -> ("Data (differentiated)"=w924:dbl[][])  [unwired: 3 in]
                n469 = call "Differentiate 3D.vi"("Sample Rate 4"=w886, "Data (in)"=w897) -> ("Data (differentiated)"=w898:dbl[][])  [unwired: 3 in]
                n470 = Index Array(array=w924, index (row)=0) -> (element=w918:dbl[])  [unwired: 1 in]
                n471 = Index Array(array=w898, index (row)=0) -> (element=w904:dbl[])  [unwired: 1 in]
                n472 = Divide(x=1000, y=w886) -> (x/y=w892:dbl)
                n473 = Threshold 1D Array(1:0 ("start index (0)"), 2:500.0 ("threshold y"), 3:w918) -> (0:w883:dbl)
                n474 = Threshold 1D Array(1:0 ("start index (0)"), 2:500.0 ("threshold y"), 3:w904) -> (0:w881:dbl)
                n475 = Subtract(x=w883, y=w880) -> (x-y=w879:dbl)
                n476 = Array Subset(array=w875, index=w913, length=w879) -> (w912:dbl[])
                n477 = Array Subset(array=w874, index=w913, length=w879) -> (w920:dbl[])
                n478 = call-poly <vilib>:"Mean.vi"("X"=w912) -> ("mean"=w911:dbl)  [unwired: 1 out]
                n479 = call-poly <vilib>:"Mean.vi"("X"=w920) -> ("mean"=w914:dbl)  [unwired: 1 out]
                n480 = Multiply(x=w914, y=w938) -> (x*y=w916:dbl)
                n481 = Add(x=w911, y=w916) -> (x+y=w917:dbl)
                n482 = Threshold 1D Array(1:0 ("start index (0)"), 2:w917, 3:w875) -> (0:w893:dbl)
                n483 = Subtract(x=w881, y=w880) -> (x-y=w882:dbl)
                n484 = Array Subset(array=w878, index=w908, length=w882) -> (w909:dbl[])
                n485 = Array Subset(array=w873, index=w908, length=w882) -> (w902:dbl[])
                n486 = call-poly <vilib>:"Mean.vi"("X"=w909) -> ("mean"=w910:dbl)  [unwired: 1 out]
                n487 = call-poly <vilib>:"Mean.vi"("X"=w902) -> ("mean"=w907:dbl)  [unwired: 1 out]
                n488 = Multiply(x=w907, y=w938) -> (x*y=w905:dbl)
                n489 = Add(x=w910, y=w905) -> (x+y=w896:dbl)
                n490 = Threshold 1D Array(1:0 ("start index (0)"), 2:w896, 3:w878) -> (0:w891:dbl)
                n491 = Multiply(x=w893, y=w892) -> (x*y=w889:dbl)
                n492 = Multiply(x=w892, y=w891) -> (x*y=w890:dbl)
                n493 = Subtract(x=w890, y=w889) -> (x-y=w926:dbl)
                n494 = Bundle By Name(cluster=w927, "Transient Gains.Stim.Onset"=w889, "Transient Gains.Response Onset"=w890, "Transient Gains.Latency (ms)"=w926, "Fit Calculated"=FALSE) -> (w895:T18)
                n495 = Unbundle By Name(w895) -> ("Transient Gains"=w894:T9)
                n496 = local write "Transient Gains"(w894) -> ()
              }
              frame 1 {
                w965 = 1000.0
                w984 = FALSE  # Mean and STD
                # "Summarise using mean & sd"
                # "Resp."
                # "Stim."
                # "Retreieve impulse data"
                # "Latency calculation for SD method using individual traces"
                n497 = Unbundle By Name(w992) -> ("Data File"=w991:T25, "Impulse Positions"=w990:T24, "desaccading parameters.Impulse dir"=w983:bool, "Data File.Sample Rate"=w977:i32, "desaccading parameters.Impulse Plane 2"=w987:T28, "desacc"=w986:T27, "Transient Gains.TH/#SDs 2"=w969:dbl)
                n498 = local read "Parameter Impuls Series"() -> (w985:T3)
                n499 = local read "Trace Select"() -> (w989:i32)
                n500 = local read "Interpolate"() -> (w988:bool)
                n501 = call "Couple Head Impulse Traces.vi"("Data Input"=w991, "Impulse Positions"=w990, "Trace Select"=w989, "Impulse Direction +ve?"=w983, "Impulse Plane"=w987, "Mean and STD"=w984, "Plot Selection 2"=w985, "desacc"=w986, "Interpolate"=w988) -> ("No Impulses"=w981:i32, "Impulses"=w982:dbl[][])  [unwired: 7 in, 2 out]
                n502 = case shown="True" w983 {
                  tunnel: w982 -> [w1001 w1002]
                  tunnel: [w1000 w1002] -> w979
                  frame False {
                    n503 = Negate(x=w1001) -> (-x=w1000:dbl[][])
                  }
                  frame True {
                  }
                }
                n504 = Array Subset(array=w979, length (row)=w981) -> (w980:dbl[][])  [unwired: 3 in]
                n505 = Array Subset(array=w979, index (row)=w981, length (row)=w981) -> (w978:dbl[][])  [unwired: 2 in]
                n506 = for {
                  tunnel: w980 -> [w999] mode=indexing
                  tunnel: w978 -> [w998] mode=indexing
                  tunnel: w977 -> [w997]
                  tunnel: [w996] -> w976 mode=indexing
                  tunnel: [w995] -> w974 mode=indexing
                  tunnel: [w994] -> w975 mode=indexing
                  tunnel: w969 -> [w993]
                  # "Calculate onset and latency for each individual trace"
                  n507 = call "Find Onset by SD.vi"("#SDs (3)"=w993, "Sample Rate (Hz)"=w997, "Data"=w999) -> ("Onset (s)"=w996:dbl)  [unwired: 7 in, 1 out]
                  n508 = call "Find Onset by SD.vi"("#SDs (3)"=w993, "Sample Rate (Hz)"=w997, "Data"=w998) -> ("Onset (s)"=w995:dbl)  [unwired: 7 in, 1 out]
                  n509 = Subtract(x=w995, y=w996) -> (x-y=w994:dbl)
                }
                n510 = call <userlib>:"Remove NaNs.vi"("Data in"=w976) -> ("Data Out"=w967:dbl[])  [unwired: 5 in, 1 out]
                n511 = call <userlib>:"Remove NaNs.vi"("Data in"=w974) -> ("Data Out"=w968:dbl[])  [unwired: 5 in, 1 out]
                n512 = call <userlib>:"Remove NaNs.vi"("Data in"=w975) -> ("Data Out"=w966:dbl[])  [unwired: 5 in, 1 out]
                n513 = Multiply(x=w967, y=w965) -> (x*y=w964:dbl[])
                n514 = Multiply(x=w966, y=w965) -> (x*y=w962:dbl[])
                n515 = Multiply(x=w968, y=w965) -> (x*y=w963:dbl[])
                n516 = call <vilib>:"Std Deviation and Variance.vi"("X"=w964) -> ("mean"=w961:dbl)  [unwired: 1 in, 2 out]
                n517 = call <vilib>:"Std Deviation and Variance.vi"("X"=w963) -> ("mean"=w960:dbl)  [unwired: 1 in, 2 out]
                n518 = call <vilib>:"Std Deviation and Variance.vi"("X"=w962) -> ("mean"=w959:dbl)  [unwired: 1 in, 2 out]
                n519 = Bundle By Name(cluster=w973, "Transient Gains.Stim.Onset"=w961, "Transient Gains.Response Onset"=w960, "Transient Gains.Latency (ms)"=w959, "Fit Calculated"=FALSE) -> (w971:T18)
                n520 = Unbundle By Name(w971) -> ("Transient Gains"=w970:T9)
                n521 = local write "Transient Gains"(w970) -> ()
              }
            }
          }
          frame 1 {
            n522 = Unbundle By Name(w1020) -> ("Data File"=w1038:T25, "Impulse Positions"=w1037:T24, "desaccading parameters.Impulse dir"=w1021:bool, "Data File.Sample Rate"=w1008:i32, "desaccading parameters.Impulse Plane 2"=w1036:T28, "desacc"=w1035:T27, "Transient Gains"=w1032:T9)
            n523 = local read "Parameter Impuls Series"() -> (w1039:T3)
            n524 = local read "Trace Select"() -> (w1006:i32)
            n525 = Unbundle By Name(w1032) -> ("TH/#SDs 2"=w1031:dbl)
            n526 = local read "Interpolate"() -> (w1007:bool)
            n527 = call "Couple Head Impulse Traces.vi"("Data Input"=w1038, "Impulse Positions"=w1037, "Trace Select"=w1006, "Impulse Direction +ve?"=w1021, "Impulse Plane"=w1036, "Mean and STD"=TRUE ("Mean Traces"), "Plot Selection 2"=w1039, "desacc"=w1035, "Interpolate"=w1007) -> ("Mean and STD"=w1005:dbl[][])  [unwired: 7 in, 3 out]
            n528 = Index Array "Stimulus"(array=w1005, index (row)=3 ("Index (row)")) -> (element=w1025:dbl[])  [unwired: 1 in]
            n529 = Index Array "Stimulus"(array=w1005, index (row)=0 ("Index (row)")) -> (element=w1029:dbl[])  [unwired: 1 in]
            n530 = Index Array "Stimulus"(array=w1005, index (row)=1 ("Index (row)")) -> (element=w1028:dbl[])  [unwired: 1 in]
            n531 = Index Array "Stimulus"(array=w1005, index (row)=4 ("Index (row)")) -> (element=w1026:dbl[])  [unwired: 1 in]
            n532 = case shown="True" w1021 {
              tunnel: w1029 -> [w1049 w1051]
              tunnel: [w1047 w1051] -> _
              tunnel: w1028 -> [w1048 w1050]
              tunnel: [w1046 w1050] -> w1027
              frame False {
                n533 = Negate(x=w1049) -> (-x=w1047:dbl[])
                n534 = Negate(x=w1048) -> (-x=w1046:dbl[])
              }
              frame True {
              }
            }
            n535 = case shown="True" w1021 {
              tunnel: w1025 -> [w1043 w1045]
              tunnel: [w1041 w1045] -> _
              tunnel: w1026 -> [w1042 w1044]
              tunnel: [w1040 w1044] -> w1022
              frame False {
                n536 = Negate(x=w1043) -> (-x=w1041:dbl[])
                n537 = Negate(x=w1042) -> (-x=w1040:dbl[])
              }
              frame True {
              }
            }
            n538 = Threshold 1D Array(1:0, 2:w1031, 3:w1027) -> (0:w1010:dbl)
            n539 = Threshold 1D Array(1:0, 2:w1031, 3:w1022) -> (0:w1013:dbl)
            n540 = Divide(x=1000.0, y=w1008) -> (x/y=w1011:dbl)
            n541 = Multiply(x=w1010, y=w1011) -> (x*y=w1004:dbl)
            n542 = Multiply(x=w1011, y=w1013) -> (x*y=w1012:dbl)
            n543 = Subtract(x=w1012, y=w1004) -> (x-y=w1018:dbl)
            n544 = Bundle By Name(cluster=w1019, "Fit Calculated"=FALSE, "Transient Gains.Stim.Onset"=w1004, "Transient Gains.Response Onset"=w1012, "Transient Gains.Latency (ms)"=w1018) -> (w1015:T18)
            n545 = Unbundle By Name(w1015) -> ("Transient Gains"=w1014:T9)
            n546 = local write "Transient Gains"(w1014) -> ()
          }
          frame 2, Default {
            w1056 = 1000.0 ("y")
            n547 = Unbundle By Name(w1063) -> ("Transient Gains.Line Fit Res Latency.Offset"=w1064:dbl, "Transient Gains.Line Fit Res Latency.Slope"=w1065:dbl, "Transient Gains.Line Fit Stim Latency.Offset"=w1066:dbl, "Transient Gains.Line Fit Stim Latency.Slope"=w1067:dbl)
            n548 = Negate(x=w1064) -> (-x=w1060:dbl)
            n549 = Negate(x=w1066) -> (-x=w1059:dbl)
            n550 = Divide(x=w1060, y=w1065) -> (x/y=w1057:dbl)
            n551 = Divide(x=w1059, y=w1067) -> (x/y=w1058:dbl)
            n552 = Multiply(x=w1057, y=w1056) -> (x*y=w1054:dbl)
            n553 = Multiply(x=w1058, y=w1056) -> (x*y=w1053:dbl)
            n554 = Subtract(x=w1054, y=w1053) -> (x-y=w1055:dbl)
            n555 = Bundle By Name(cluster=w1061, "Fit Calculated"=TRUE, "Transient Gains.Response Onset"=w1054, "Transient Gains.Stim.Onset"=w1053, "Transient Gains.Latency (ms)"=w1055) -> (w1062:T18)
            n556 = Unbundle By Name(w1062) -> ("Transient Gains"=w1068:T9)
            n557 = local write "Transient Gains"(w1068) -> ()
          }
        }
      }
      frame "Calculate Sinusoidal Gains" {
        (unwired) T34 [] ("Impulse Positions")
        n558 = Unbundle By Name(w1100) -> ("Impulse Manager"=w1076:refnum<class "Impulse Manager.lvclass">)
        n559 = call-dynamic "Get Sample Rate.vi"("Impulse Manager in"=w1076) -> ("Sample Rate"=w1091:i32, "Impulse Manager out"=w1090:refnum<class "Impulse Manager.lvclass">)  [unwired: 8 in, 1 out]
        n560 = call "Constructor.vi"("Sample Rate"=w1091) -> ("Sinusoidal Fit out"=w1089:refnum<class "Sinusoidal Fit.lvclass">)  [unwired: 10 in]
        n561 = call-dynamic "Set Frequency.vi"("Frequency"="Stimulus\nFrequency", "Sinusoidal Fit in"=w1089) -> ("Sinusoidal Fit out"=w1071:refnum<class "Sinusoidal Fit.lvclass">)  [unwired: 8 in, 1 out]
        n562 = call-dynamic "Get Data.vi"("index"=0, "Impulse Manager in"=w1090) -> ("Data out"=w1081:dbl[][])  [unwired: 6 in, 3 out]
        n563 = call-dynamic "Get Data.vi"("index"=1, "Impulse Manager in"=w1090) -> ("Impulse Positions"=w1069:T34, "Data out"=w1080:dbl[][])  [unwired: 6 in, 2 out]
        n564 = call "Write Impulse Positions.vi"("Impulse Positions"=w1069, "Abstract Fit in"=w1071) -> ("Abstract Fit out"=w1070:refnum<class "Sinusoidal Fit.lvclass">)  [unwired: 8 in, 1 out]
        n565 = call-dynamic "Advanced Fit.vi"("Sinusoidal Fit Controls.Stat."="Stat. Method", "Response"=w1080, "Stimulus"=w1081, "Sinusoidal Fit in"=w1070) -> ("Sinusoidal Fit out"=w1079:refnum<class "Sinusoidal Fit.lvclass">)  [unwired: 5 in, 2 out]
        n566 = call "Constructor with Reference Fit.vi"("Direction"=TRUE, "Reference Fit"=w1079) -> ("Halfwave Sinusoidal Fit out"=w1086:refnum<class "Halfwave Sinusoidal Fit.lvclass">)  [unwired: 9 in]
        n567 = call "Constructor with Reference Fit.vi"("Direction"=FALSE, "Reference Fit"=w1079) -> ("Halfwave Sinusoidal Fit out"=w1083:refnum<class "Halfwave Sinusoidal Fit.lvclass">)  [unwired: 9 in]
        n568 = call-dynamic "Advanced Fit.vi"("Offset"="Offset", "Sinusoidal Fit Controls.Stat."="Stat. Method", "Response"=w1080, "Stimulus"=w1081, "Halfwave Sinusoidal Fit in"=w1086) -> ("Halfwave Sinusoidal Fit out"=w1074:refnum<class "Halfwave Sinusoidal Fit.lvclass">)  [unwired: 4 in, 2 out]
        n569 = call-dynamic "Advanced Fit.vi"("Offset"="Offset", "Sinusoidal Fit Controls.Stat."="Stat. Method", "Response"=w1080, "Stimulus"=w1081, "Halfwave Sinusoidal Fit in"=w1083) -> ("Halfwave Sinusoidal Fit out"=w1082:refnum<class "Halfwave Sinusoidal Fit.lvclass">)  [unwired: 4 in, 2 out]
        n570 = call-dynamic "Get Response Coefficients.vi"("Sinusoidal Fit in"=w1074) -> ("Sinusoidal Fit out"=w1073:refnum<class "Halfwave Sinusoidal Fit.lvclass">)  [unwired: 8 in, 2 out]
        n571 = Build Array(w1079, w1073, w1082) -> (w1084:refnum<class "Sinusoidal Fit.lvclass">[])
        n572 = Bundle By Name(cluster=w1100, "Sine Fit"=w1084) -> (w1095:T18)
        n573 = Unbundle By Name(w1095) -> ("Sinusoidal Fit Controls.Gain and Phase.Gain"=w1098:dbl, "Sinusoidal Fit Controls.Gain and Phase.Phase"=w1097:dbl)
        n574 = call "limit phase to 180 degrees.vi"("enable"="Limit Phase to 180 degrees (negative gains!)", "phase in"=w1097, "gain in"=w1098) -> ("phase out"=w1093:dbl, "gain out"=w1096:dbl)  [unwired: 7 in]
        n575 = Bundle By Name(cluster=w1095, "Sinusoidal Fit Controls.Gain and Phase.Gain"=w1096, "Sinusoidal Fit Controls.Gain and Phase.Phase"=w1093) -> (w1094:T18)
      }
      frame "Calculate Transient Ga 1 Gain" {
        n576 = Unbundle By Name(w1116) -> ("Fit Calculated"=w1107:bool, "Transient Gains.Snap Cursor"=w1121:u16, "Transient Gains.Ga Window (early)"=w1106:u16, "Transient Gains.Stim.Onset"=w1127:dbl, "Data File.Sample Rate"=w1115:i32, "Transient Gains.Ga Stat."=w1114:u16, "Transient Gains.Latency"=w1111:u16, "Transient Gains.GA1 desaccading"=w1104:bool)
        n577 = Equal?(x=u16 1, y=w1121) -> (x = y?=w1119:bool)
        n578 = case shown="False" w1107 {
          tunnel: [u16 6 ("Ga Window") w1137] -> w1105
          tunnel: w1106 -> [_ w1137]
          frame False {
          }
          frame True {
          }
        }
        n579 = Reciprocal(x=w1115) -> (1/x=w1125:dbl)
        n580 = case shown="1" w1105 {
          tunnel: [w1402 w1409 w1414 w1419 w1424 w1429 w1434] -> w1108
          tunnel: [w1403 w1408 w1413 w1418 w1423 w1428 w1433] -> w1109
          tunnel: w1127 -> [_ w1410 w1415 w1420 w1425 w1430 w1435]
          frame 0, Default {
            n581 = stacked-sequence {
              tunnel: [_ w1406] -> w1403
              tunnel: [w1404 _] -> w1402
              frame #0 {
                n582 = property on="Impulse Trace" class="WFGraph (strict)"("Active Cursor"=u32 0) -> ("Cursor.Cursor Position:Cursor X"=w1404:dbl)  [unwired: 2 in, 2 out]
              }
              frame #1 {
                n583 = property on="Impulse Trace" class="WFGraph (strict)"("Active Cursor"=u32 1) -> ("Cursor.Cursor Position:Cursor X"=w1406:dbl)  [unwired: 2 in, 2 out]
              }
            }
          }
          frame 1 {
            n584 = Add(x=w1410, y=10.0) -> (x+y=w1408:dbl)
            n585 = Add(x=w1408, y=10.0) -> (x+y=w1409:dbl)
          }
          frame 2 {
            n586 = Add(x=w1415, y=20.0) -> (x+y=w1413:dbl)
            n587 = Add(x=w1413, y=10.0) -> (x+y=w1414:dbl)
          }
          frame 3 {
            n588 = Add(x=w1420, y=30.0) -> (x+y=w1418:dbl)
            n589 = Add(x=w1418, y=10.0) -> (x+y=w1419:dbl)
          }
          frame 4 {
            n590 = Add(x=w1425, y=40.0) -> (x+y=w1423:dbl)
            n591 = Add(x=w1423, y=10.0) -> (x+y=w1424:dbl)
          }
          frame 5 {
            n592 = Add(x=w1430, y=20.0) -> (x+y=w1428:dbl)
            n593 = Add(x=w1428, y=20.0) -> (x+y=w1429:dbl)
          }
          frame 6 {
            n594 = Add(x=w1435, y=10.0) -> (x+y=w1433:dbl)
            n595 = Add(x=w1433, y=20.0) -> (x+y=w1434:dbl)
          }
        }
        n596 = Divide(x=w1115, y=1000.0) -> (x/y=w1126:dbl)
        n597 = Multiply(x=w1109, y=w1126) -> (x*y=w1122:dbl)
        n598 = Multiply(x=w1108, y=w1126) -> (x*y=w1123:dbl)
        n599 = case shown="False" w1119 {
          tunnel: w1108 -> [_ w1397]
          tunnel: w1109 -> [_ w1396]
          frame False {
          }
          frame True {
            n600 = stacked-sequence {
              tunnel: w1397 -> [w1398 _]
              tunnel: w1396 -> [_ w1400]
              frame #0 {
                n601 = property on="Impulse Trace" class="WFGraph (strict)"("Cursor.Cursor Position:Cursor X"=w1398, "Active Cursor"=u32 0) -> ()  [unwired: 2 in, 2 out]
              }
              frame #1 {
                n602 = property on="Impulse Trace" class="WFGraph (strict)"("Cursor.Cursor Position:Cursor X"=w1400, "Active Cursor"=u32 1) -> ()  [unwired: 2 in, 2 out]
              }
            }
          }
        }
        n603 = Subtract(x=w1123, y=w1122) -> (x-y=w1124:dbl)
        n604 = To Long Integer(number=w1122) -> (32bit integer=w1128:i32)
        n605 = To Long Integer(number=w1124) -> (32bit integer=w1129:i32)
        n606 = case shown="3" w1114 {
          tunnel: [w1168 w1207 w1276 w1346] -> w1132
          tunnel: [w1167 w1205 w1276 w1346] -> w1130
          tunnel: w1129 -> [w1166 w1211 w1282 w1352]
          tunnel: w1128 -> [w1165 w1210 w1281 w1351]
          tunnel: w1125 -> [w1164 w1212 w1283 w1353]
          tunnel: [w1159 w1204 w1276 w1346] -> w1118
          tunnel: [w1158 w1206 w1276 w1346] -> w1117
          tunnel: w1116 -> [w1160 w1221 w1292 w1362]
          tunnel: [w1157 w1209 w1280 w1350] -> w1113
          tunnel: [w1155 w1208 w1279 w1349] -> w1112
          tunnel: w1111 -> [_ _ w1275 w1345]
          tunnel: [TRUE TRUE FALSE FALSE] -> w1110
          tunnel: w1104 -> [_ w1194 w1270 w1340]
          frame 0, Default {
            w1156 = 0.0 ("standard deviation")
            # "Analysis of Mean Trace"
            n607 = Unbundle By Name(w1160) -> ("Stimulus"=w1152:dbl[], "Response"=w1153:dbl[])
            n608 = for {
              tunnel: w1164 -> [w1193]
              tunnel: [w1191] -> w1151 mode=indexing
              tunnel: w1153 -> [_] mode=indexing
              i -> [w1190]
              n609 = Multiply(x=w1193, y=w1190) -> (x*y=w1189:dbl)
              n610 = Build Array(1.0 ("Input Element"), w1189) -> (w1191:dbl[])
            }
            n611 = Array Subset(array=w1153, index=w1165, length=w1166) -> (w1162:dbl[])
            n612 = Array Subset(array=w1152, index=w1165, length=w1166) -> (w1163:dbl[])
            n613 = Array Subset(array=w1151, index (row)=w1165, length (row)=w1166) -> (w1161:dbl[][])  [unwired: 2 in]
            n614 = disable-structure shown="Enabled" {
              disable-tunnel: [w1181 w1186] -> w1168
              disable-tunnel: [w1180 w1184] -> w1167
              disable-tunnel: w1163 -> [w1175 w1188]
              disable-tunnel: w1162 -> [w1174 w1187]
              disable-tunnel: w1161 -> [w1173 w1182]
              disable-tunnel: [w1170 w1183] -> w1159
              disable-tunnel: [w1169 w1185] -> w1158
              frame Disabled {
                n615 = call <vilib>:"General LS Linear Fit (obs).vi"("H"=w1173, "Y"=w1175) -> ("Coefficients"=w1172:dbl[])  [unwired: 3 in, 4 out]
                n616 = call <vilib>:"General LS Linear Fit (obs).vi"("H"=w1173, "Y"=w1174) -> ("Coefficients"=w1171:dbl[])  [unwired: 3 in, 4 out]
                n617 = Index Array(array=w1172, index=0 ("Index")) -> (element=w1180:dbl)
                n618 = Index Array(array=w1172, index=1 ("Index")) -> (element=w1170:dbl)
                n619 = Index Array(array=w1171, index=0 ("Index")) -> (element=w1181:dbl)
                n620 = Index Array(array=w1171, index=1 ("Index")) -> (element=w1169:dbl)
              }
              frame Enabled {
                n621 = call "linear fit NaN.vi"("Array 2"=w1182, "Array"=w1188) -> ("sloap"=w1183:dbl, "intercept"=w1184:dbl)  [unwired: 2 in]
                n622 = call "linear fit NaN.vi"("Array 2"=w1182, "Array"=w1187) -> ("sloap"=w1185:dbl, "intercept"=w1186:dbl)  [unwired: 2 in]
              }
            }
            n623 = Divide(x=w1158, y=w1159) -> (x/y=w1157:dbl)
            n624 = Divide(x=w1156, y=w1156) -> (x/y=w1155:dbl)
          }
          frame 1 {
            n625 = Unbundle By Name(w1221) -> ("Data File"=w1226:T25, "Impulse Positions"=w1225:T24, "desaccading parameters.Impulse dir"=w1224:bool, "desaccading parameters.Impulse Plane 2"=w1223:T28, "desacc"=w1222:T27)
            n626 = local read "Parameter Impuls Series"() -> (w1219:T3)
            n627 = Array Size(array=w1219) -> (size(s)=w1214:i32)
            n628 = local read "Trace Select"() -> (w1200:i32)
            n629 = local read "Interpolate"() -> (w1201:bool)
            n630 = call "Couple Head Impulse Traces.vi"("Data Input"=w1226, "Impulse Positions"=w1225, "Trace Select"=w1200, "Impulse Direction +ve?"=w1224, "Impulse Plane"=w1223, "Mean and STD"=FALSE ("Mean Traces"), "Plot Selection 2"=w1219, "desacc"=w1222, "Interpolate"=w1201, "desacc."=TRUE, "man. desacc.."=w1194) -> ("Impulses"=w1218:dbl[][])  [unwired: 5 in, 3 out]
            n631 = Array Size(array=w1218) -> (size(s)=w1217:i32[])
            n632 = Index Array(array=w1217, index=0) -> (element=w1215:i32)
            n633 = Quotient & Remainder(x=w1215, y=w1214) -> (floor(x/y)=w1213:i32)  [unwired: 1 out]
            n634 = for {
              N: w1213 -> [w1241]
              tunnel: w1218 -> [w1232]
              tunnel: w1212 -> [w1240]
              tunnel: w1211 -> [w1239]
              tunnel: w1210 -> [w1238]
              tunnel: [w1237] -> w1196 mode=indexing
              tunnel: [w1236] -> w1198 mode=indexing
              tunnel: [w1235] -> w1197 mode=indexing
              tunnel: [w1234] -> w1199 mode=indexing
              i -> [w1242]
              n635 = Add(x=w1241, y=w1242) -> (x+y=w1243:i32)
              n636 = Index Array(array=w1232, index (row)=w1242) -> (element=w1229:dbl[])  [unwired: 1 in]
              n637 = Index Array(array=w1232, index (row)=w1243) -> (element=w1230:dbl[])  [unwired: 1 in]
              n638 = for {
                tunnel: w1240 -> [w1268]
                tunnel: [w1266] -> w1228 mode=indexing
                tunnel: w1230 -> [_] mode=indexing
                i -> [w1265]
                n639 = Multiply(x=w1268, y=w1265) -> (x*y=w1264:dbl)
                n640 = Build Array(1.0 ("Input Element"), w1264) -> (w1266:dbl[])
              }
              n641 = Array Subset(array=w1230, index=w1238, length=w1239) -> (w1231:dbl[])
              n642 = Array Subset(array=w1229, index=w1238, length=w1239) -> (w1233:dbl[])
              n643 = Array Subset(array=w1228, index (row)=w1238, length (row)=w1239) -> (w1227:dbl[][])  [unwired: 2 in]
              n644 = disable-structure shown="Enabled" {
                disable-tunnel: [w1250 w1258] -> w1237
                disable-tunnel: [w1249 w1259] -> w1236
                disable-tunnel: [w1248 w1260] -> w1235
                disable-tunnel: [w1247 w1261] -> w1234
                disable-tunnel: w1227 -> [w1246 _]
                disable-tunnel: w1233 -> [w1245 w1263]
                disable-tunnel: w1231 -> [w1244 w1262]
                disable-tunnel: w1227 -> [_ w1257]
                frame Disabled {
                  n645 = call <vilib>:"General LS Linear Fit (obs).vi"("H"=w1246, "Y"=w1245) -> ("Coefficients"=w1252:dbl[])  [unwired: 3 in, 4 out]
                  n646 = call <vilib>:"General LS Linear Fit (obs).vi"("H"=w1246, "Y"=w1244) -> ("Coefficients"=w1251:dbl[])  [unwired: 3 in, 4 out]
                  n647 = Index Array(array=w1252, index=0 ("Index")) -> (element=w1249:dbl)
                  n648 = Index Array(array=w1252, index=1 ("Index")) -> (element=w1250:dbl)
                  n649 = Index Array(array=w1251, index=0 ("Index")) -> (element=w1247:dbl)
                  n650 = Index Array(array=w1251, index=1 ("Index")) -> (element=w1248:dbl)
                }
                frame Enabled {
                  n651 = call "linear fit NaN.vi"("Array 2"=w1257, "Array"=w1262) -> ("sloap"=w1260:dbl, "intercept"=w1261:dbl)  [unwired: 2 in]
                  n652 = call "linear fit NaN.vi"("Array 2"=w1257, "Array"=w1263) -> ("sloap"=w1258:dbl, "intercept"=w1259:dbl)  [unwired: 2 in]
                }
              }
            }
            n653 = Divide(x=w1197, y=w1196) -> (x/y=w1203:dbl[])
            n654 = call "standard deviation NaN.vi"("Array"=w1203) -> ("standard deviation"=w1208:dbl, "mean"=w1209:dbl)  [unwired: 2 in, 1 out]
            n655 = call "mean_nan.vi"("Array"=w1199) -> ("Mean"=w1207:dbl)  [unwired: 10 in]
            n656 = call "mean_nan.vi"("Array"=w1197) -> ("Mean"=w1206:dbl)  [unwired: 10 in]
            n657 = call "mean_nan.vi"("Array"=w1198) -> ("Mean"=w1205:dbl)  [unwired: 10 in]
            n658 = call "mean_nan.vi"("Array"=w1196) -> ("Mean"=w1204:dbl)  [unwired: 10 in]
          }
          frame 2 {
            w1277 = 0.0 ("standard deviation")
            n659 = Unbundle By Name(w1292) -> ("Data File"=w1296:T25, "Impulse Positions"=w1295:T24, "desaccading parameters.Impulse dir"=w1294:bool, "desaccading parameters.Impulse Plane 2"=w1293:T28, "desacc"=w1269:T27)
            n660 = local read "Parameter Impuls Series"() -> (w1290:T3)
            n661 = local read "Interpolate"() -> (w1273:bool)
            n662 = Array Size(array=w1290) -> (size(s)=w1285:i32)
            n663 = local read "Trace Select"() -> (w1272:i32)
            n664 = call "Couple Head Impulse Traces.vi"("Data Input"=w1296, "Impulse Positions"=w1295, "Trace Select"=w1272, "Impulse Direction +ve?"=w1294, "Impulse Plane"=w1293, "Mean and STD"=FALSE ("Mean Traces"), "Plot Selection 2"=w1290, "desacc"=w1269, "Interpolate"=w1273, "desacc."=FALSE, "man. desacc.."=w1270) -> ("Impulses"=w1289:dbl[][])  [unwired: 5 in, 3 out]
            n665 = Array Size(array=w1289) -> (size(s)=w1288:i32[])
            n666 = Index Array(array=w1288, index=0) -> (element=w1286:i32)
            n667 = Quotient & Remainder(x=w1286, y=w1285) -> (floor(x/y)=w1284:i32)  [unwired: 1 out]
            n668 = for {
              N: w1284 -> [w1315]
              tunnel: w1289 -> [w1318]
              tunnel: w1283 -> [w1311]
              tunnel: w1282 -> [w1313]
              tunnel: w1281 -> [w1314]
              tunnel: [w1312] -> w1278 mode=indexing
              tunnel: w1275 -> [w1307]
              i -> [w1316]
              n669 = Add(x=w1315, y=w1316) -> (x+y=w1317:i32)
              n670 = Index Array(array=w1318, index (row)=w1316) -> (element=w1297:dbl[])  [unwired: 1 in]
              n671 = Index Array(array=w1318, index (row)=w1317) -> (element=w1298:dbl[])  [unwired: 1 in]
              n672 = for {
                tunnel: w1311 -> [w1339]
                tunnel: [w1337] -> _ mode=indexing
                tunnel: w1298 -> [_] mode=indexing
                i -> [w1336]
                n673 = Multiply(x=w1339, y=w1336) -> (x*y=w1335:dbl)
                n674 = Build Array(1.0 ("Input Element"), w1335) -> (w1337:dbl[])
              }
              n675 = Reciprocal(x=w1311) -> (1/x=w1310:dbl)
              n676 = Divide(x=w1310, y=1000.0) -> (x/y=w1308:dbl)
              n677 = Multiply(x=w1307, y=w1308) -> (x*y=w1306:dbl)
              n678 = Round To Nearest(number=w1306) -> (nearest integer value=w1302:dbl)
              n679 = Array Subset(array=w1298, index=w1314, length=w1313) -> (w1304:dbl[])
              n680 = Array Subset(array=w1297, index=w1314, length=w1313) -> (w1303:dbl[])
              n681 = Greater Or Equal To 0?(x=w1302) -> (x >= 0?=w1305:bool)
              n682 = case shown="True" w1305 {
                tunnel: w1303 -> [w1320 w1329]
                tunnel: w1304 -> [w1326 w1330]
                tunnel: w1302 -> [w1323 w1332]
                tunnel: [w1321 w1328] -> w1300
                tunnel: [w1319 w1327] -> w1299
                frame True {
                  n683 = Array Size(array=w1326) -> (size(s)=w1324:i32)
                  n684 = Subtract(x=w1324, y=w1323) -> (x-y=w1322:dbl)
                  n685 = Array Subset(array=w1326, index=w1323, length=w1324) -> (w1321:dbl[])
                  n686 = Array Subset(array=w1320, index=0, length=w1322) -> (w1319:dbl[])
                }
                frame False {
                  n687 = Array Size(array=w1330) -> (size(s)=w1333:i32)
                  n688 = Subtract(x=w1333, y=w1332) -> (x-y=w1331:dbl)
                  n689 = Array Subset(array=w1329, index=w1332, length=w1333) -> (w1327:dbl[])
                  n690 = Array Subset(array=w1330, index=0, length=w1331) -> (w1328:dbl[])
                }
              }
              n691 = Divide(x=w1300, y=w1299) -> (x/y=w1301:dbl[])
              n692 = call "mean_nan.vi"("Array"=w1301) -> ("Mean"=w1312:dbl)  [unwired: 10 in]
            }
            n693 = call "standard deviation NaN.vi"("Array"=w1278) -> ("standard deviation"=w1279:dbl, "mean"=w1280:dbl)  [unwired: 2 in, 1 out]
            n694 = Divide(x=w1277, y=w1277) -> (x/y=w1276:dbl)
          }
          frame 3 {
            w1347 = 0.0 ("standard deviation")
            n695 = Unbundle By Name(w1362) -> ("Data File"=w1367:T25, "Impulse Positions"=w1366:T24, "desaccading parameters.Impulse dir"=w1365:bool, "desaccading parameters.Impulse Plane 2"=w1364:T28, "desacc"=w1363:T27)
            n696 = local read "Parameter Impuls Series"() -> (w1360:T3)
            n697 = local read "Trace Select"() -> (w1342:i32)
            n698 = call "Couple Head Impulse Traces.vi"("Data Input"=w1367, "Impulse Positions"=w1366, "Trace Select"=w1342, "Impulse Direction +ve?"=w1365, "Impulse Plane"=w1364, "Mean and STD"=FALSE ("Mean Traces"), "Plot Selection 2"=w1360, "desacc"=w1363, "Interpolate"="Interpolate", "desacc."=FALSE, "man. desacc.."=w1340) -> ("Impulses"=w1359:dbl[][])  [unwired: 5 in, 3 out]
            n699 = Array Size(array=w1360) -> (size(s)=w1355:i32)
            n700 = Array Size(array=w1359) -> (size(s)=w1358:i32[])
            n701 = Index Array(array=w1358, index=0) -> (element=w1356:i32)
            n702 = Quotient & Remainder(x=w1356, y=w1355) -> (floor(x/y)=w1354:i32)  [unwired: 1 out]
            n703 = for {
              N: w1354 -> [w1387]
              tunnel: w1359 -> [w1390]
              tunnel: w1353 -> [w1378]
              tunnel: w1352 -> [w1380]
              tunnel: w1351 -> [w1381]
              tunnel: [w1379] -> w1348 mode=indexing
              tunnel: w1345 -> [_]
              i -> [w1388]
              (unwired) 1000.0 ("y")
              n704 = Add(x=w1387, y=w1388) -> (x+y=w1389:i32)
              n705 = Index Array(array=w1390, index (row)=w1388) -> (element=w1382:dbl[])  [unwired: 1 in]
              n706 = Index Array(array=w1390, index (row)=w1389) -> (element=w1383:dbl[])  [unwired: 1 in]
              n707 = for {
                tunnel: w1378 -> [w1395]
                tunnel: [w1393] -> w1386 mode=indexing
                tunnel: w1383 -> [_] mode=indexing
                i -> [w1392]
                n708 = Multiply(x=w1395, y=w1392) -> (x*y=w1391:dbl)
                n709 = Build Array(1.0 ("Input Element"), w1391) -> (w1393:dbl[])
              }
              n710 = call <userlib>:"Remove NaNs.vi"("Sinusoid"=w1386, "Response"=w1383, "Stimulus"=w1382) -> ("Response (out)"=w1384:dbl[], "Stimulus (out)"=w1385:dbl[])  [unwired: 1 out]
              n711 = Reciprocal(x=w1378) -> (1/x=w1371:dbl)
              n712 = Array Subset(array=w1384, index=w1381, length=w1380) -> (w1373:dbl[])
              n713 = Array Subset(array=w1385, index=w1381, length=w1380) -> (w1372:dbl[])
              n714 = Build Array(w1373, w1372) -> (w1376:dbl[][])
              n715 = call "Differentiate 3D.vi"("Sample Rate 4"=w1371, "Data (in)"=w1376) -> ("Data (differentiated)"=w1368:dbl[][])  [unwired: 3 in]
              n716 = Index Array(array=w1368, index (row)=0) -> (element=w1369:dbl[])  [unwired: 1 in]
              n717 = Index Array(array=w1368, index (row)=1) -> (element=w1370:dbl[])  [unwired: 1 in]
              n718 = Divide(x=w1369, y=w1370) -> (x/y=w1377:dbl[])
              n719 = call-poly <vilib>:"Mean.vi"("X"=w1377) -> ("mean"=w1379:dbl)  [unwired: 1 out]
            }
            n720 = call <vilib>:"Std Deviation and Variance.vi"("X"=w1348) -> ("mean"=w1350:dbl, "standard deviation"=w1349:dbl)  [unwired: 1 in, 1 out]
            n721 = Divide(x=w1347, y=w1347) -> (x/y=w1346:dbl)
          }
        }
        n722 = case shown="True" w1110 {
          tunnel: [w1146 w1150] -> w1133
          tunnel: w1132 -> [w1145 _]
          tunnel: w1130 -> [w1144 _]
          tunnel: w1118 -> [w1143 _]
          tunnel: w1117 -> [w1142 _]
          tunnel: w1116 -> [w1141 w1149]
          tunnel: w1113 -> [w1140 w1148]
          tunnel: w1112 -> [w1139 w1147]
          frame True {
            n723 = Bundle By Name(cluster=w1141, "Transient Gains.Line Fit Response.Offset"=w1145, "Transient Gains.Line Fit Response.Slope"=w1142, "Transient Gains.Line Fit Stimulus.Offset"=w1144, "Transient Gains.Line Fit Stimulus.Slope"=w1143, "Transient Gains.Ga"=w1140, "Transient Gains.Ga SD"=w1139, "Fit Calculated"=TRUE) -> (w1146:T18)
          }
          frame False {
            n724 = Bundle By Name(cluster=w1149, "Transient Gains.Ga"=w1148, "Transient Gains.Ga SD"=w1147) -> (w1150:T18)
          }
        }
      }
      frame "Calculate Latency Fits" {
        # "Dependent on Latency Statistic selector (mean trace, individual trace, etc...)"
        n725 = Unbundle By Name(w1451) -> ("Fit Calculated"=w1442:bool, "Transient Gains.Snap Cursor"=w1456:u16, "Transient Gains.Latency window"=w1441:u16, "Transient Gains.Stim.Onset"=w1462:dbl, "Data File.Sample Rate"=w1450:i32, "Transient Gains.Latency Stat."=w1449:u16, "Transient Gains.Latency"=w1446:u16, "Transient Gains.GA1 desaccading"=w1438:bool)
        n726 = Equal?(x=u16 4, y=w1456) -> (x = y?=w1454:bool)
        n727 = case shown="False" w1442 {
          tunnel: [w1471 w1472] -> w1440
          tunnel: w1441 -> [w1471 w1472]
          frame False {
          }
          frame True {
          }
        }
        n728 = Reciprocal(x=w1450) -> (1/x=w1460:dbl)
        n729 = case shown="0, Default" w1440 {
          tunnel: [w1737 w1744 w1749 w1754 w1759 w1764 w1769] -> w1443
          tunnel: [w1738 w1743 w1748 w1753 w1758 w1763 w1768] -> w1444
          tunnel: w1462 -> [_ w1745 w1750 w1755 w1760 w1765 w1770]
          frame 0, Default {
            n730 = stacked-sequence {
              tunnel: [_ w1741] -> w1738
              tunnel: [w1739 _] -> w1737
              frame #0 {
                n731 = property on="Impulse Trace" class="WFGraph (strict)"("Active Cursor"=u32 0) -> ("Cursor.Cursor Position:Cursor X"=w1739:dbl)  [unwired: 2 in, 2 out]
              }
              frame #1 {
                n732 = property on="Impulse Trace" class="WFGraph (strict)"("Active Cursor"=u32 1) -> ("Cursor.Cursor Position:Cursor X"=w1741:dbl)  [unwired: 2 in, 2 out]
              }
            }
          }
          frame 1 {
            n733 = Add(x=w1745, y=10.0) -> (x+y=w1743:dbl)
            n734 = Add(x=w1743, y=10.0) -> (x+y=w1744:dbl)
          }
          frame 2 {
            n735 = Add(x=w1750, y=20.0) -> (x+y=w1748:dbl)
            n736 = Add(x=w1748, y=10.0) -> (x+y=w1749:dbl)
          }
          frame 3 {
            n737 = Add(x=w1755, y=30.0) -> (x+y=w1753:dbl)
            n738 = Add(x=w1753, y=10.0) -> (x+y=w1754:dbl)
          }
          frame 4 {
            n739 = Add(x=w1760, y=40.0) -> (x+y=w1758:dbl)
            n740 = Add(x=w1758, y=10.0) -> (x+y=w1759:dbl)
          }
          frame 5 {
            n741 = Add(x=w1765, y=20.0) -> (x+y=w1763:dbl)
            n742 = Add(x=w1763, y=20.0) -> (x+y=w1764:dbl)
          }
          frame 6 {
            n743 = Add(x=w1770, y=10.0) -> (x+y=w1768:dbl)
            n744 = Add(x=w1768, y=20.0) -> (x+y=w1769:dbl)
          }
        }
        n745 = Divide(x=w1450, y=1000.0) -> (x/y=w1461:dbl)
        n746 = Multiply(x=w1444, y=w1461) -> (x*y=w1457:dbl)
        n747 = Multiply(x=w1443, y=w1461) -> (x*y=w1458:dbl)
        n748 = case shown="True" w1454 {
          tunnel: w1443 -> [_ w1732]
          tunnel: w1444 -> [_ w1731]
          frame False {
          }
          frame True {
            n749 = stacked-sequence {
              tunnel: w1732 -> [w1733 _]
              tunnel: w1731 -> [_ w1735]
              frame #0 {
                n750 = property on="Impulse Trace" class="WFGraph (strict)"("Cursor.Cursor Position:Cursor X"=w1733, "Active Cursor"=u32 0) -> ()  [unwired: 2 in, 2 out]
              }
              frame #1 {
                n751 = property on="Impulse Trace" class="WFGraph (strict)"("Cursor.Cursor Position:Cursor X"=w1735, "Active Cursor"=u32 1) -> ()  [unwired: 2 in, 2 out]
              }
            }
          }
        }
        n752 = Subtract(x=w1458, y=w1457) -> (x-y=w1459:dbl)
        n753 = To Long Integer(number=w1457) -> (32bit integer=w1463:i32)
        n754 = To Long Integer(number=w1459) -> (32bit integer=w1464:i32)
        n755 = case shown="1" w1449 {
          tunnel: [w1503 w1542 w1610 w1681] -> w1467
          tunnel: [w1502 w1540 w1610 w1681] -> w1465
          tunnel: w1464 -> [w1501 w1546 w1616 w1687]
          tunnel: w1463 -> [w1500 w1545 w1615 w1686]
          tunnel: w1460 -> [w1499 w1547 w1617 w1688]
          tunnel: [w1494 w1539 w1610 w1681] -> w1453
          tunnel: [w1493 w1541 w1610 w1681] -> w1452
          tunnel: w1451 -> [w1495 w1556 w1626 w1697]
          tunnel: [w1492 w1544 w1614 w1685] -> w1448
          tunnel: [w1490 w1543 w1613 w1684] -> w1447
          tunnel: w1446 -> [_ _ w1609 w1680]
          tunnel: [TRUE TRUE FALSE FALSE] -> w1445
          tunnel: w1438 -> [_ w1531 w1604 w1675]
          frame 0, Default {
            w1491 = 0.0 ("standard deviation")
            n756 = Unbundle By Name(w1495) -> ("Stimulus"=w1487:dbl[], "Response"=w1488:dbl[])
            n757 = for {
              tunnel: w1499 -> [w1528]
              tunnel: [w1526] -> w1486 mode=indexing
              tunnel: w1488 -> [_] mode=indexing
              i -> [w1525]
              n758 = Multiply(x=w1528, y=w1525) -> (x*y=w1524:dbl)
              n759 = Build Array(1.0 ("Input Element"), w1524) -> (w1526:dbl[])
            }
            n760 = Array Subset(array=w1488, index=w1500, length=w1501) -> (w1497:dbl[])
            n761 = Array Subset(array=w1487, index=w1500, length=w1501) -> (w1498:dbl[])
            n762 = Array Subset(array=w1486, index (row)=w1500, length (row)=w1501) -> (w1496:dbl[][])  [unwired: 2 in]
            n763 = disable-structure shown="Enabled" {
              disable-tunnel: [w1516 w1521] -> w1503
              disable-tunnel: [w1515 w1519] -> w1502
              disable-tunnel: w1498 -> [w1510 w1523]
              disable-tunnel: w1497 -> [w1509 w1522]
              disable-tunnel: w1496 -> [w1508 w1517]
              disable-tunnel: [w1505 w1518] -> w1494
              disable-tunnel: [w1504 w1520] -> w1493
              frame Disabled {
                n764 = call <vilib>:"General LS Linear Fit (obs).vi"("H"=w1508, "Y"=w1510) -> ("Coefficients"=w1507:dbl[])  [unwired: 3 in, 4 out]
                n765 = call <vilib>:"General LS Linear Fit (obs).vi"("H"=w1508, "Y"=w1509) -> ("Coefficients"=w1506:dbl[])  [unwired: 3 in, 4 out]
                n766 = Index Array(array=w1507, index=0 ("Index")) -> (element=w1515:dbl)
                n767 = Index Array(array=w1507, index=1 ("Index")) -> (element=w1505:dbl)
                n768 = Index Array(array=w1506, index=0 ("Index")) -> (element=w1516:dbl)
                n769 = Index Array(array=w1506, index=1 ("Index")) -> (element=w1504:dbl)
              }
              frame Enabled {
                n770 = call "linear fit NaN.vi"("Array 2"=w1517, "Array"=w1523) -> ("sloap"=w1518:dbl, "intercept"=w1519:dbl)  [unwired: 2 in]
                n771 = call "linear fit NaN.vi"("Array 2"=w1517, "Array"=w1522) -> ("sloap"=w1520:dbl, "intercept"=w1521:dbl)  [unwired: 2 in]
              }
            }
            n772 = Divide(x=w1493, y=w1494) -> (x/y=w1492:dbl)
            n773 = Divide(x=w1491, y=w1491) -> (x/y=w1490:dbl)
          }
          frame 1 {
            n774 = Unbundle By Name(w1556) -> ("Data File"=w1561:T25, "Impulse Positions"=w1560:T24, "desaccading parameters.Impulse dir"=w1559:bool, "desaccading parameters.Impulse Plane 2"=w1558:T28, "desacc"=w1557:T27)
            n775 = local read "Parameter Impuls Series"() -> (w1554:T3)
            n776 = Array Size(array=w1554) -> (size(s)=w1549:i32)
            n777 = local read "Trace Select"() -> (w1535:i32)
            n778 = local read "Interpolate 3"() -> (w1536:bool)
            n779 = call "Couple Head Impulse Traces.vi"("Data Input"=w1561, "Impulse Positions"=w1560, "Trace Select"=w1535, "Impulse Direction +ve?"=w1559, "Impulse Plane"=w1558, "Mean and STD"=FALSE ("Mean Traces"), "Plot Selection 2"=w1554, "desacc"=w1557, "Interpolate"=w1536, "desacc."=TRUE, "man. desacc.."=w1531) -> ("Impulses"=w1553:dbl[][])  [unwired: 5 in, 3 out]
            n780 = Array Size(array=w1553) -> (size(s)=w1552:i32[])
            n781 = Index Array(array=w1552, index=0) -> (element=w1550:i32)
            n782 = Quotient & Remainder(x=w1550, y=w1549) -> (floor(x/y)=w1548:i32)  [unwired: 1 out]
            n783 = for {
              N: w1548 -> [w1576]
              tunnel: w1553 -> [w1567]
              tunnel: w1547 -> [w1575]
              tunnel: w1546 -> [w1574]
              tunnel: w1545 -> [w1573]
              tunnel: [w1572] -> w1533 mode=indexing
              tunnel: [w1571] -> w1529 mode=indexing
              tunnel: [w1570] -> w1534 mode=indexing
              tunnel: [w1569] -> w1530 mode=indexing
              i -> [w1577]
              n784 = Add(x=w1576, y=w1577) -> (x+y=w1578:i32)
              n785 = Index Array(array=w1567, index (row)=w1577) -> (element=w1564:dbl[])  [unwired: 1 in]
              n786 = Index Array(array=w1567, index (row)=w1578) -> (element=w1565:dbl[])  [unwired: 1 in]
              n787 = for {
                tunnel: w1575 -> [w1603]
                tunnel: [w1601] -> w1563 mode=indexing
                tunnel: w1565 -> [_] mode=indexing
                i -> [w1600]
                n788 = Multiply(x=w1603, y=w1600) -> (x*y=w1599:dbl)
                n789 = Build Array(1.0 ("Input Element"), w1599) -> (w1601:dbl[])
              }
              n790 = Array Subset(array=w1565, index=w1573, length=w1574) -> (w1566:dbl[])
              n791 = Array Subset(array=w1564, index=w1573, length=w1574) -> (w1568:dbl[])
              n792 = Array Subset(array=w1563, index (row)=w1573, length (row)=w1574) -> (w1562:dbl[][])  [unwired: 2 in]
              n793 = disable-structure shown="Enabled" {
                disable-tunnel: [w1585 w1593] -> w1572
                disable-tunnel: [w1584 w1594] -> w1571
                disable-tunnel: [w1583 w1595] -> w1570
                disable-tunnel: [w1582 w1596] -> w1569
                disable-tunnel: w1562 -> [w1581 _]
                disable-tunnel: w1568 -> [w1580 w1598]
                disable-tunnel: w1566 -> [w1579 w1597]
                disable-tunnel: w1562 -> [_ w1592]
                frame Disabled {
                  n794 = call <vilib>:"General LS Linear Fit (obs).vi"("H"=w1581, "Y"=w1580) -> ("Coefficients"=w1587:dbl[])  [unwired: 3 in, 4 out]
                  n795 = call <vilib>:"General LS Linear Fit (obs).vi"("H"=w1581, "Y"=w1579) -> ("Coefficients"=w1586:dbl[])  [unwired: 3 in, 4 out]
                  n796 = Index Array(array=w1587, index=0 ("Index")) -> (element=w1584:dbl)
                  n797 = Index Array(array=w1587, index=1 ("Index")) -> (element=w1585:dbl)
                  n798 = Index Array(array=w1586, index=0 ("Index")) -> (element=w1582:dbl)
                  n799 = Index Array(array=w1586, index=1 ("Index")) -> (element=w1583:dbl)
                }
                frame Enabled {
                  n800 = call "linear fit NaN.vi"("Array 2"=w1592, "Array"=w1597) -> ("sloap"=w1595:dbl, "intercept"=w1596:dbl)  [unwired: 2 in]
                  n801 = call "linear fit NaN.vi"("Array 2"=w1592, "Array"=w1598) -> ("sloap"=w1593:dbl, "intercept"=w1594:dbl)  [unwired: 2 in]
                }
              }
            }
            n802 = Divide(x=w1534, y=w1533) -> (x/y=w1538:dbl[])
            n803 = call "standard deviation NaN.vi"("Array"=w1538) -> ("standard deviation"=w1543:dbl, "mean"=w1544:dbl)  [unwired: 2 in, 1 out]
            n804 = call "mean_nan.vi"("Array"=w1530) -> ("Mean"=w1542:dbl)  [unwired: 10 in]
            n805 = call "mean_nan.vi"("Array"=w1534) -> ("Mean"=w1541:dbl)  [unwired: 10 in]
            n806 = call "mean_nan.vi"("Array"=w1529) -> ("Mean"=w1540:dbl)  [unwired: 10 in]
            n807 = call "mean_nan.vi"("Array"=w1533) -> ("Mean"=w1539:dbl)  [unwired: 10 in]
          }
          frame 2 {
            w1611 = 0.0 ("standard deviation")
            n808 = Unbundle By Name(w1626) -> ("Data File"=w1631:T25, "Impulse Positions"=w1630:T24, "desaccading parameters.Impulse dir"=w1629:bool, "desaccading parameters.Impulse Plane 2"=w1628:T28, "desacc"=w1627:T27)
            n809 = local read "Parameter Impuls Series"() -> (w1624:T3)
            n810 = local read "Interpolate 3"() -> (w1607:bool)
            n811 = Array Size(array=w1624) -> (size(s)=w1619:i32)
            n812 = local read "Trace Select"() -> (w1606:i32)
            n813 = call "Couple Head Impulse Traces.vi"("Data Input"=w1631, "Impulse Positions"=w1630, "Trace Select"=w1606, "Impulse Direction +ve?"=w1629, "Impulse Plane"=w1628, "Mean and STD"=FALSE ("Mean Traces"), "Plot Selection 2"=w1624, "desacc"=w1627, "Interpolate"=w1607, "desacc."=FALSE, "man. desacc.."=w1604) -> ("Impulses"=w1623:dbl[][])  [unwired: 5 in, 3 out]
            n814 = Array Size(array=w1623) -> (size(s)=w1622:i32[])
            n815 = Index Array(array=w1622, index=0) -> (element=w1620:i32)
            n816 = Quotient & Remainder(x=w1620, y=w1619) -> (floor(x/y)=w1618:i32)  [unwired: 1 out]
            n817 = for {
              N: w1618 -> [w1650]
              tunnel: w1623 -> [w1653]
              tunnel: w1617 -> [w1646]
              tunnel: w1616 -> [w1648]
              tunnel: w1615 -> [w1649]
              tunnel: [w1647] -> w1612 mode=indexing
              tunnel: w1609 -> [w1642]
              i -> [w1651]
              n818 = Add(x=w1650, y=w1651) -> (x+y=w1652:i32)
              n819 = Index Array(array=w1653, index (row)=w1651) -> (element=w1632:dbl[])  [unwired: 1 in]
              n820 = Index Array(array=w1653, index (row)=w1652) -> (element=w1633:dbl[])  [unwired: 1 in]
              n821 = for {
                tunnel: w1646 -> [w1674]
                tunnel: [w1672] -> _ mode=indexing
                tunnel: w1633 -> [_] mode=indexing
                i -> [w1671]
                n822 = Multiply(x=w1674, y=w1671) -> (x*y=w1670:dbl)
                n823 = Build Array(1.0 ("Input Element"), w1670) -> (w1672:dbl[])
              }
              n824 = Reciprocal(x=w1646) -> (1/x=w1645:dbl)
              n825 = Divide(x=w1645, y=1000.0) -> (x/y=w1643:dbl)
              n826 = Multiply(x=w1642, y=w1643) -> (x*y=w1641:dbl)
              n827 = Round To Nearest(number=w1641) -> (nearest integer value=w1637:dbl)
              n828 = Array Subset(array=w1633, index=w1649, length=w1648) -> (w1639:dbl[])
              n829 = Array Subset(array=w1632, index=w1649, length=w1648) -> (w1638:dbl[])
              n830 = Greater Or Equal To 0?(x=w1637) -> (x >= 0?=w1640:bool)
              n831 = case shown="True" w1640 {
                tunnel: w1638 -> [w1655 w1664]
                tunnel: w1639 -> [w1661 w1665]
                tunnel: w1637 -> [w1658 w1667]
                tunnel: [w1656 w1663] -> w1635
                tunnel: [w1654 w1662] -> w1634
                frame True {
                  n832 = Array Size(array=w1661) -> (size(s)=w1659:i32)
                  n833 = Subtract(x=w1659, y=w1658) -> (x-y=w1657:dbl)
                  n834 = Array Subset(array=w1661, index=w1658, length=w1659) -> (w1656:dbl[])
                  n835 = Array Subset(array=w1655, index=0, length=w1657) -> (w1654:dbl[])
                }
                frame False {
                  n836 = Array Size(array=w1665) -> (size(s)=w1668:i32)
                  n837 = Subtract(x=w1668, y=w1667) -> (x-y=w1666:dbl)
                  n838 = Array Subset(array=w1664, index=w1667, length=w1668) -> (w1662:dbl[])
                  n839 = Array Subset(array=w1665, index=0, length=w1666) -> (w1663:dbl[])
                }
              }
              n840 = Divide(x=w1635, y=w1634) -> (x/y=w1636:dbl[])
              n841 = call "mean_nan.vi"("Array"=w1636) -> ("Mean"=w1647:dbl)  [unwired: 10 in]
            }
            n842 = call "standard deviation NaN.vi"("Array"=w1612) -> ("standard deviation"=w1613:dbl, "mean"=w1614:dbl)  [unwired: 2 in, 1 out]
            n843 = Divide(x=w1611, y=w1611) -> (x/y=w1610:dbl)
          }
          frame 3 {
            w1682 = 0.0 ("standard deviation")
            n844 = Unbundle By Name(w1697) -> ("Data File"=w1702:T25, "Impulse Positions"=w1701:T24, "desaccading parameters.Impulse dir"=w1700:bool, "desaccading parameters.Impulse Plane 2"=w1699:T28, "desacc"=w1698:T27)
            n845 = local read "Trace Select"() -> (w1677:i32)
            n846 = local read "Parameter Impuls Series"() -> (w1695:T3)
            n847 = call "Couple Head Impulse Traces.vi"("Data Input"=w1702, "Impulse Positions"=w1701, "Trace Select"=w1677, "Impulse Direction +ve?"=w1700, "Impulse Plane"=w1699, "Mean and STD"=FALSE ("Mean Traces"), "Plot Selection 2"=w1695, "desacc"=w1698, "Interpolate"="Interpolate 3", "desacc."=FALSE, "man. desacc.."=w1675) -> ("Impulses"=w1694:dbl[][])  [unwired: 5 in, 3 out]
            n848 = Array Size(array=w1695) -> (size(s)=w1690:i32)
            n849 = Array Size(array=w1694) -> (size(s)=w1693:i32[])
            n850 = Index Array(array=w1693, index=0) -> (element=w1691:i32)
            n851 = Quotient & Remainder(x=w1691, y=w1690) -> (floor(x/y)=w1689:i32)  [unwired: 1 out]
            n852 = for {
              N: w1689 -> [w1722]
              tunnel: w1694 -> [w1725]
              tunnel: w1688 -> [w1713]
              tunnel: w1687 -> [w1715]
              tunnel: w1686 -> [w1716]
              tunnel: [w1714] -> w1683 mode=indexing
              tunnel: w1680 -> [_]
              i -> [w1723]
              (unwired) 1000.0 ("y")
              n853 = Add(x=w1722, y=w1723) -> (x+y=w1724:i32)
              n854 = Index Array(array=w1725, index (row)=w1723) -> (element=w1717:dbl[])  [unwired: 1 in]
              n855 = Index Array(array=w1725, index (row)=w1724) -> (element=w1718:dbl[])  [unwired: 1 in]
              n856 = for {
                tunnel: w1713 -> [w1730]
                tunnel: [w1728] -> w1721 mode=indexing
                tunnel: w1718 -> [_] mode=indexing
                i -> [w1727]
                n857 = Multiply(x=w1730, y=w1727) -> (x*y=w1726:dbl)
                n858 = Build Array(1.0 ("Input Element"), w1726) -> (w1728:dbl[])
              }
              n859 = call <userlib>:"Remove NaNs.vi"("Sinusoid"=w1721, "Response"=w1718, "Stimulus"=w1717) -> ("Response (out)"=w1719:dbl[], "Stimulus (out)"=w1720:dbl[])  [unwired: 1 out]
              n860 = Reciprocal(x=w1713) -> (1/x=w1706:dbl)
              n861 = Array Subset(array=w1719, index=w1716, length=w1715) -> (w1708:dbl[])
              n862 = Array Subset(array=w1720, index=w1716, length=w1715) -> (w1707:dbl[])
              n863 = Build Array(w1708, w1707) -> (w1711:dbl[][])
              n864 = call "Differentiate 3D.vi"("Sample Rate 4"=w1706, "Data (in)"=w1711) -> ("Data (differentiated)"=w1703:dbl[][])  [unwired: 3 in]
              n865 = Index Array(array=w1703, index (row)=0) -> (element=w1704:dbl[])  [unwired: 1 in]
              n866 = Index Array(array=w1703, index (row)=1) -> (element=w1705:dbl[])  [unwired: 1 in]
              n867 = Divide(x=w1704, y=w1705) -> (x/y=w1712:dbl[])
              n868 = call-poly <vilib>:"Mean.vi"("X"=w1712) -> ("mean"=w1714:dbl)  [unwired: 1 out]
            }
            n869 = call <vilib>:"Std Deviation and Variance.vi"("X"=w1683) -> ("mean"=w1685:dbl, "standard deviation"=w1684:dbl)  [unwired: 1 in, 1 out]
            n870 = Divide(x=w1682, y=w1682) -> (x/y=w1681:dbl)
          }
        }
        n871 = case shown="True" w1445 {
          tunnel: [w1481 w1485] -> w1468
          tunnel: w1467 -> [w1480 _]
          tunnel: w1465 -> [w1479 _]
          tunnel: w1453 -> [w1478 _]
          tunnel: w1452 -> [w1477 _]
          tunnel: w1451 -> [w1476 w1484]
          tunnel: w1448 -> [w1475 w1483]
          tunnel: w1447 -> [w1474 w1482]
          frame True {
            n872 = Bundle By Name(cluster=w1476, "Transient Gains.Line Fit Res Latency.Offset"=w1480, "Transient Gains.Line Fit Res Latency.Slope"=w1477, "Transient Gains.Line Fit Stim Latency.Offset"=w1479, "Transient Gains.Line Fit Stim Latency.Slope"=w1478, "Transient Gains.Ga"=w1475, "Transient Gains.Ga SD"=w1474, "Fit Calculated"=TRUE) -> (w1481:T18)
          }
          frame False {
            n873 = Bundle By Name(cluster=w1484, "Transient Gains.Ga"=w1483, "Transient Gains.Ga SD"=w1482) -> (w1485:T18)
          }
        }
      }
      frame "Calculate Transient Ga 2 Gain" {
        n874 = Unbundle By Name(w1786) -> ("Fit Calculated"=w1777:bool, "Transient Gains.Snap Cursor"=w1791:u16, "Transient Gains.Ga Window  (late)"=w1776:u16, "Transient Gains.Stim.Onset"=w1797:dbl, "Data File.Sample Rate"=w1785:i32, "Transient Gains.Ga Stat. 2"=w1784:u16, "Transient Gains.Latency"=w1781:u16, "Transient Gains.GA2 desaccading"=w1773:bool)
        n875 = Equal?(x=u16 2, y=w1791) -> (x = y?=w1789:bool)
        n876 = case shown="False" w1777 {
          tunnel: [u16 6 ("Ga Window") w1807] -> w1775
          tunnel: w1776 -> [_ w1807]
          frame False {
          }
          frame True {
          }
        }
        n877 = Reciprocal(x=w1785) -> (1/x=w1795:dbl)
        n878 = case shown="6" w1775 {
          tunnel: [w2072 w2079 w2084 w2089 w2094 w2099 w2104] -> w1778
          tunnel: [w2073 w2078 w2083 w2088 w2093 w2098 w2103] -> w1779
          tunnel: w1797 -> [_ w2080 w2085 w2090 w2095 w2100 w2105]
          frame 0, Default {
            n879 = stacked-sequence {
              tunnel: [_ w2076] -> w2073
              tunnel: [w2074 _] -> w2072
              frame #0 {
                n880 = property on="Impulse Trace" class="WFGraph (strict)"("Active Cursor"=u32 0) -> ("Cursor.Cursor Position:Cursor X"=w2074:dbl)  [unwired: 2 in, 2 out]
              }
              frame #1 {
                n881 = property on="Impulse Trace" class="WFGraph (strict)"("Active Cursor"=u32 1) -> ("Cursor.Cursor Position:Cursor X"=w2076:dbl)  [unwired: 2 in, 2 out]
              }
            }
          }
          frame 1 {
            n882 = Add(x=w2080, y=10.0) -> (x+y=w2078:dbl)
            n883 = Add(x=w2078, y=10.0) -> (x+y=w2079:dbl)
          }
          frame 2 {
            n884 = Add(x=w2085, y=20.0) -> (x+y=w2083:dbl)
            n885 = Add(x=w2083, y=10.0) -> (x+y=w2084:dbl)
          }
          frame 3 {
            n886 = Add(x=w2090, y=30.0) -> (x+y=w2088:dbl)
            n887 = Add(x=w2088, y=10.0) -> (x+y=w2089:dbl)
          }
          frame 4 {
            n888 = Add(x=w2095, y=40.0) -> (x+y=w2093:dbl)
            n889 = Add(x=w2093, y=10.0) -> (x+y=w2094:dbl)
          }
          frame 5 {
            n890 = Add(x=w2100, y=20.0) -> (x+y=w2098:dbl)
            n891 = Add(x=w2098, y=20.0) -> (x+y=w2099:dbl)
          }
          frame 6 {
            n892 = Add(x=w2105, y=10.0) -> (x+y=w2103:dbl)
            n893 = Add(x=w2103, y=20.0) -> (x+y=w2104:dbl)
          }
        }
        n894 = Divide(x=w1785, y=1000.0) -> (x/y=w1796:dbl)
        n895 = Multiply(x=w1779, y=w1796) -> (x*y=w1792:dbl)
        n896 = Multiply(x=w1778, y=w1796) -> (x*y=w1793:dbl)
        n897 = case shown="True" w1789 {
          tunnel: w1778 -> [_ w2067]
          tunnel: w1779 -> [_ w2066]
          frame False {
          }
          frame True {
            n898 = stacked-sequence {
              tunnel: w2067 -> [w2068 _]
              tunnel: w2066 -> [_ w2070]
              frame #0 {
                n899 = property on="Impulse Trace" class="WFGraph (strict)"("Cursor.Cursor Position:Cursor X"=w2068, "Active Cursor"=u32 0) -> ()  [unwired: 2 in, 2 out]
              }
              frame #1 {
                n900 = property on="Impulse Trace" class="WFGraph (strict)"("Cursor.Cursor Position:Cursor X"=w2070, "Active Cursor"=u32 1) -> ()  [unwired: 2 in, 2 out]
              }
            }
          }
        }
        n901 = Subtract(x=w1793, y=w1792) -> (x-y=w1794:dbl)
        n902 = To Long Integer(number=w1792) -> (32bit integer=w1798:i32)
        n903 = To Long Integer(number=w1794) -> (32bit integer=w1799:i32)
        n904 = case shown="0, Default" w1784 {
          tunnel: [w1838 w1877 w1945 w2016] -> w1802
          tunnel: [w1837 w1875 w1945 w2016] -> w1800
          tunnel: w1799 -> [w1836 w1881 w1951 w2022]
          tunnel: w1798 -> [w1835 w1880 w1950 w2021]
          tunnel: w1795 -> [w1834 w1882 w1952 w2023]
          tunnel: [w1829 w1874 w1945 w2016] -> w1788
          tunnel: [w1828 w1876 w1945 w2016] -> w1787
          tunnel: w1786 -> [w1830 w1891 w1961 w2032]
          tunnel: [w1827 w1879 w1949 w2020] -> w1783
          tunnel: [w1825 w1878 w1948 w2019] -> w1782
          tunnel: w1781 -> [_ _ w1944 w2015]
          tunnel: [TRUE TRUE FALSE FALSE] -> w1780
          tunnel: w1773 -> [_ w1864 w1939 w2010]
          frame 0, Default {
            w1826 = 0.0 ("standard deviation")
            n905 = Unbundle By Name(w1830) -> ("Stimulus"=w1822:dbl[], "Response"=w1823:dbl[])
            n906 = for {
              tunnel: w1834 -> [w1863]
              tunnel: [w1861] -> w1821 mode=indexing
              tunnel: w1823 -> [_] mode=indexing
              i -> [w1860]
              n907 = Multiply(x=w1863, y=w1860) -> (x*y=w1859:dbl)
              n908 = Build Array(1.0 ("Input Element"), w1859) -> (w1861:dbl[])
            }
            n909 = Array Subset(array=w1823, index=w1835, length=w1836) -> (w1832:dbl[])
            n910 = Array Subset(array=w1822, index=w1835, length=w1836) -> (w1833:dbl[])
            n911 = Array Subset(array=w1821, index (row)=w1835, length (row)=w1836) -> (w1831:dbl[][])  [unwired: 2 in]
            n912 = disable-structure shown="Enabled" {
              disable-tunnel: [w1851 w1856] -> w1838
              disable-tunnel: [w1850 w1854] -> w1837
              disable-tunnel: w1833 -> [w1845 w1858]
              disable-tunnel: w1832 -> [w1844 w1857]
              disable-tunnel: w1831 -> [w1843 w1852]
              disable-tunnel: [w1840 w1853] -> w1829
              disable-tunnel: [w1839 w1855] -> w1828
              frame Disabled {
                n913 = call <vilib>:"General LS Linear Fit (obs).vi"("H"=w1843, "Y"=w1845) -> ("Coefficients"=w1842:dbl[])  [unwired: 3 in, 4 out]
                n914 = call <vilib>:"General LS Linear Fit (obs).vi"("H"=w1843, "Y"=w1844) -> ("Coefficients"=w1841:dbl[])  [unwired: 3 in, 4 out]
                n915 = Index Array(array=w1842, index=0 ("Index")) -> (element=w1850:dbl)
                n916 = Index Array(array=w1842, index=1 ("Index")) -> (element=w1840:dbl)
                n917 = Index Array(array=w1841, index=0 ("Index")) -> (element=w1851:dbl)
                n918 = Index Array(array=w1841, index=1 ("Index")) -> (element=w1839:dbl)
              }
              frame Enabled {
                n919 = call "linear fit NaN.vi"("Array 2"=w1852, "Array"=w1858) -> ("sloap"=w1853:dbl, "intercept"=w1854:dbl)  [unwired: 2 in]
                n920 = call "linear fit NaN.vi"("Array 2"=w1852, "Array"=w1857) -> ("sloap"=w1855:dbl, "intercept"=w1856:dbl)  [unwired: 2 in]
              }
            }
            n921 = Divide(x=w1828, y=w1829) -> (x/y=w1827:dbl)
            n922 = Divide(x=w1826, y=w1826) -> (x/y=w1825:dbl)
          }
          frame 1 {
            n923 = Unbundle By Name(w1891) -> ("Data File"=w1896:T25, "Impulse Positions"=w1895:T24, "desaccading parameters.Impulse dir"=w1894:bool, "desaccading parameters.Impulse Plane 2"=w1893:T28, "desacc"=w1892:T27)
            n924 = local read "Parameter Impuls Series"() -> (w1889:T3)
            n925 = local read "Interpolate 2"() -> (w1871:bool)
            n926 = Array Size(array=w1889) -> (size(s)=w1884:i32)
            n927 = local read "Trace Select"() -> (w1870:i32)
            n928 = call "Couple Head Impulse Traces.vi"("Data Input"=w1896, "Impulse Positions"=w1895, "Trace Select"=w1870, "Impulse Direction +ve?"=w1894, "Impulse Plane"=w1893, "Mean and STD"=FALSE ("Mean Traces"), "Plot Selection 2"=w1889, "desacc"=w1892, "Interpolate"=w1871, "desacc."=FALSE, "man. desacc.."=w1864) -> ("Impulses"=w1888:dbl[][])  [unwired: 5 in, 3 out]
            n929 = Array Size(array=w1888) -> (size(s)=w1887:i32[])
            n930 = Index Array(array=w1887, index=0) -> (element=w1885:i32)
            n931 = Quotient & Remainder(x=w1885, y=w1884) -> (floor(x/y)=w1883:i32)  [unwired: 1 out]
            n932 = for {
              N: w1883 -> [w1911]
              tunnel: w1888 -> [w1902]
              tunnel: w1882 -> [w1910]
              tunnel: w1881 -> [w1909]
              tunnel: w1880 -> [w1908]
              tunnel: [w1907] -> w1866 mode=indexing
              tunnel: [w1906] -> w1868 mode=indexing
              tunnel: [w1905] -> w1867 mode=indexing
              tunnel: [w1904] -> w1869 mode=indexing
              i -> [w1912]
              n933 = Add(x=w1911, y=w1912) -> (x+y=w1913:i32)
              n934 = Index Array(array=w1902, index (row)=w1912) -> (element=w1899:dbl[])  [unwired: 1 in]
              n935 = Index Array(array=w1902, index (row)=w1913) -> (element=w1900:dbl[])  [unwired: 1 in]
              n936 = for {
                tunnel: w1910 -> [w1938]
                tunnel: [w1936] -> w1898 mode=indexing
                tunnel: w1900 -> [_] mode=indexing
                i -> [w1935]
                n937 = Multiply(x=w1938, y=w1935) -> (x*y=w1934:dbl)
                n938 = Build Array(1.0 ("Input Element"), w1934) -> (w1936:dbl[])
              }
              n939 = Array Subset(array=w1900, index=w1908, length=w1909) -> (w1901:dbl[])
              n940 = Array Subset(array=w1899, index=w1908, length=w1909) -> (w1903:dbl[])
              n941 = Array Subset(array=w1898, index (row)=w1908, length (row)=w1909) -> (w1897:dbl[][])  [unwired: 2 in]
              n942 = disable-structure shown="Enabled" {
                disable-tunnel: [w1920 w1928] -> w1907
                disable-tunnel: [w1919 w1929] -> w1906
                disable-tunnel: [w1918 w1930] -> w1905
                disable-tunnel: [w1917 w1931] -> w1904
                disable-tunnel: w1897 -> [w1916 _]
                disable-tunnel: w1903 -> [w1915 w1933]
                disable-tunnel: w1901 -> [w1914 w1932]
                disable-tunnel: w1897 -> [_ w1927]
                frame Disabled {
                  n943 = call <vilib>:"General LS Linear Fit (obs).vi"("H"=w1916, "Y"=w1915) -> ("Coefficients"=w1922:dbl[])  [unwired: 3 in, 4 out]
                  n944 = call <vilib>:"General LS Linear Fit (obs).vi"("H"=w1916, "Y"=w1914) -> ("Coefficients"=w1921:dbl[])  [unwired: 3 in, 4 out]
                  n945 = Index Array(array=w1922, index=0 ("Index")) -> (element=w1919:dbl)
                  n946 = Index Array(array=w1922, index=1 ("Index")) -> (element=w1920:dbl)
                  n947 = Index Array(array=w1921, index=0 ("Index")) -> (element=w1917:dbl)
                  n948 = Index Array(array=w1921, index=1 ("Index")) -> (element=w1918:dbl)
                }
                frame Enabled {
                  n949 = call "linear fit NaN.vi"("Array 2"=w1927, "Array"=w1932) -> ("sloap"=w1930:dbl, "intercept"=w1931:dbl)  [unwired: 2 in]
                  n950 = call "linear fit NaN.vi"("Array 2"=w1927, "Array"=w1933) -> ("sloap"=w1928:dbl, "intercept"=w1929:dbl)  [unwired: 2 in]
                }
              }
            }
            n951 = Divide(x=w1867, y=w1866) -> (x/y=w1873:dbl[])
            n952 = call "standard deviation NaN.vi"("Array"=w1873) -> ("standard deviation"=w1878:dbl, "mean"=w1879:dbl)  [unwired: 2 in, 1 out]
            n953 = call "mean_nan.vi"("Array"=w1869) -> ("Mean"=w1877:dbl)  [unwired: 10 in]
            n954 = call "mean_nan.vi"("Array"=w1867) -> ("Mean"=w1876:dbl)  [unwired: 10 in]
            n955 = call "mean_nan.vi"("Array"=w1868) -> ("Mean"=w1875:dbl)  [unwired: 10 in]
            n956 = call "mean_nan.vi"("Array"=w1866) -> ("Mean"=w1874:dbl)  [unwired: 10 in]
          }
          frame 2 {
            w1946 = 0.0 ("standard deviation")
            n957 = Unbundle By Name(w1961) -> ("Data File"=w1966:T25, "Impulse Positions"=w1965:T24, "desaccading parameters.Impulse dir"=w1964:bool, "desaccading parameters.Impulse Plane 2"=w1963:T28, "desacc"=w1962:T27)
            n958 = local read "Parameter Impuls Series"() -> (w1959:T3)
            n959 = local read "Interpolate 2"() -> (w1942:bool)
            n960 = Array Size(array=w1959) -> (size(s)=w1954:i32)
            n961 = local read "Trace Select"() -> (w1941:i32)
            n962 = call "Couple Head Impulse Traces.vi"("Data Input"=w1966, "Impulse Positions"=w1965, "Trace Select"=w1941, "Impulse Direction +ve?"=w1964, "Impulse Plane"=w1963, "Mean and STD"=FALSE ("Mean Traces"), "Plot Selection 2"=w1959, "desacc"=w1962, "Interpolate"=w1942, "desacc."=FALSE, "man. desacc.."=w1939) -> ("Impulses"=w1958:dbl[][])  [unwired: 5 in, 3 out]
            n963 = Array Size(array=w1958) -> (size(s)=w1957:i32[])
            n964 = Index Array(array=w1957, index=0) -> (element=w1955:i32)
            n965 = Quotient & Remainder(x=w1955, y=w1954) -> (floor(x/y)=w1953:i32)  [unwired: 1 out]
            n966 = for {
              N: w1953 -> [w1985]
              tunnel: w1958 -> [w1988]
              tunnel: w1952 -> [w1981]
              tunnel: w1951 -> [w1983]
              tunnel: w1950 -> [w1984]
              tunnel: [w1982] -> w1947 mode=indexing
              tunnel: w1944 -> [w1977]
              i -> [w1986]
              n967 = Add(x=w1985, y=w1986) -> (x+y=w1987:i32)
              n968 = Index Array(array=w1988, index (row)=w1986) -> (element=w1967:dbl[])  [unwired: 1 in]
              n969 = Index Array(array=w1988, index (row)=w1987) -> (element=w1968:dbl[])  [unwired: 1 in]
              n970 = for {
                tunnel: w1981 -> [w2009]
                tunnel: [w2007] -> _ mode=indexing
                tunnel: w1968 -> [_] mode=indexing
                i -> [w2006]
                n971 = Multiply(x=w2009, y=w2006) -> (x*y=w2005:dbl)
                n972 = Build Array(1.0 ("Input Element"), w2005) -> (w2007:dbl[])
              }
              n973 = Reciprocal(x=w1981) -> (1/x=w1980:dbl)
              n974 = Divide(x=w1980, y=1000.0) -> (x/y=w1978:dbl)
              n975 = Multiply(x=w1977, y=w1978) -> (x*y=w1976:dbl)
              n976 = Round To Nearest(number=w1976) -> (nearest integer value=w1972:dbl)
              n977 = Array Subset(array=w1968, index=w1984, length=w1983) -> (w1974:dbl[])
              n978 = Array Subset(array=w1967, index=w1984, length=w1983) -> (w1973:dbl[])
              n979 = Greater Or Equal To 0?(x=w1972) -> (x >= 0?=w1975:bool)
              n980 = case shown="True" w1975 {
                tunnel: w1973 -> [w1990 w1999]
                tunnel: w1974 -> [w1996 w2000]
                tunnel: w1972 -> [w1993 w2002]
                tunnel: [w1991 w1998] -> w1970
                tunnel: [w1989 w1997] -> w1969
                frame True {
                  n981 = Array Size(array=w1996) -> (size(s)=w1994:i32)
                  n982 = Subtract(x=w1994, y=w1993) -> (x-y=w1992:dbl)
                  n983 = Array Subset(array=w1996, index=w1993, length=w1994) -> (w1991:dbl[])
                  n984 = Array Subset(array=w1990, index=0, length=w1992) -> (w1989:dbl[])
                }
                frame False {
                  n985 = Array Size(array=w2000) -> (size(s)=w2003:i32)
                  n986 = Subtract(x=w2003, y=w2002) -> (x-y=w2001:dbl)
                  n987 = Array Subset(array=w1999, index=w2002, length=w2003) -> (w1997:dbl[])
                  n988 = Array Subset(array=w2000, index=0, length=w2001) -> (w1998:dbl[])
                }
              }
              n989 = Divide(x=w1970, y=w1969) -> (x/y=w1971:dbl[])
              n990 = call "mean_nan.vi"("Array"=w1971) -> ("Mean"=w1982:dbl)  [unwired: 10 in]
            }
            n991 = call "standard deviation NaN.vi"("Array"=w1947) -> ("standard deviation"=w1948:dbl, "mean"=w1949:dbl)  [unwired: 2 in, 1 out]
            n992 = Divide(x=w1946, y=w1946) -> (x/y=w1945:dbl)
          }
          frame 3 {
            w2017 = 0.0 ("standard deviation")
            n993 = Unbundle By Name(w2032) -> ("Data File"=w2037:T25, "Impulse Positions"=w2036:T24, "desaccading parameters.Impulse dir"=w2035:bool, "desaccading parameters.Impulse Plane 2"=w2034:T28, "desacc"=w2033:T27)
            n994 = local read "Parameter Impuls Series"() -> (w2030:T3)
            n995 = Array Size(array=w2030) -> (size(s)=w2025:i32)
            n996 = local read "Trace Select"() -> (w2012:i32)
            n997 = call "Couple Head Impulse Traces.vi"("Data Input"=w2037, "Impulse Positions"=w2036, "Trace Select"=w2012, "Impulse Direction +ve?"=w2035, "Impulse Plane"=w2034, "Mean and STD"=FALSE ("Mean Traces"), "Plot Selection 2"=w2030, "desacc"=w2033, "Interpolate"="Interpolate 2", "desacc."=FALSE, "man. desacc.."=w2010) -> ("Impulses"=w2029:dbl[][])  [unwired: 5 in, 3 out]
            n998 = Array Size(array=w2029) -> (size(s)=w2028:i32[])
            n999 = Index Array(array=w2028, index=0) -> (element=w2026:i32)
            n1000 = Quotient & Remainder(x=w2026, y=w2025) -> (floor(x/y)=w2024:i32)  [unwired: 1 out]
            n1001 = for {
              N: w2024 -> [w2057]
              tunnel: w2029 -> [w2060]
              tunnel: w2023 -> [w2048]
              tunnel: w2022 -> [w2050]
              tunnel: w2021 -> [w2051]
              tunnel: [w2049] -> w2018 mode=indexing
              tunnel: w2015 -> [_]
              i -> [w2058]
              (unwired) 1000.0 ("y")
              n1002 = Add(x=w2057, y=w2058) -> (x+y=w2059:i32)
              n1003 = Index Array(array=w2060, index (row)=w2058) -> (element=w2052:dbl[])  [unwired: 1 in]
              n1004 = Index Array(array=w2060, index (row)=w2059) -> (element=w2053:dbl[])  [unwired: 1 in]
              n1005 = for {
                tunnel: w2048 -> [w2065]
                tunnel: [w2063] -> w2056 mode=indexing
                tunnel: w2053 -> [_] mode=indexing
                i -> [w2062]
                n1006 = Multiply(x=w2065, y=w2062) -> (x*y=w2061:dbl)
                n1007 = Build Array(1.0 ("Input Element"), w2061) -> (w2063:dbl[])
              }
              n1008 = call <userlib>:"Remove NaNs.vi"("Sinusoid"=w2056, "Response"=w2053, "Stimulus"=w2052) -> ("Response (out)"=w2054:dbl[], "Stimulus (out)"=w2055:dbl[])  [unwired: 1 out]
              n1009 = Reciprocal(x=w2048) -> (1/x=w2041:dbl)
              n1010 = Array Subset(array=w2054, index=w2051, length=w2050) -> (w2043:dbl[])
              n1011 = Array Subset(array=w2055, index=w2051, length=w2050) -> (w2042:dbl[])
              n1012 = Build Array(w2043, w2042) -> (w2046:dbl[][])
              n1013 = call "Differentiate 3D.vi"("Sample Rate 4"=w2041, "Data (in)"=w2046) -> ("Data (differentiated)"=w2038:dbl[][])  [unwired: 3 in]
              n1014 = Index Array(array=w2038, index (row)=0) -> (element=w2039:dbl[])  [unwired: 1 in]
              n1015 = Index Array(array=w2038, index (row)=1) -> (element=w2040:dbl[])  [unwired: 1 in]
              n1016 = Divide(x=w2039, y=w2040) -> (x/y=w2047:dbl[])
              n1017 = call-poly <vilib>:"Mean.vi"("X"=w2047) -> ("mean"=w2049:dbl)  [unwired: 1 out]
            }
            n1018 = call <vilib>:"Std Deviation and Variance.vi"("X"=w2018) -> ("mean"=w2020:dbl, "standard deviation"=w2019:dbl)  [unwired: 1 in, 1 out]
            n1019 = Divide(x=w2017, y=w2017) -> (x/y=w2016:dbl)
          }
        }
        n1020 = case shown="False" w1780 {
          tunnel: [w1816 w1820] -> w1803
          tunnel: w1802 -> [w1815 _]
          tunnel: w1800 -> [w1814 _]
          tunnel: w1788 -> [w1813 _]
          tunnel: w1787 -> [w1812 _]
          tunnel: w1786 -> [w1811 w1819]
          tunnel: w1783 -> [w1810 w1818]
          tunnel: w1782 -> [w1809 w1817]
          frame True {
            n1021 = Bundle By Name(cluster=w1811, "Transient Gains.Line Fit Response 2.Offset"=w1815, "Transient Gains.Line Fit Response 2.Slope"=w1812, "Transient Gains.Line Fit Stimulus 2.Offset"=w1814, "Transient Gains.Line Fit Stimulus 2.Slope"=w1813, "Transient Gains.Ga 2"=w1810, "Transient Gains.Ga SD 2"=w1809, "Fit Calculated"=TRUE) -> (w1816:T18)
          }
          frame False {
            n1022 = Bundle By Name(cluster=w1819, "Transient Gains.Ga 2"=w1818, "Transient Gains.Ga SD 2"=w1817) -> (w1820:T18)
          }
        }
      }
      frame "Calculate Transient Gv Gain" {
        n1023 = Unbundle By Name(w2122) -> ("Transient Gains.Snap Cursor"=w2128:u16, "Transient Gains.Gv Window"=w2130:u16, "Transient Gains.Stim.Onset"=w2131:dbl, "Data File.Sample Rate"=w2121:i32, "Transient Gains.Gv Stat."=w2115:u16, "Transient Gains.GV desaccading"=w2108:bool)
        n1024 = Equal?(x=u16 3, y=w2128) -> (x = y?=w2123:bool)
        n1025 = Reciprocal(x=w2121) -> (1/x=w2119:dbl)
        n1026 = case shown="2" w2130 {
          tunnel: [w2346 w2352 w2357] -> w2110
          tunnel: [w2345 w2351 w2356] -> w2125
          tunnel: w2131 -> [_ w2355 w2360]
          frame 0, Default {
            n1027 = stacked-sequence {
              tunnel: [_ w2349] -> w2345
              tunnel: [w2347 _] -> w2346
              frame #0 {
                n1028 = property on="Impulse Trace" class="WFGraph (strict)"("Active Cursor"=u32 0) -> ("Cursor.Cursor Position:Cursor X"=w2347:dbl)  [unwired: 2 in, 2 out]
              }
              frame #1 {
                n1029 = property on="Impulse Trace" class="WFGraph (strict)"("Active Cursor"=u32 1) -> ("Cursor.Cursor Position:Cursor X"=w2349:dbl)  [unwired: 2 in, 2 out]
              }
            }
          }
          frame 1 {
            n1030 = Add(x=w2355, y=200.0) -> (x+y=w2351:dbl)
            n1031 = Add(x=w2351, y=200.0) -> (x+y=w2352:dbl)
          }
          frame 2 {
            n1032 = Add(x=w2360, y=200.0) -> (x+y=w2356:dbl)
            n1033 = Add(x=w2356, y=500.0) -> (x+y=w2357:dbl)
          }
        }
        n1034 = Divide(x=w2121, y=1000.0) -> (x/y=w2129:dbl)
        n1035 = case shown="True" w2123 {
          tunnel: w2110 -> [_ w2340]
          tunnel: w2125 -> [_ w2339]
          frame False {
          }
          frame True {
            n1036 = stacked-sequence {
              tunnel: w2340 -> [w2341 _]
              tunnel: w2339 -> [_ w2343]
              frame #0 {
                n1037 = property on="Impulse Trace" class="WFGraph (strict)"("Cursor.Cursor Position:Cursor X"=w2341, "Active Cursor"=u32 0) -> ()  [unwired: 2 in, 2 out]
              }
              frame #1 {
                n1038 = property on="Impulse Trace" class="WFGraph (strict)"("Cursor.Cursor Position:Cursor X"=w2343, "Active Cursor"=u32 1) -> ()  [unwired: 2 in, 2 out]
              }
            }
          }
        }
        n1039 = Multiply(x=w2125, y=w2129) -> (x*y=w2126:dbl)
        n1040 = Multiply(x=w2110, y=w2129) -> (x*y=w2124:dbl)
        n1041 = Subtract(x=w2124, y=w2126) -> (x-y=w2132:dbl)
        n1042 = To Long Integer(number=w2126) -> (32bit integer=w2117:i32)
        n1043 = To Long Integer(number=w2132) -> (32bit integer=w2118:i32)
        n1044 = case shown="0" w2115 {
          tunnel: w2118 -> [w2153 w2203 w2293]
          tunnel: w2117 -> [w2152 w2202 w2292]
          tunnel: w2119 -> [w2151 w2204 w2294]
          tunnel: w2122 -> [w2150 w2213 w2303]
          tunnel: [w2149 w2201 w2291] -> w2120
          tunnel: [w2147 w2200 w2290] -> w2116
          tunnel: [w2138 w2188 0.0 ("mean")] -> w2114
          tunnel: [w2146 w2189 w2282] -> w2113
          tunnel: [w2137 w2190 0.0 ("mean")] -> w2112
          tunnel: [w2145 w2191 w2285] -> w2111
          tunnel: w2108 -> [_ w2182 w2279]
          frame 0 {
            w2148 = 0.0 ("standard deviation")
            n1045 = Unbundle By Name(w2150) -> ("Stimulus"=w2143:dbl[], "Response"=w2144:dbl[])
            n1046 = for {
              tunnel: w2151 -> [w2181]
              tunnel: [w2179] -> w2142 mode=indexing
              tunnel: w2144 -> [_] mode=indexing
              i -> [w2178]
              n1047 = Multiply(x=w2181, y=w2178) -> (x*y=w2177:dbl)
              n1048 = Build Array(1.0 ("Input Element"), w2177) -> (w2179:dbl[])
            }
            n1049 = Array Subset(array=w2144, index=w2152, length=w2153) -> (w2139:dbl[])
            n1050 = Array Subset(array=w2143, index=w2152, length=w2153) -> (w2140:dbl[])
            n1051 = Array Subset(array=w2142, index (row)=w2152, length (row)=w2153) -> (w2141:dbl[][])  [unwired: 2 in]
            n1052 = disable-structure shown="Enabled" {
              disable-tunnel: [w2164 w2172] -> w2146
              disable-tunnel: [w2163 w2174] -> w2145
              disable-tunnel: w2141 -> [w2161 w2170]
              disable-tunnel: w2140 -> [w2160 w2176]
              disable-tunnel: w2139 -> [w2159 w2175]
              disable-tunnel: [w2155 w2171] -> w2138
              disable-tunnel: [w2154 w2173] -> w2137
              frame Disabled {
                n1053 = call <userlib>:"Remove NaNs.vi"("Sinusoid"=w2161, "Response"=w2160, "Stimulus"=w2159) -> ("Sinusoid (out)"=w2156:dbl[][], "Response (out)"=w2157:dbl[], "Stimulus (out)"=w2158:dbl[])
                n1054 = call <vilib>:"General LS Linear Fit (obs).vi"("H"=w2156, "Y"=w2157) -> ("Coefficients"=w2162:dbl[])  [unwired: 3 in, 4 out]
                n1055 = call <vilib>:"General LS Linear Fit (obs).vi"("H"=w2156, "Y"=w2158) -> ("Coefficients"=w2165:dbl[])  [unwired: 3 in, 4 out]
                n1056 = Index Array(array=w2162, index=0 ("Index")) -> (element=w2164:dbl)
                n1057 = Index Array(array=w2162, index=1 ("Index")) -> (element=w2155:dbl)
                n1058 = Index Array(array=w2165, index=0 ("Index")) -> (element=w2163:dbl)
                n1059 = Index Array(array=w2165, index=1 ("Index")) -> (element=w2154:dbl)
              }
              frame Enabled {
                n1060 = call "linear fit NaN.vi"("Array 2"=w2170, "Array"=w2176) -> ("sloap"=w2171:dbl, "intercept"=w2172:dbl)  [unwired: 2 in]
                n1061 = call "linear fit NaN.vi"("Array 2"=w2170, "Array"=w2175) -> ("sloap"=w2173:dbl, "intercept"=w2174:dbl)  [unwired: 2 in]
              }
            }
            n1062 = Divide(x=w2145, y=w2146) -> (x/y=w2149:dbl)
            n1063 = Divide(x=w2148, y=w2148) -> (x/y=w2147:dbl)
          }
          frame 1, Default {
            n1064 = Unbundle By Name(w2213) -> ("Data File"=w2218:T25, "Impulse Positions"=w2217:T24, "desaccading parameters.Impulse dir"=w2216:bool, "desaccading parameters.Impulse Plane 2"=w2215:T28, "desacc"=w2214:T27)
            n1065 = local read "Parameter Impuls Series"() -> (w2211:T3)
            n1066 = local read "Interpolate"() -> (w2197:bool)
            n1067 = Array Size(array=w2211) -> (size(s)=w2206:i32)
            n1068 = local read "Trace Select"() -> (w2196:i32)
            n1069 = call "Couple Head Impulse Traces.vi"("Data Input"=w2218, "Impulse Positions"=w2217, "Trace Select"=w2196, "Impulse Direction +ve?"=w2216, "Impulse Plane"=w2215, "Mean and STD"=FALSE ("Mean Traces"), "Plot Selection 2"=w2211, "desacc"=w2214, "Interpolate"=w2197, "desacc."=FALSE, "man. desacc.."=w2182) -> ("Impulses"=w2210:dbl[][])  [unwired: 5 in, 3 out]
            n1070 = Array Size(array=w2210) -> (size(s)=w2209:i32[])
            n1071 = Index Array(array=w2209, index=0) -> (element=w2207:i32)
            n1072 = Quotient & Remainder(x=w2207, y=w2206) -> (floor(x/y)=w2205:i32)  [unwired: 1 out]
            n1073 = for {
              N: w2205 -> [w2247]
              tunnel: w2210 -> [w2250]
              tunnel: w2204 -> [w2246]
              tunnel: w2203 -> [w2245]
              tunnel: w2202 -> [w2244]
              tunnel: [w2243] -> w2186 mode=indexing
              tunnel: [w2242] -> w2185 mode=indexing
              tunnel: [w2241] -> w2187 mode=indexing
              tunnel: [w2240] -> w2184 mode=indexing
              i -> [w2248]
              n1074 = Add(x=w2247, y=w2248) -> (x+y=w2249:i32)
              n1075 = Index Array(array=w2250, index (row)=w2248) -> (element=w2238:dbl[])  [unwired: 1 in]
              n1076 = Index Array(array=w2250, index (row)=w2249) -> (element=w2239:dbl[])  [unwired: 1 in]
              n1077 = for {
                tunnel: w2246 -> [w2278]
                tunnel: [w2276] -> w2237 mode=indexing
                tunnel: w2239 -> [_] mode=indexing
                i -> [w2275]
                n1078 = Multiply(x=w2278, y=w2275) -> (x*y=w2274:dbl)
                n1079 = Build Array(1.0 ("Input Element"), w2274) -> (w2276:dbl[])
              }
              n1080 = Array Subset(array=w2239, index=w2244, length=w2245) -> (w2235:dbl[])
              n1081 = Array Subset(array=w2238, index=w2244, length=w2245) -> (w2234:dbl[])
              n1082 = Array Subset(array=w2237, index (row)=w2244, length (row)=w2245) -> (w2236:dbl[][])  [unwired: 2 in]
              n1083 = disable-structure shown="Enabled" {
                disable-tunnel: [w2262 w2273] -> w2243
                disable-tunnel: [w2261 w2272] -> w2242
                disable-tunnel: [w2260 w2270] -> w2241
                disable-tunnel: [w2259 w2271] -> w2240
                disable-tunnel: w2236 -> [w2257 w2269]
                disable-tunnel: w2235 -> [w2254 w2267]
                disable-tunnel: w2234 -> [w2253 w2268]
                frame Disabled {
                  n1084 = call <userlib>:"Remove NaNs.vi"("Sinusoid"=w2257, "Response"=w2253, "Stimulus"=w2254) -> ("Sinusoid (out)"=w2256:dbl[][], "Response (out)"=w2252:dbl[], "Stimulus (out)"=w2255:dbl[])
                  n1085 = call <vilib>:"General LS Linear Fit (obs).vi"("H"=w2256, "Y"=w2252) -> ("Coefficients"=w2251:dbl[])  [unwired: 3 in, 4 out]
                  n1086 = call <vilib>:"General LS Linear Fit (obs).vi"("H"=w2256, "Y"=w2255) -> ("Coefficients"=w2258:dbl[])  [unwired: 3 in, 4 out]
                  n1087 = Index Array(array=w2251, index=0 ("Index")) -> (element=w2261:dbl)
                  n1088 = Index Array(array=w2251, index=1 ("Index")) -> (element=w2262:dbl)
                  n1089 = Index Array(array=w2258, index=0 ("Index")) -> (element=w2259:dbl)
                  n1090 = Index Array(array=w2258, index=1 ("Index")) -> (element=w2260:dbl)
                }
                frame Enabled {
                  n1091 = call "linear fit NaN.vi"("Array 2"=w2269, "Array"=w2267) -> ("sloap"=w2270:dbl, "intercept"=w2271:dbl)  [unwired: 2 in]
                  n1092 = call "linear fit NaN.vi"("Array 2"=w2269, "Array"=w2268) -> ("sloap"=w2273:dbl, "intercept"=w2272:dbl)  [unwired: 2 in]
                }
              }
            }
            n1093 = Divide(x=w2184, y=w2185) -> (x/y=w2199:dbl[])
            n1094 = disable-structure shown="Enabled" {
              disable-tunnel: [w2225 w2226] -> w2193
              disable-tunnel: [w2224 w2227] -> w2192
              disable-tunnel: w2185 -> [w2223 w2226]
              disable-tunnel: w2186 -> [w2222 w2227]
              frame Disabled {
                n1095 = call <userlib>:"Remove NaNs.vi"("Response"=w2222, "Stimulus"=w2223) -> ("Response (out)"=w2224:dbl[], "Stimulus (out)"=w2225:dbl[])  [unwired: 1 in, 1 out]
              }
              frame Enabled {
              }
            }
            n1096 = disable-structure shown="Enabled" {
              disable-tunnel: [w2231 w2233] -> w2195
              disable-tunnel: [w2230 w2232] -> w2194
              disable-tunnel: w2184 -> [w2229 w2233]
              disable-tunnel: w2187 -> [w2228 w2232]
              frame Disabled {
                n1097 = call <userlib>:"Remove NaNs.vi"("Response"=w2228, "Stimulus"=w2229) -> ("Response (out)"=w2230:dbl[], "Stimulus (out)"=w2231:dbl[])  [unwired: 1 in, 1 out]
              }
              frame Enabled {
              }
            }
            n1098 = disable-structure shown="Enabled" {
              disable-tunnel: w2199 -> [w2220 w2221]
              disable-tunnel: [w2219 w2221] -> w2198
              frame Disabled {
                n1099 = call <userlib>:"Remove NaNs.vi"("Response"=w2220, "Stimulus"=w2220) -> ("Stimulus (out)"=w2219:dbl[])  [unwired: 1 in, 2 out]
              }
              frame Enabled {
              }
            }
            n1100 = call "mean_nan.vi"("Array"=w2195) -> ("Mean"=w2191:dbl)  [unwired: 10 in]
            n1101 = call "mean_nan.vi"("Array"=w2194) -> ("Mean"=w2190:dbl)  [unwired: 10 in]
            n1102 = call "mean_nan.vi"("Array"=w2193) -> ("Mean"=w2189:dbl)  [unwired: 10 in]
            n1103 = call "mean_nan.vi"("Array"=w2192) -> ("Mean"=w2188:dbl)  [unwired: 10 in]
            n1104 = call "standard deviation NaN.vi"("Array"=w2198) -> ("standard deviation"=w2200:dbl, "mean"=w2201:dbl)  [unwired: 2 in, 1 out]
          }
          frame 2 {
            n1105 = Unbundle By Name(w2303) -> ("Data File"=w2308:T25, "Impulse Positions"=w2307:T24, "desaccading parameters.Impulse dir"=w2306:bool, "desaccading parameters.Impulse Plane 2"=w2305:T28, "desacc"=w2304:T27)
            n1106 = local read "Parameter Impuls Series"() -> (w2301:T3)
            n1107 = local read "Interpolate"() -> (w2288:bool)
            n1108 = Array Size(array=w2301) -> (size(s)=w2296:i32)
            n1109 = local read "Trace Select"() -> (w2287:i32)
            n1110 = call "Couple Head Impulse Traces.vi"("Data Input"=w2308, "Impulse Positions"=w2307, "Trace Select"=w2287, "Impulse Direction +ve?"=w2306, "Impulse Plane"=w2305, "Mean and STD"=FALSE ("Mean Traces"), "Plot Selection 2"=w2301, "desacc"=w2304, "Interpolate"=w2288, "desacc."=FALSE, "man. desacc.."=w2279) -> ("Impulses"=w2300:dbl[][])  [unwired: 5 in, 3 out]
            n1111 = Array Size(array=w2300) -> (size(s)=w2299:i32[])
            n1112 = Index Array(array=w2299, index=0) -> (element=w2297:i32)
            n1113 = Quotient & Remainder(x=w2297, y=w2296) -> (floor(x/y)=w2295:i32)  [unwired: 1 out]
            n1114 = for {
              N: w2295 -> [w2323]
              tunnel: w2300 -> [w2326]
              tunnel: w2294 -> [w2319]
              tunnel: w2293 -> [w2317]
              tunnel: w2292 -> [w2318]
              tunnel: [w2313] -> w2289 mode=indexing
              tunnel: [w2311] -> w2286 mode=indexing
              tunnel: [w2309] -> w2283 mode=indexing
              i -> [w2324]
              n1115 = Add(x=w2323, y=w2324) -> (x+y=w2325:i32)
              n1116 = Index Array(array=w2326, index (row)=w2324) -> (element=w2320:dbl[])  [unwired: 1 in]
              n1117 = Index Array(array=w2326, index (row)=w2325) -> (element=w2321:dbl[])  [unwired: 1 in]
              n1118 = for {
                tunnel: w2319 -> [w2338]
                tunnel: [w2336] -> w2322 mode=indexing
                tunnel: w2321 -> [_] mode=indexing
                i -> [w2335]
                n1119 = Multiply(x=w2338, y=w2335) -> (x*y=w2334:dbl)
                n1120 = Build Array(1.0 ("Input Element"), w2334) -> (w2336:dbl[])
              }
              n1121 = disable-structure shown="Enabled" {
                disable-tunnel: w2322 -> [w2331 _]
                disable-tunnel: w2321 -> [w2330 w2332]
                disable-tunnel: w2320 -> [w2329 w2333]
                disable-tunnel: [w2328 w2333] -> w2316
                disable-tunnel: [w2327 w2332] -> w2315
                frame Disabled {
                  n1122 = call <userlib>:"Remove NaNs.vi"("Sinusoid"=w2331, "Response"=w2330, "Stimulus"=w2329) -> ("Response (out)"=w2327:dbl[], "Stimulus (out)"=w2328:dbl[])  [unwired: 1 out]
                }
                frame Enabled {
                }
              }
              n1123 = Array Subset(array=w2315, index=w2318, length=w2317) -> (w2312:dbl[])
              n1124 = Array Subset(array=w2316, index=w2318, length=w2317) -> (w2310:dbl[])
              n1125 = Divide(x=w2312, y=w2310) -> (x/y=w2314:dbl[])
              n1126 = call "mean_nan.vi"("Array"=w2310) -> ("Mean"=w2309:dbl)  [unwired: 10 in]
              n1127 = call "mean_nan.vi"("Array"=w2312) -> ("Mean"=w2311:dbl)  [unwired: 10 in]
              n1128 = call "mean_nan.vi"("Array"=w2314) -> ("Mean"=w2313:dbl)  [unwired: 10 in]
            }
            n1129 = call "mean_nan.vi"("Array"=w2283) -> ("Mean"=w2282:dbl)  [unwired: 10 in]
            n1130 = call "standard deviation NaN.vi"("Array"=w2289) -> ("standard deviation"=w2290:dbl, "mean"=w2291:dbl)  [unwired: 2 in, 1 out]
            n1131 = call "mean_nan.vi"("Array"=w2286) -> ("Mean"=w2285:dbl)  [unwired: 10 in]
          }
        }
        n1132 = Bundle By Name(cluster=w2122, "Gv Line Fit Stimulus.Offset"=w2111, "Gv Line Fit Stimulus.Slope"=w2112, "Gv Line Fit Response.Offset"=w2113, "Gv Line Fit Response.Slope"=w2114, "Transient Gains.Gv"=w2120, "Transient Gains.Gv SD"=w2116) -> (w2134:T18)
      }
      frame "Polynomial Fit" {
        n1133 = Unbundle By Name(w2386) -> ("Transient Gains.Poly. Window"=w2395:u16, "Transient Gains.Stim.Onset"=w2394:dbl, "Stimulus"=w2371:dbl[], "Response"=w2375:dbl[], "Data File.Sample Rate"=w2392:i32, "Transient Gains.Ord."=w2388:i32, "Transient Gains.Mirror"=w2365:bool)
        n1134 = Increment(x=w2388) -> (x+1=w2376:i32)
        n1135 = case shown="2" w2395 {
          tunnel: [w2428 w2435 w2440 w2445] -> w2401
          tunnel: [w2429 w2434 w2439 w2444] -> w2400
          tunnel: w2394 -> [_ w2436 w2441 w2446]
          frame 0, Default {
            n1136 = stacked-sequence {
              tunnel: [_ w2432] -> w2429
              tunnel: [w2430 _] -> w2428
              frame #0 {
                n1137 = property on="Impulse Trace" class="WFGraph (strict)"("Active Cursor"=u32 0) -> ("Cursor.Cursor Position:Cursor X"=w2430:dbl)  [unwired: 2 in, 2 out]
              }
              frame #1 {
                n1138 = property on="Impulse Trace" class="WFGraph (strict)"("Active Cursor"=u32 1) -> ("Cursor.Cursor Position:Cursor X"=w2432:dbl)  [unwired: 2 in, 2 out]
              }
            }
          }
          frame 1 {
            n1139 = Add(x=w2436, y=10.0) -> (x+y=w2434:dbl)
            n1140 = Add(x=w2434, y=30.0) -> (x+y=w2435:dbl)
          }
          frame 2 {
            n1141 = Add(x=w2441, y=5.0) -> (x+y=w2439:dbl)
            n1142 = Add(x=w2439, y=30.0) -> (x+y=w2440:dbl)
          }
          frame 3 {
            n1143 = Add(x=w2446, y=0.0) -> (x+y=w2444:dbl)
            n1144 = Add(x=w2444, y=30.0) -> (x+y=w2445:dbl)
          }
        }
        n1145 = Divide(x=w2392, y=1000.0) -> (x/y=w2393:dbl)
        n1146 = Multiply(x=w2400, y=w2393) -> (x*y=w2389:dbl)
        n1147 = Multiply(x=w2401, y=w2393) -> (x*y=w2390:dbl)
        n1148 = Subtract(x=w2390, y=w2389) -> (x-y=w2391:dbl)
        n1149 = To Long Integer(number=w2389) -> (32bit integer=w2373:i32)
        n1150 = To Long Integer(number=w2391) -> (32bit integer=w2372:i32)
        n1151 = Array Subset(array=w2375, index=w2373, length=w2372) -> (w2367:dbl[])
        n1152 = Array Subset(array=w2371, index=w2373, length=w2372) -> (w2368:dbl[])
        n1153 = case shown="True" w2365 {
          tunnel: [w2405 w2409] -> w2366
          tunnel: w2367 -> [w2405 w2408]
          frame False {
          }
          frame True {
            n1154 = Reverse 1D Array(array=w2408) -> (reversed array=w2407:dbl[])
            n1155 = Negate(x=w2407) -> (-x=w2406:dbl[])
            n1156 = Build Array (concatenate)(w2406, w2408) -> (w2409:dbl[])
          }
        }
        n1157 = case shown="True" w2365 {
          tunnel: [w2410 w2414] -> w2369
          tunnel: w2368 -> [w2410 w2413]
          frame False {
          }
          frame True {
            n1158 = Reverse 1D Array(array=w2413) -> (reversed array=w2412:dbl[])
            n1159 = Negate(x=w2412) -> (-x=w2411:dbl[])
            n1160 = Build Array (concatenate)(w2411, w2413) -> (w2414:dbl[])
          }
        }
        n1161 = for {
          tunnel: [w2451] -> w2364 mode=indexing
          tunnel: w2376 -> [w2450]
          tunnel: w2369 -> [w2449] mode=indexing
          n1162 = for {
            N: w2450 -> [_]
            tunnel: w2449 -> [w2454]
            shift-right: [w2455] -> w2451
            shift-left: dbl[] [] -> [w2457]
            i -> [w2453]
            n1163 = Power Of X(1:w2454, 2:w2453) -> (0:w2456:dbl)
            n1164 = Build Array (concatenate)(w2457, w2456) -> (w2455:dbl[])
          }
        }
        n1165 = call <userlib>:"Remove NaNs.vi"("Sinusoid"=w2364, "Response"=w2366, "Stimulus"=w2369) -> ("Sinusoid (out)"=w2374:dbl[][], "Response (out)"=w2370:dbl[])  [unwired: 1 out]
        n1166 = call <vilib>:"General LS Linear Fit (obs).vi"("H"=w2374, "Y"=w2370) -> ("Coefficients"=w2387:dbl[], "mse"=w2363:dbl)  [unwired: 3 in, 3 out]
        n1167 = Natural Logarithm(1:w2363) -> (0:w2380:dbl)
        n1168 = Natural Logarithm(1:w2372) -> (0:w2384:dbl)
        n1169 = for {
          tunnel: w2387 -> [w2425] mode=indexing
          shift-right: [w2418] -> w2377
          shift-left: "" -> [w2415]
          i -> [w2421]
          n1170 = Equal To 0?(x=w2421) -> (x = 0?=w2420:bool)
          n1171 = Format Value(format string="%d", value (0)=w2421) -> (output string=w2422:string)  [unwired: 1 in]
          n1172 = Format Value(format string="%^.2e ", value (0)=w2425) -> (output string=w2424:string)  [unwired: 1 in]
          n1173 = case shown="True" w2420 {
            tunnel: [" + " ""] -> w2419
            frame False {
            }
            frame True {
            }
          }
          n1174 = Concatenate Strings(w2415, w2419, w2424, "Hv^", w2422) -> (w2418:string)
        }
        n1175 = Multiply(x=w2384, y=w2376) -> (x*y=w2383:dbl)
        n1176 = Add(x=w2372, y=w2372) -> (x+y=w2382:i32)
        n1177 = local read "Transient Gains"() -> (w2396:T9)
        n1178 = Divide(x=w2383, y=w2382) -> (x/y=w2381:dbl)
        n1179 = Add(x=w2380, y=w2381) -> (x+y=w2379:dbl)
        n1180 = Bundle By Name(cluster=w2386, "Transient Gains.Poly Equation"=w2377, "Transient Gains.BIC"=w2379, "Transient Gains.MSE"=w2363) -> (w2385:T18)
        n1181 = Unbundle By Name(w2385) -> ("Transient Gains.MSE"=w2362:dbl, "Transient Gains.BIC"=w2398:dbl, "Transient Gains.Poly Equation"=w2399:string)
        n1182 = Bundle By Name(cluster=w2396, "MSE"=w2362, "BIC"=w2398, "Poly Equation"=w2399) -> (w2397:T9)
        n1183 = local write "Transient Gains"(w2397) -> ()
      }
      frame "Make Transient Fits & Equations" {
        w2494 = "%.2f " ("format string")
        w2493 = "t "
        w2496 = " + "
        n1184 = Unbundle By Name(w2503) -> ("Data File"=w2511:T25, "Impulse Positions"=w2512:T24, "desaccading parameters.Impulse dir"=w2513:bool, "Data File.Sample Rate"=w2509:i32, "desaccading parameters.Impulse Plane 2"=w2514:T28, "desacc"=w2515:T27, "Transient Gains.Line Fit Response"=w2468:cluster{"Offset":dbl, "Slope":dbl}, "Transient Gains.Line Fit Stimulus"=w2469:cluster{"Offset":dbl, "Slope":dbl}, "Transient Gains"=w2490:T9, "Gv Line Fit Stimulus"=w2482:cluster{"Offset":dbl, "Slope":dbl}, "Gv Line Fit Response"=w2481:cluster{"Offset":dbl, "Slope":dbl}, "Transient Gains.Line Fit Response 2"=w2465:cluster{"Offset":dbl, "Slope":dbl}, "Transient Gains.Line Fit Stimulus 2"=w2464:cluster{"Offset":dbl, "Slope":dbl}, "Transient Gains.Line Fit Res Latency"=w2463:cluster{"Offset":dbl, "Slope":dbl}, "Transient Gains.Line Fit Stim Latency"=w2462:cluster{"Offset":dbl, "Slope":dbl}, "Transient Gains.Snap Cursor"=w2472:u16, "Transient Gains.GA Line active"=w2471:i32, "Transient Gains.Stim.Onset"=w2459:dbl)
        n1185 = case shown="4" w2472 {
          selector: w2472 -> [_ w2523 _ w2525]
          tunnel: w2471 -> [w2522 _ w2524 _]
          tunnel: [w2522 w2523 w2524 w2525] -> w2470
          frame 0, Default {
          }
          frame 1, 2 {
          }
          frame 3 {
          }
          frame 4 {
          }
        }
        n1186 = local read "Trace Select"() -> (w2483:i32)
        n1187 = local read "Parameter Impuls Series"() -> (w2510:T3)
        n1188 = Unbundle By Name(w2503) -> ("Transient Gains.Line Fit Response.Offset"=w2487:dbl, "Transient Gains.Line Fit Response.Slope"=w2486:dbl, "Transient Gains.Line Fit Stimulus.Offset"=w2488:dbl, "Transient Gains.Line Fit Stimulus.Slope"=w2485:dbl)
        n1189 = case shown="1, Default" w2470 {
          tunnel: w2468 -> [w2527 _ _ _]
          tunnel: w2469 -> [w2526 _ _ _]
          tunnel: [w2526 w2528 w2530 w2532] -> w2467
          tunnel: [w2527 w2529 w2531 w2533] -> w2466
          tunnel: w2465 -> [_ w2529 _ _]
          tunnel: w2464 -> [_ w2528 _ _]
          tunnel: w2463 -> [_ _ w2531 w2533]
          tunnel: w2462 -> [_ _ w2530 w2532]
          frame 1, Default {
          }
          frame 2 {
          }
          frame 3 {
          }
          frame 4 {
          }
        }
        n1190 = Reciprocal(x=w2509) -> (1/x=w2461:dbl)
        n1191 = Unbundle By Name(w2482) -> ("Offset"=w2477:dbl, "Slope"=w2478:dbl)
        n1192 = Unbundle By Name(w2481) -> ("Offset"=w2480:dbl, "Slope"=w2479:dbl)
        n1193 = local read "Interpolate"() -> (w2484:bool)
        n1194 = call "Couple Head Impulse Traces.vi"("Data Input"=w2511, "Impulse Positions"=w2512, "Trace Select"=w2483, "Impulse Direction +ve?"=w2513, "Impulse Plane"=w2514, "Mean and STD"=TRUE, "Plot Selection 2"=w2510, "desacc"=w2515, "Interpolate"=w2484) -> ("Mean and STD"=w2516:dbl[][])  [unwired: 7 in, 3 out]
        n1195 = Array Size(array=w2516) -> (size(s)=w2518:i32[])
        n1196 = Divide(x=w2459, y=1000.0) -> (x/y=w2460:dbl)
        n1197 = Unbundle By Name(w2467) -> ("Offset"=w2505:dbl, "Slope"=w2507:dbl)
        n1198 = Unbundle By Name(w2466) -> ("Offset"=w2506:dbl, "Slope"=w2508:dbl)
        n1199 = Index Array(array=w2518, index=1) -> (element=w2473:i32)
        n1200 = for {
          N: w2473 -> [_]
          tunnel: w2461 -> [w2578]
          tunnel: w2508 -> [w2577]
          tunnel: w2507 -> [w2576]
          tunnel: w2506 -> [w2573]
          tunnel: w2505 -> [w2572]
          tunnel: [w2566] -> w2501 mode=indexing
          tunnel: [w2565] -> w2502 mode=indexing
          tunnel: w2460 -> [w2561]
          i -> [w2579]
          n1201 = Multiply(x=w2579, y=w2578) -> (x*y=w2564:dbl)
          n1202 = Multiply(x=w2564, y=w2577) -> (x*y=w2575:dbl)
          n1203 = Multiply(x=w2564, y=w2576) -> (x*y=w2574:dbl)
          n1204 = Add(x=w2573, y=w2575) -> (x+y=w2568:dbl)
          n1205 = Add(x=w2572, y=w2574) -> (x+y=w2567:dbl)
          n1206 = Add(x="Line Range +/- GA", y=w2561) -> (x+y=w2562:dbl)
          n1207 = Subtract(x=w2561, y=0.005) -> (x-y=w2559:dbl)
          n1208 = In Range and Coerce(upper limit=w2562, x=w2564, lower limit=w2559) -> (In Range?=w2571:bool)  [unwired: 1 out]
          n1209 = In Range and Coerce(upper limit=w2562, x=w2564, lower limit=w2559) -> (In Range?=w2570:bool)  [unwired: 1 out]
          n1210 = Or(x=w2571, y=w2570) -> (x .or. y?=w2569:bool)
          n1211 = case shown="True" w2569 {
            tunnel: w2568 -> [_ w2583]
            tunnel: w2567 -> [_ w2582]
            tunnel: [w2580 w2583] -> w2566
            tunnel: [w2580 w2582] -> w2565
            frame False {
              w2581 = 0.0 ("x")
              n1212 = Divide(x=w2581, y=w2581) -> (x/y=w2580:dbl)
            }
            frame True {
            }
          }
        }
        n1213 = for {
          N: w2473 -> [_]
          tunnel: w2461 -> [w2553]
          tunnel: w2478 -> [w2552]
          tunnel: w2479 -> [w2551]
          tunnel: w2477 -> [w2548]
          tunnel: w2480 -> [w2547]
          tunnel: [w2541] -> w2476 mode=indexing
          tunnel: [w2540] -> w2475 mode=indexing
          tunnel: w2460 -> [w2539]
          i -> [w2554]
          n1214 = Multiply(x=w2554, y=w2553) -> (x*y=w2535:dbl)
          n1215 = Multiply(x=w2535, y=w2552) -> (x*y=w2550:dbl)
          n1216 = Multiply(x=w2535, y=w2551) -> (x*y=w2549:dbl)
          n1217 = Add(x=w2539, y=0.2) -> (x+y=w2534:dbl)
          n1218 = Add(x=w2548, y=w2550) -> (x+y=w2543:dbl)
          n1219 = Add(x=w2547, y=w2549) -> (x+y=w2542:dbl)
          n1220 = Add(x="Line Range +/- GV", y=w2534) -> (x+y=w2536:dbl)
          n1221 = In Range and Coerce(upper limit=w2536, x=w2535, lower limit=w2534) -> (In Range?=w2546:bool)  [unwired: 1 out]
          n1222 = In Range and Coerce(upper limit=w2536, x=w2535, lower limit=w2534) -> (In Range?=w2545:bool)  [unwired: 1 out]
          n1223 = Or(x=w2546, y=w2545) -> (x .or. y?=w2544:bool)
          n1224 = case shown="True" w2544 {
            tunnel: w2543 -> [_ w2558]
            tunnel: w2542 -> [_ w2557]
            tunnel: [w2555 w2558] -> w2541
            tunnel: [w2555 w2557] -> w2540
            frame False {
              w2556 = 0.0 ("x")
              n1225 = Divide(x=w2556, y=w2556) -> (x/y=w2555:dbl)
            }
            frame True {
            }
          }
        }
        n1226 = Format Value(format string=w2494, value (0)=w2487) -> (output string=w2499:string)  [unwired: 1 in]
        n1227 = Format Value(format string=w2494, value (0)=w2486) -> (output string=w2498:string)  [unwired: 1 in]
        n1228 = Format Value(format string=w2494, value (0)=w2488) -> (output string=w2497:string)  [unwired: 1 in]
        n1229 = Format Value(format string=w2494, value (0)=w2485) -> (output string=w2495:string)  [unwired: 1 in]
        n1230 = Concatenate Strings(w2499, w2496, w2498, w2493) -> (w2492:string)
        n1231 = Concatenate Strings(w2497, w2496, w2495, w2493) -> (w2491:string)
        n1232 = Bundle By Name(cluster=w2490, "Reponse Equation"=w2492, "Stimulus Equation"=w2491) -> (w2489:T9)
        n1233 = local write "Transient Gains"(w2489) -> ()
        n1234 = Build Array(w2501, w2502, w2476, w2475) -> (w2500:dbl[][])
        n1235 = Bundle By Name(cluster=w2503, "Fitted Curves"=w2500, "Transient Gains"=w2489, "Transient Gains.GA Line active"=w2470) -> (w2504:T18)
      }
      frame "Calculate Mean" {
        n1236 = Unbundle By Name(w2601) -> ("Impulse Manager"=w2600:refnum<class "Impulse Manager.lvclass">)
        n1237 = property on="Impulse Trace" class="WFGraph (strict)"() -> ("CrsrList"=w2595:T35)  [unwired: 2 in, 2 out]
        n1238 = Index Array(array=w2595) -> (element #1=w2594:T36, element #2=w2593:T36)  [unwired: 2 in]
        n1239 = call-dynamic "Get Data.vi"("index"=0, "Impulse Manager in"=w2600) -> ("Data out"=w2597:dbl[][], "Impulse Manager out"=w2589:refnum<class "Impulse Manager.lvclass">)  [unwired: 6 in, 2 out]
        n1240 = Unbundle By Name(w2593) -> ("Position.X"=w2590:dbl)
        n1241 = Unbundle By Name(w2594) -> ("Position.X"=w2591:dbl)
        n1242 = local read "Mean Stats Method"() -> (w2584:T7)
        n1243 = call-dynamic "Get Data.vi"("index"=1, "Impulse Manager in"=w2589) -> ("Data out"=w2586:dbl[][], "Impulse Manager out"=w2588:refnum<class "Impulse Manager.lvclass">)  [unwired: 6 in, 2 out]
        n1244 = Build Array(w2591, w2590) -> (w2585:dbl[])
        n1245 = call-dynamic "Get Sample Rate.vi"("Impulse Manager in"=w2588) -> ("Sample Rate"=w2592:i32)  [unwired: 8 in, 2 out]
        n1246 = call "Constructor.vi"("Sample Rate"=w2592) -> ("Mean Fit out"=w2598:refnum<class "Mean Fit.lvclass">)  [unwired: 10 in]
        n1247 = call "CalculateFit.vi"("Stat Method"=w2584, "X Range"=w2585, "Response in"=w2586, "Stimulus in"=w2597, "Mean Fit in"=w2598) -> ("Mean Fit out"=w2596:refnum<class "Mean Fit.lvclass">)  [unwired: 6 in]
        n1248 = Bundle By Name(cluster=w2601, "Mean Fit"=w2596) -> (w2603:T18)
      }
      frame "Calculate Exponential" {
        n1249 = Unbundle By Name(w2625) -> ("Impulse Manager"=w2624:refnum<class "Impulse Manager.lvclass">)
        n1250 = property on="Impulse Trace" class="WFGraph (strict)"() -> ("CrsrList"=w2622:T35)  [unwired: 2 in, 2 out]
        n1251 = call-dynamic "Get Data.vi"("index"=0, "Impulse Manager in"=w2624) -> ("Data out"=w2610:dbl[][], "Impulse Manager out"=w2617:refnum<class "Impulse Manager.lvclass">)  [unwired: 6 in, 2 out]
        n1252 = Index Array(array=w2622) -> (element #1=w2621:T36, element #2=w2620:T36)  [unwired: 2 in]
        n1253 = Unbundle By Name(w2620) -> ("Position.X"=w2618:dbl, "Position.Y"=w2607:dbl)
        n1254 = Unbundle By Name(w2621) -> ("Position.X"=w2619:dbl, "Position.Y"=w2608:dbl)
        n1255 = call-dynamic "Get Data.vi"("index"=1, "Impulse Manager in"=w2617) -> ("Data out"=w2609:dbl[][], "Impulse Manager out"=w2616:refnum<class "Impulse Manager.lvclass">)  [unwired: 6 in, 2 out]
        n1256 = call-dynamic "Get Sample Rate.vi"("Impulse Manager in"=w2616) -> ("Sample Rate"=w2614:i32)  [unwired: 8 in, 2 out]
        n1257 = Build Array(w2619, w2618) -> (w2613:dbl[])
        n1258 = Build Array(w2608, w2607) -> (w2606:dbl[])
        n1259 = call "Constructor.vi"("Y Range"=w2606, "X Range"=w2613, "Sample Rate"=w2614) -> ("Exponential Fit out"=w2612:refnum<class "Exponential Fit.lvclass">)  [unwired: 8 in]
        n1260 = call "Calculate Fit.vi"("Response in"=w2609, "Stimulus in"=w2610, "Exponential Fit in"=w2612) -> ("Exponential Fit out"=w2611:refnum<class "Exponential Fit.lvclass">)  [unwired: 8 in]
        n1261 = Bundle By Name(cluster=w2625, "Exponential Fit"=w2611) -> (w2627:T18)
      }
      frame "Calculate Head Impulse" {
        n1262 = Unbundle By Name(w2634) -> ("Impulse Manager"=w2648:refnum<class "Impulse Manager.lvclass">)
        n1263 = call-dynamic "Get Data.vi"("index"=0, "Impulse Manager in"=w2648) -> ("error out"=w2643:errorcluster, "Data out"=w2637:dbl[][], "Impulse Manager out"=w2646:refnum<class "Impulse Manager.lvclass">)  [unwired: 6 in, 1 out]
        n1264 = local read "Head Impulse Fit Controls"() -> (w2630:T12)
        n1265 = call-dynamic "Get Data.vi"("error in (no error)"=w2643, "index"=1, "Impulse Manager in"=w2646) -> ("error out"=w2642:errorcluster, "Data out"=w2638:dbl[][], "Impulse Manager out"=w2645:refnum<class "Impulse Manager.lvclass">)  [unwired: 5 in, 1 out]
        n1266 = call-dynamic "Get Sample Rate.vi"("error in (no error)"=w2642, "Impulse Manager in"=w2645) -> ("error out"=w2641:errorcluster, "Sample Rate"=w2640:i32)  [unwired: 7 in, 1 out]
        n1267 = call "Constructor.vi"("error in (no error)"=w2641, "Fit Controls"=w2630, "Sample Rate"=w2640) -> ("error out"=w2639:errorcluster, "Head Impulse Fit out"=w2636:refnum<class "Head Impulse Fit.lvclass">)  [unwired: 7 in]
        n1268 = call "CalculateFit.vi"("error in (no error)"=w2639, "Response in"=w2638, "Stimulus in"=w2637, "Head Impulse Fit in"=w2636) -> ("Head Impulse Fit out"=w2635:refnum<class "Head Impulse Fit.lvclass">)  [unwired: 6 in, 1 out]
        n1269 = Bundle By Name(cluster=w2634, "HI Fit"=w2635) -> (w2633:T18)
      }
      frame "Save All Gain And Phase To Excel" {
        # "Write a new record for each impulse rather than the usual mean & standard deviation"
        # "Just get whole-fit sinusoids"
        n1270 = Unbundle By Name(w2659) -> ("Sine Fit"=w2668:refnum<class "Sinusoidal Fit.lvclass">[])
        n1271 = Unbundle By Name(w2652) -> ("filename"=w2658:string)
        n1272 = Index Array(array=w2668) -> (element=w2667:refnum<class "Sinusoidal Fit.lvclass">)  [unwired: 1 in]
        n1273 = Unbundle By Name(w2652) -> ("Excel"=w2653:refnum<class "Excel.lvclass">)
        n1274 = call-dynamic "Get Sample Rate.vi"("Abstract Fit in"=w2667) -> ("error out"=w2664:errorcluster, "Sample Rate"=w2662:i32, "Abstract Fit out"=w2666:refnum<class "Sinusoidal Fit.lvclass">)  [unwired: 8 in]
        n1275 = call "Read Impulse Positions.vi"("error in (no error)"=w2664, "Abstract Fit in"=w2666) -> ("error out"=w2663:errorcluster, "Impulse Positions"=w2661:T34, "Abstract Fit out"=w2665:refnum<class "Sinusoidal Fit.lvclass">)  [unwired: 7 in]
        n1276 = call <userlib>:"Open.vi"("Worksheet Name (Sheet1)"="All Sinusoid G&P", "Excel in"=w2653) -> ("error out"=w2675:errorcluster, "Excel out"=w2676:refnum<class "Excel.lvclass">)  [unwired: 8 in]
        n1277 = call "Read All Gain and Phase.vi"("error in (no error)"=w2663, "Sinusoidal Fit in"=w2665) -> ("All Gain and Phase"=w2660:cluster{"Gain":dbl, "Phase":dbl}[])  [unwired: 7 in, 2 out]
        n1278 = call <userlib>:"Write.vi"("error in (no error)"=w2675, "Cell (Append to next row)"=cluster{"Row":i32, "Col":i32} {"Row"=0, "Col"=0}, "Data"=string[] ["File", "Onset", "Gain", "Phase"], "Excel in"=w2676) -> ("error out"=w2671:errorcluster, "Excel out"=w2672:refnum<class "Excel.lvclass">)  [unwired: 5 in, 1 out]
        n1279 = for {
          tunnel: w2662 -> [w2693]
          tunnel: w2661 -> [w2694] mode=indexing
          tunnel: w2660 -> [w2695] mode=indexing
          tunnel: [w2688] -> w2656 mode=indexing
          tunnel: w2658 -> [w2687]
          tunnel: [w2686] -> w2657 mode=indexing
          # "New record for each impulse"
          n1280 = Unbundle By Name(w2694) -> ("Start"=w2686:i32)
          n1281 = Unbundle By Name(w2695) -> ("Gain"=w2692:dbl, "Phase"=w2691:dbl)
          n1282 = Divide(x=w2686, y=w2693) -> (x/y=w2685:dbl)
          n1283 = Build Array(w2685, w2692, w2691) -> (w2690:dbl[])
          n1284 = Number To Fractional String(number=w2690) -> (F-format string=w2689:string[])  [unwired: 3 in]
          n1285 = Build Array (concatenate)(w2687, w2689) -> (w2688:string[])
        }
        n1286 = call-poly <userlib>:"Remove Duplicates from 1D Array__ogtk.vi"("Input Array"=w2657) -> ("indices of removed elements"=w2655:i32[])  [unwired: 1 out]
        n1287 = for {
          tunnel: w2656 -> [w2681] mode=indexing
          tunnel: w2655 -> [w2684]
          tunnel: [w2681] -> w2654 mode=indexing if=w2680
          i -> [w2683]
          # "Remove duplicate impulses"
          n1288 = Search 1D Array(1D array=w2684, element=w2683) -> (index of element=w2682:i32)  [unwired: 1 in]
          n1289 = Less Than 0?(x=w2682) -> (x < 0?=w2680:bool)
        }
        n1290 = call <userlib>:"Write.vi"("error in (no error)"=w2671, "Data"=w2654, "Excel in"=w2672) -> ("error out"=w2669:errorcluster, "Excel out"=w2670:refnum<class "Excel.lvclass">)  [unwired: 6 in, 1 out]
        n1291 = call <userlib>:"Save.vi"("error in (no error)"=w2669, "Excel in"=w2670) -> ("Excel out"=w2650:refnum<class "Excel.lvclass">)  [unwired: 7 in, 2 out]
        n1292 = Bundle By Name(cluster=w2652, "Excel"=w2650) -> (w2651:T1)
      }
      frame "Calculate Impulse Latency" {
        w2744 = TRUE  # Mean and STD
        w2755 = FALSE  # Mean and STD
        # "Resp."
        # "Stim."
        # "Determine the threshold for head and eye onset"
        # "Resp."
        # "Stim."
        # "Retreieve mean impulse data"
        # "Retreieve individual impulse data"
        n1293 = local read "Impulse Latency Controls"() -> (w2720:T15)
        n1294 = property on="Impulse Trace" class="WFGraph (strict)"() -> ("CrsrList"=w2706:T35)  [unwired: 2 in, 2 out]
        n1295 = Unbundle By Name(w2736) -> ("Data File"=w2737:T25, "Impulse Positions"=w2738:T24, "desaccading parameters.Impulse dir"=w2745:bool, "Data File.Sample Rate"=w2708:i32, "desaccading parameters.Impulse Plane 2"=w2741:T28, "desacc"=w2742:T27)
        n1296 = Unbundle By Name(w2736) -> ("Data File"=w2762:T25, "Impulse Positions"=w2761:T24, "desaccading parameters.Impulse dir"=w2754:bool, "desaccading parameters.Impulse Plane 2"=w2758:T28, "desacc"=w2757:T27)  [unwired: 1 out]
        n1297 = Index Array(array=w2706) -> (element #1=w2705:T36, element #2=w2704:T36)  [unwired: 2 in]
        n1298 = local read "Parameter Impuls Series"() -> (w2743:T3)
        n1299 = local read "Parameter Impuls Series"() -> (w2756:T3)
        n1300 = Unbundle By Name(w2705) -> ("Position.X"=w2703:dbl)
        n1301 = Unbundle By Name(w2704) -> ("Position.X"=w2702:dbl)
        n1302 = local read "Trace Select"() -> (w2739:i32)
        n1303 = local read "Trace Select"() -> (w2760:i32)
        n1304 = local read "Interpolate"() -> (w2740:bool)
        n1305 = Unbundle By Name(w2720) -> ("Only After\nCursor?"=w2699:bool, "Max Valid Latency"=w2719:dbl, "Min Valid Latency"=w2718:dbl)
        n1306 = local read "Interpolate"() -> (w2759:bool)
        n1307 = Max & Min(x=w2703, y=w2702) -> (min(x,y)=w2701:dbl)  [unwired: 1 out]
        n1308 = local read "Impulse Latency Controls"() -> (w2750:T15)
        n1309 = call "Couple Head Impulse Traces.vi"("Data Input"=w2737, "Impulse Positions"=w2738, "Trace Select"=w2739, "Impulse Direction +ve?"=w2745, "Impulse Plane"=w2741, "Mean and STD"=w2744, "Plot Selection 2"=w2743, "desacc"=w2742, "Interpolate"=w2740) -> ("Mean and STD"=w2735:dbl[][])  [unwired: 7 in, 3 out]
        n1310 = call "Couple Head Impulse Traces.vi"("Data Input"=w2762, "Impulse Positions"=w2761, "Trace Select"=w2760, "Impulse Direction +ve?"=w2754, "Impulse Plane"=w2758, "Mean and STD"=w2755, "Plot Selection 2"=w2756, "desacc"=w2757, "Interpolate"=w2759) -> ("No Impulses"=w2752:i32, "Impulses"=w2753:dbl[][])  [unwired: 7 in, 2 out]
        n1311 = Divide(x=1000.0, y=w2708) -> (x/y=w2700:dbl)
        n1312 = Divide(x=w2701, y=w2700) -> (x/y=w2698:dbl)
        n1313 = case shown="False" w2754 {
          tunnel: w2753 -> [w2783 w2784]
          tunnel: [w2782 w2784] -> w2751
          frame False {
            n1314 = Negate(x=w2783) -> (-x=w2782:dbl[][])
          }
          frame True {
          }
        }
        n1315 = case shown="False" w2745 {
          tunnel: w2735 -> [w2780 w2781]
          tunnel: [w2779 w2781] -> w2734
          frame False {
            n1316 = Negate(x=w2780) -> (-x=w2779:dbl[][])
          }
          frame True {
          }
        }
        n1317 = Unbundle By Name(w2750) -> ("Peak%"=w2729:dbl)
        n1318 = Select(t=w2698, s=w2699, f=0.0) -> (s? t:f=w2696:dbl)
        n1319 = Array Subset(array=w2751, length (row)=w2752) -> (w2724:dbl[][])  [unwired: 3 in]
        n1320 = Array Subset(array=w2751, index (row)=w2752, length (row)=w2752) -> (w2723:dbl[][])  [unwired: 2 in]
        n1321 = Index Array ("Stimulus")(array=w2734, index (row) #1=1 ("index (row)"), index (row) #2=4 ("index (row)")) -> (element #1=w2731:dbl[], element #2=w2730:dbl[])  [unwired: 2 in]
        n1322 = Array Max & Min(array=w2731) -> (max value=w2727:dbl)  [unwired: 3 out]
        n1323 = Array Max & Min(array=w2730) -> (max value=w2725:dbl)  [unwired: 3 out]
        n1324 = Divide(x=w2729, y=100.0) -> (x/y=w2726:dbl)
        n1325 = Multiply(x=w2726, y=w2727) -> (x*y=w2722:dbl)
        n1326 = Multiply(x=w2726, y=w2725) -> (x*y=w2721:dbl)
        n1327 = for {
          tunnel: w2724 -> [w2778] mode=indexing
          tunnel: w2723 -> [w2776] mode=indexing
          tunnel: w2722 -> [w2777]
          tunnel: w2721 -> [w2775]
          tunnel: w2700 -> [w2772]
          tunnel: w2719 -> [w2771]
          tunnel: w2718 -> [w2770]
          tunnel: [w2766] -> w2717 mode=indexing if=w2767
          tunnel: [w2769] -> w2715 mode=indexing if=w2767
          tunnel: [w2768] -> w2716 mode=indexing if=w2767
          tunnel: w2696 -> [w2765]
          tunnel: w2696 -> [w2764]
          # "Find onset in each trace and calc latency."
          n1328 = Threshold 1D Array(1:w2764, 2:w2777, 3:w2778) -> (0:w2774:dbl)
          n1329 = Threshold 1D Array(1:w2765, 2:w2775, 3:w2776) -> (0:w2773:dbl)
          n1330 = Multiply(x=w2774, y=w2772) -> (x*y=w2766:dbl)
          n1331 = Multiply(x=w2773, y=w2772) -> (x*y=w2768:dbl)
          n1332 = Subtract(x=w2768, y=w2766) -> (x-y=w2769:dbl)
          n1333 = In Range and Coerce(upper limit=w2771, x=w2769, lower limit=w2770) -> (In Range?=w2767:bool)  [unwired: 1 out]
        }
        n1334 = Build Array(w2717, w2716, w2715) -> (w2710:dbl[][])
        n1335 = Array Size(array=w2717) -> (size(s)=w2714:i32)
        n1336 = call <vilib>:"Std Deviation and Variance.vi"("X"=w2717) -> ("mean"=w2713:dbl)  [unwired: 1 in, 2 out]
        n1337 = call <vilib>:"Std Deviation and Variance.vi"("X"=w2716) -> ("mean"=w2712:dbl)  [unwired: 1 in, 2 out]
        n1338 = call <vilib>:"Std Deviation and Variance.vi"("X"=w2715) -> ("mean"=w2711:dbl)  [unwired: 1 in, 2 out]
        n1339 = Transpose 2D Array(2D array=w2710) -> (transposed array=w2707:dbl[][])
        n1340 = Bundle By Name(cluster=T14 {"Stimulus Onset (ms)"=0.0, "Response Onset (ms)"=0.0, "Latency (ms)"=0.0, "Num Impulses"=0.0} ("Impulse Latency Results"), "Num Impulses"=w2714, "Stimulus Onset (ms)"=w2713, "Response Onset (ms)"=w2712, "Latency (ms)"=w2711) -> (w2748:T14)
        n1341 = local write "Impulse Latency Results"(w2707) -> ()
        n1342 = local write "Impulse Latency Summary"(w2748) -> ()
      }
      frame "Save Impulse Latency To Excel" {
        # "Write a new record for each impulse rather than the usual mean & standard deviation"
        n1343 = local read "Impulse Direction"() -> (w2788:bool)
        n1344 = Unbundle By Name(w2794) -> ("Excel"=w2796:refnum<class "Excel.lvclass">, "filename"=w2790:string)
        n1345 = local read "Impulse Latency Results"() -> (w2792:dbl[][])
        n1346 = Select(t="POS", s=w2788, f="NEG") -> (s? t:f=w2785:string)
        n1347 = call <userlib>:"Open.vi"("Worksheet Name (Sheet1)"="Impulse Latency", "Excel in"=w2796) -> ("error out"=w2803:errorcluster, "Excel out"=w2804:refnum<class "Excel.lvclass">)  [unwired: 8 in]
        n1348 = Number To Fractional String(number=w2792) -> (F-format string=w2791:string[][])  [unwired: 3 in]
        n1349 = call <userlib>:"Write.vi"("error in (no error)"=w2803, "Cell (Append to next row)"=cluster{"Row":i32, "Col":i32} {"Row"=0, "Col"=0}, "Data"=string[] ["File", "Direction", "Stimulus Onset (ms)", "Response Onset (ms)", "Latency (ms)"], "Excel in"=w2804) -> ("error out"=w2799:errorcluster, "Excel out"=w2800:refnum<class "Excel.lvclass">)  [unwired: 5 in, 1 out]
        n1350 = for {
          tunnel: w2791 -> [w2810] mode=indexing
          tunnel: w2790 -> [w2812]
          tunnel: [w2811] -> w2789 mode=indexing
          tunnel: w2785 -> [w2809]
          n1351 = Build Array (concatenate)(w2812, w2809, w2810) -> (w2811:string[])
        }
        n1352 = call <userlib>:"Write.vi"("error in (no error)"=w2799, "Data"=w2789, "Excel in"=w2800) -> ("error out"=w2797:errorcluster, "Excel out"=w2798:refnum<class "Excel.lvclass">)  [unwired: 6 in, 1 out]
        n1353 = call <userlib>:"Save.vi"("error in (no error)"=w2797, "Excel in"=w2798) -> ("Excel out"=w2795:refnum<class "Excel.lvclass">)  [unwired: 7 in, 2 out]
        n1354 = Bundle By Name(cluster=w2794, "Excel"=w2795) -> (w2793:T1)
      }
    }
  }
  "Data OUT" <- w3
